vi "MacroGUI_MD.vi"() -> ()   [LabVIEW 2012]
doc: "SciScan 1.2 160622\nThis is the Macro User Interface which lets the user create a new macro, load an existing macro (from text file) and execute the macro (with feedback of execution)"
uses:
  Custom Controls and Typedefs/Available Operations Tree.ctl
  HFG/SubVIs/Master Slave messaging Flags.ctl
  HFG/Custom Controls and Typedefs/HB_Error Conditions Cluster.ctl
  HFG/Custom Controls and Typedefs/Heartbeat information cluster.ctl
  HFG/Custom Controls and Typedefs/Heartbeat Event Source.ctl
  Custom Controls/Heartbeat_States.ctl
  CommonResource VIs/Timing/Timing Indicator.ctl
  Custom Controls/Edit button with text.ctl
  Custom Controls and Typedefs/Timing Estimate Cluster.ctl
  Custom Controls and Typedefs/Confirm Settings.ctl
  Custom Controls and Typedefs/Delete Button.ctl
  Custom Controls and Typedefs/Cancel Settings.ctl
  Custom Controls and Typedefs/Load from PSM Button.ctl
  Custom Controls and Typedefs/Macro_MD_UI Control Refnums.ctl
  HFG/SubVIs/Heartbeat state manager Input VI names.ctl
  HFG/Custom Controls and Typedefs/HB Actionable Event.ctl
  CommonResource VIs/FormatTree&TableStyle_Commands.ctl
  <vilib>/Utility/miscctls.llb/LVRowAndColumnUnsignedTypeDef.ctl
  <vilib>/Utility/miscctls.llb/LVNodeAndColumnTypeDef.ctl
  Custom Controls and Typedefs/LOOP Control Cluster.ctl
  SubVIs/FGV_MacroCore_Commands.ctl
  CommonResource VIs/Timing/Timer Commands.ctl
  Common Macro VIs/Backup or Restore GFG Config Data_Commands.ctl
  HFG/Custom Controls and Typedefs/HFG Commands.ctl
  SubVIs/Update Scan Settings_Commands.ctl
  CommonResource VIs/UI Control and Indicator properties_Commands.ctl
  CommonResource VIs/Enable-Disable SCISCAN controls_Command.ctl
  Macro Rule/subVIs/MacroErrorsFGV_Commands.ctl
  image & display/Draw ROI on Line Scan Display Command.ctl
  SubVIs/MacroFileIO_Commands.ctl
  Macro Loop Manager Module/SubVIs/Macro Execution and Timing_Commands.ctl
  Custom Controls/scan mode main settings tab.ctl
  SubVIs/SCISCAN Image display to Enum_Commands.ctl
  GFG/GFG library.lvlib
  Custom Controls/Setting File Types.ctl
panel:
  in  "Refresh Timing":bool
  in  "Copy Button":bool
  in  "Get Positions":T1
  in  "Cancel Settings":T2
  in  "Delete Button":T3
  in  "Preview Macro":bool
  in  "Preview Cluster":T4
  in  "Edit Parameters":T5
  out "MacroFile\nPath":path caption="MacroFile\nPath*"
  in  "Confirm Settings":T6
  in  "Select Display":u16(ring) items=["Channel 1", "Channel 2", "Channel 3", "Channel 4", "all channels", "RGB overlay", "ROI", "arbitrary line scan"]
  out "Timing\n(approx.)":T7 caption="Timing\n(approx.)*" {"Elapsed" format="%<%H:%M:%S>t"; "Progress" scale=0.0..100.0; "Remaining" format="%<%H:%M:%S>t"; "Est. Time" format="%<%H:%M:%S>t"}
  out "Macro Error?":bool
  in  "Info":string[][](table)
  out "Paused/Wait for Trig":T8 caption="Paused" {"Elapsed" format="%<%H:%M:%S>t"; "Progress" scale=0.0..100.0; "Seconds" scale=0.0..60.0; "Remaining" format="%<%H:%M:%S>t"; "Set Time" format="%<%H:%M:%S>t"}
  out "Slave Completions Received":i32
  in  "stop 2":bool
  out "Master instr received":i32
  out "Slave conf received":i32
  out "Heartbeat information cluster":T9
  out "Error conditions Cluster":T12
  out "Master-Slave messaging Flags":T13={"Instruction available"=TRUE, "Slave action completed"=TRUE, "Slave Ready?"=FALSE}
  out "Current Index":i32
  in  "MacroTreeOperation":cluster{"Save Button":bool}
  in  "File Operation Cluster":T14
  in  "Parameters":string[][](table)
  in  "Execute Macro":bool
  in  "Available Actions":T15
  in  "Macro":string(tree)
  # "(hh:mm:ss)"
  # "(hh:mm:ss)"
  # "(hh:mm:ss)"
  # "(hh:mm:ss)"
  # "(hh:mm:ss)"
  # "(hh:mm:ss)"
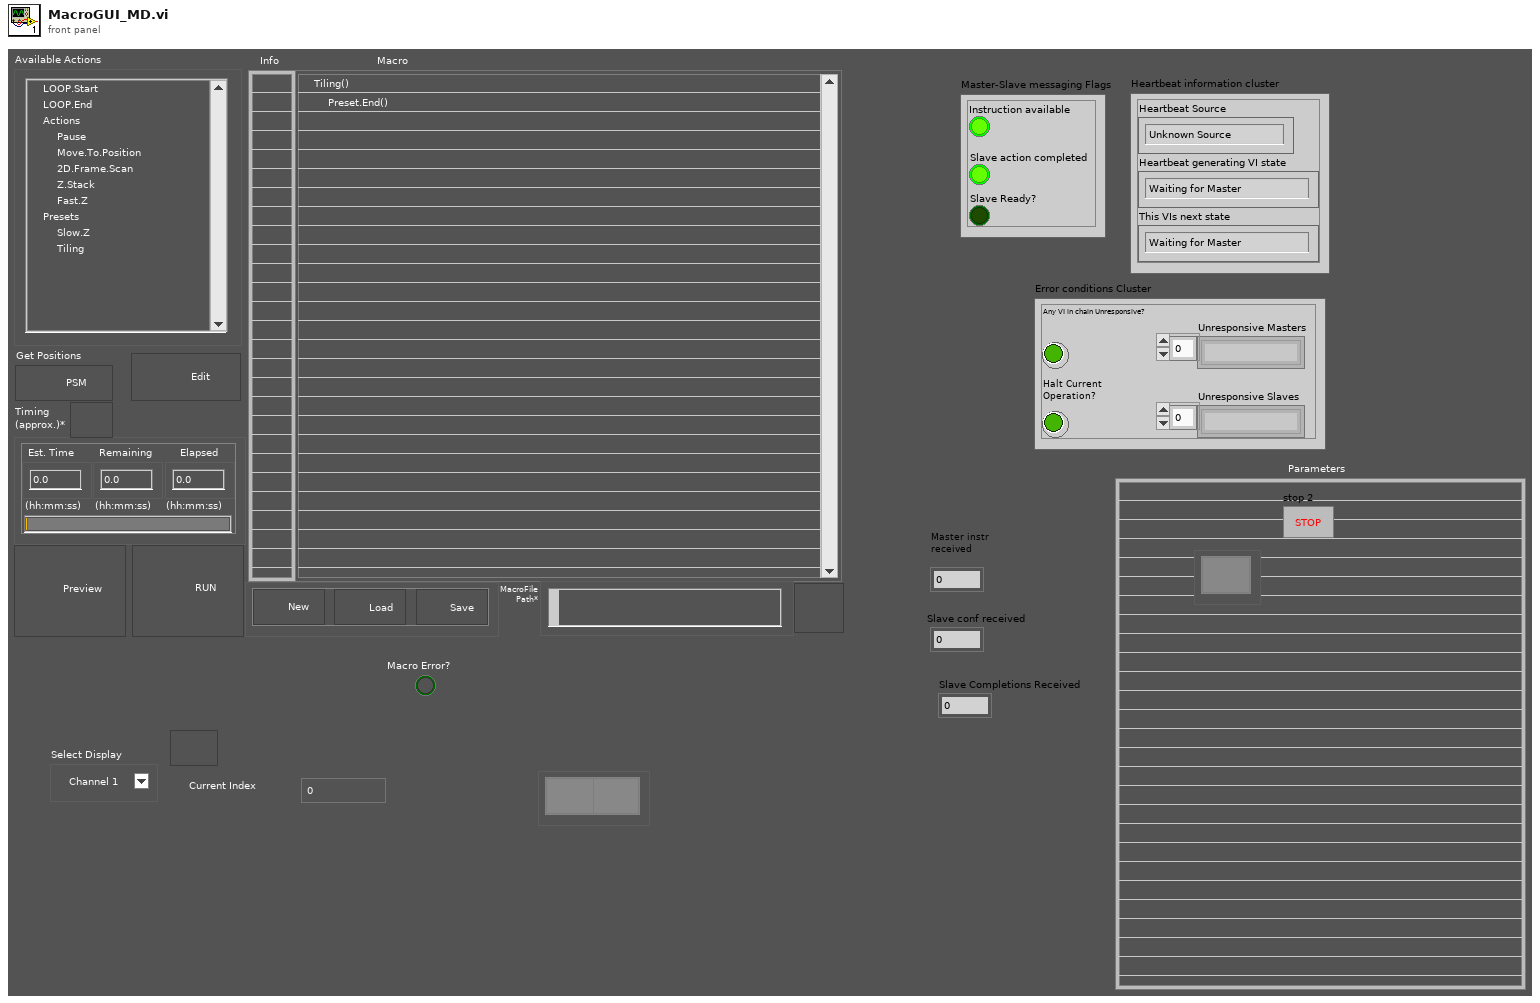
[diagram p1: front panel]
types:
  T1 = typedef "Load from PSM Button.ctl" = bool
  T2 = typedef "Cancel Settings.ctl" = bool
  T3 = typedef "Delete Button.ctl" = bool
  T4 = cluster{"Skip Forward Macro":bool, "Skip Back Macro":bool}
  T5 = typedef "Edit button with text.ctl" = bool
  T6 = typedef "Confirm Settings.ctl" = bool
  T7 = typedef "Timing Estimate Cluster.ctl" = cluster{"Est. Time":dbl, "Remaining":dbl, "Progress":u8, "Elapsed":dbl}
  T8 = typedef "Timing Indicator.ctl" = cluster{"Set Time":dbl, "Remaining":dbl, "Seconds":dbl, "Progress":u8, "Elapsed":dbl}
  T9 = typedef "Heartbeat information cluster.ctl" = cluster{"Heartbeat Source":T10, "Heartbeat generating VI state":T11, "This VIs next state":T11}
  T10 = typedef "Heartbeat Event Source.ctl" = enum16{"Unknown Source", "Timeout", "This VI", "Master", "Slave"}
  T11 = typedef "Heartbeat_States.ctl" = enum16{"Waiting for Master", "Instruction Issued", "Waiting for Slave Completion", "Completed", "Cancelled", "Failed", "Broken Link"}
  T12 = typedef "HB_Error Conditions Cluster.ctl" = cluster{"Any VI in chain Unresponsive?":bool, "Halt Current Operation?":bool, "Unresponsive Masters":string[], "Unresponsive Slaves":string[]}
  T13 = typedef "Master Slave messaging Flags.ctl" = cluster{"Instruction available":bool, "Slave action completed":bool, "Slave Ready?":bool}
  T14 = cluster{"Load Macro":bool, "Save Macro":bool, "New Macro":bool}
  T15 = typedef "Available Operations Tree.ctl" = string
  T16 = typedef "HB Actionable Event.ctl" = enum16{"Master instruction event", "Slave ready event", "Slave unavailable event", "Cancelled or Failed event", "Slave action complete event", "QUIT", "Broken Link", "Recovered from Broken Link"}
  T17 = typedef "Heartbeat state manager Input VI names.ctl" = cluster{"Current VI name":string, "Master VI Names":string[], "Slave VI Names":string[]}
  T18 = typedef "Macro_MD_UI Control Refnums.ctl" = cluster{"Avail. Operations":refnum<vi>, "Created Macro":refnum<vi>, "Load Macro":refnum<vi>, "Save Macro":refnum<vi>, "Params Table":refnum<vi>, "Delete":refnum<vi>, "Edit Button":refnum<vi>, "Execute Macro":refnum<vi>, "Info Tbl":refnum<vi>, "Execution Timing":refnum<vi>, "Select Display":refnum<vi>, "File Ops Cluster":refnum<vi>, "Paused/Waiting Trig":refnum<vi>, "Confirm":refnum<vi>, "New Macro":refnum<vi>, "Preview Macro":refnum<vi>, "Skip Forward":refnum<vi>, "Skip Back":refnum<vi>, "Macro File Path":refnum<vi>, "Main GUI Reference":refnum<vi>, "Cancel Settings":refnum<vi>, "Get Positions":refnum<vi>, "Copy":refnum<vi>, "Refresh Timing":refnum<vi>}
  T19 = typedef "LVRowAndColumnUnsignedTypeDef.ctl" = cluster{"Row":u32, "Column":u32}
  T20 = cluster{"user event out":refnum<user-event>, "HB Actionable Event":refnum<user-event>, "Index Values":refnum<user-event>, "Macro":refnum<vi>, "Parameters":refnum<vi>}
  T21 = typedef "Timer Commands.ctl" = enum16{"Clear All", "Start", "Pause", "Check Time"}
  T22 = typedef "FormatTree&TableStyle_Commands.ctl" = enum16{"Colour Row", "Uncolour Row", "Bold Row", "Unbold Row", "Clear", "UpdateVisibleRows"}
  T23 = typedef "LVNodeAndColumnTypeDef.ctl" = cluster{"Node":string, "Column":i32}
  T24 = typedef "FGV_MacroCore_Commands.ctl" = enum16{"Initialize", "Get Array", "Load macro from file", "Insert Item", "Insert at End", "Edit Parameter String", "Delete instruction", "Move Items", "Save", "SaveAs", "UpdateInfoTable", "Edit Settings File", "New Macro", "Read Temp File", "Delete Multiple"}
  T25 = enum16{"None", "Stacked", "Clockwise", "Counterclockwise"}
  T26 = typedef "SCISCAN Image display to Enum_Commands.ctl" = enum16{"Initialize", "SCISCAN disp to Enum", "Enum to SCISCAN disp"}
  T27 = typedef "Backup or Restore GFG Config Data_Commands.ctl" = enum16{"Backup", "Restore"}
  T28 = typedef "UI Control and Indicator properties_Commands.ctl" = enum16{"Enable", "Disable", "Disable and Grey", "Make Visible", "Make Invisible"}
  T29 = typedef "Update Scan Settings_Commands.ctl" = enum16{"Initiate Update", "Finalise Update"}
  T30 = typedef "HFG Commands.ctl" = enum16{"Set", "Get", "Initialize"}
  T31 = typedef "Enable-Disable SCISCAN controls_Command.ctl" = enum16{"Enable the items disabled earlier", "Disable", "Disable and Gray", "Enable all (except those in skip list)"}
  T32 = enum8{"Enabled", "Disabled", "Disabled and Grayed Out"}
  T33 = enum16{"Available Operations Tree", "Macro Tree"}
  T34 = typedef "MacroErrorsFGV_Commands.ctl" = enum16{"Initialize", "Get Error Array", "Set Error Array"}
  T35 = typedef "Draw ROI on Line Scan Display Command.ctl" = enum16{"Draw ROI from GFG", "Clear ROI"}
  T36 = typedef "Macro Execution and Timing_Commands.ctl" = enum16{"Initialize (Update FGV & Rst Idx)", "Run", "EstimateTime", "Preview", "Update Macro array (Idx Unchanged)", "Update Index", "Clear Timing Info"}
  T37 = typedef "MacroFileIO_Commands.ctl" = enum16{"Get Macro Info", "Initialize", "New Macro", "Load Macro", "Save", "Save in today's folder", "Update Settings File", "Add Settings File", "Delete Settings File", "Update Macro Text", "Save As", "Read Temp File"}
  T38 = enum32{"Invalid", "Standard", "Closed", "Hidden", "Minimized", "Maximized"}
  T39 = typedef "Setting File Types.ctl" = enum16{"2D.Frame.Scan.Settings", "2D.Line.Scan.Settings", "Z.Stack.Settings", "HW Settings", "Configuration Settings", "Unknown Settings", "Fast.Z.Settings"}
  T40 = typedef "scan mode main settings tab.ctl" = enum32{"2D frame", "2D line scan", "general settings", "Z Stack", "piezo"}
  T41 = typedef "LOOP Control Cluster.ctl" = cluster{"Index of LOOP.Start":i32, "Iteration Count Down":i32, "No of iterations (N)":i32}
  T42 = cluster{"Estimated Run time":dbl, "Step by step exec time":dbl[]}
  T43 = typedef "eventvkey.ctl" = enum16{"ASCII", "Enter", "Return", "Shift", "Ctrl", "Alt", "Cmd", "Opt", "Caps", "NumLock", "Clear", "Break", "Up", "Down", "Left", "Right", "Insert", "Delete", "Home", "End", "PageUp", "PageDown", "Escape", "Help", "Pause", "ScrollLock", "F1", "F2", "F3", "F4", "F5", "F6", "F7", "F8", "F9", "F10", "F11", "F12", "F13", "F14", "F15", "F16", "F17", "F18", "F19", "F20", "F21", "F22", "F23", "F24", "Play", "VolumeUp", "VolumeDown", "Mute", "Two Byte Char"}
  T44 = cluster{"data name":string, "drag data":variant}[]
  T45 = typedef "LVPoint32TypeDef.ctl" = cluster{"Horizontal":i32, "Vertical":i32}
  T46 = typedef "LVRowAndColumnTypeDef.ctl" = cluster{"Row":i32, "Column":i32}
  T47 = typedef "Macro Error Cluster.ctl" = cluster{"Error?":bool, "Description":string, "Warning?":bool}
  T48 = typedef "File Operation Status.ctl" = enum16{"Success", "File does not exist", "Cancelled by User", "Incorrect extension type"}
  T49 = typedef "Macro_Action_List.ctl" = enum16{"Unknown Command", "2D.Frame.Scan", "2D.Line.Scan", "Load.Settings.File", "Move.To.Position", "Pause", "Z.Stack", "LOOP.Start", "LOOP.End", "Record", "Fast.Z", "Generic", "Slow.Z", "Tiling", "Preset.End"}
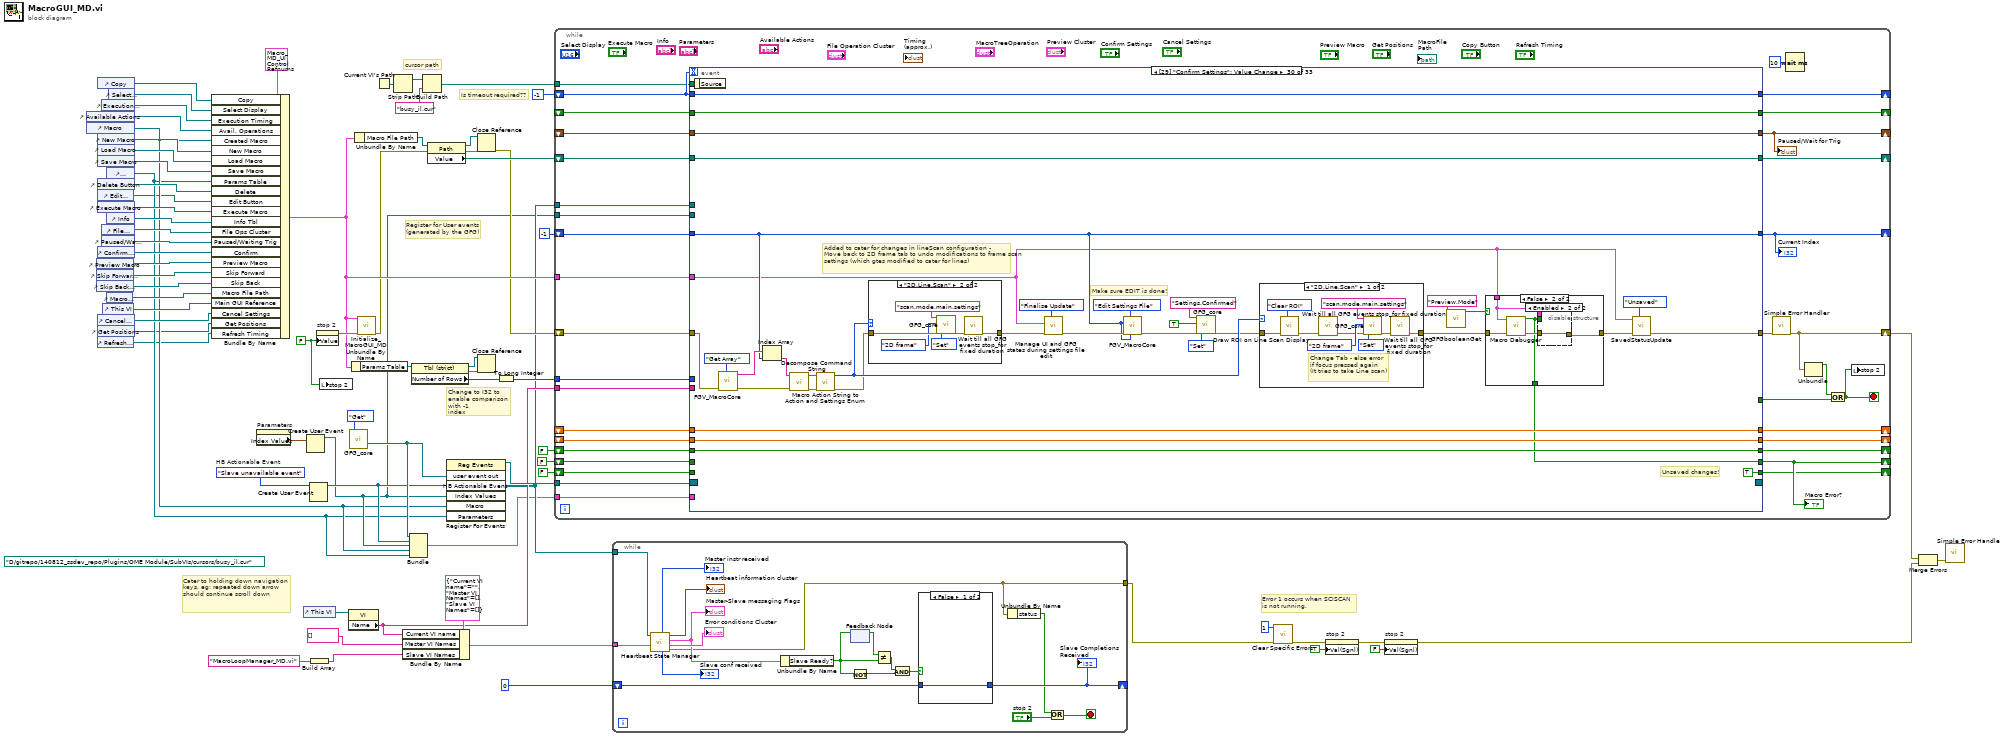
[diagram p0: block diagram]
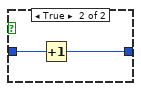
[diagram p2: hidden frame]
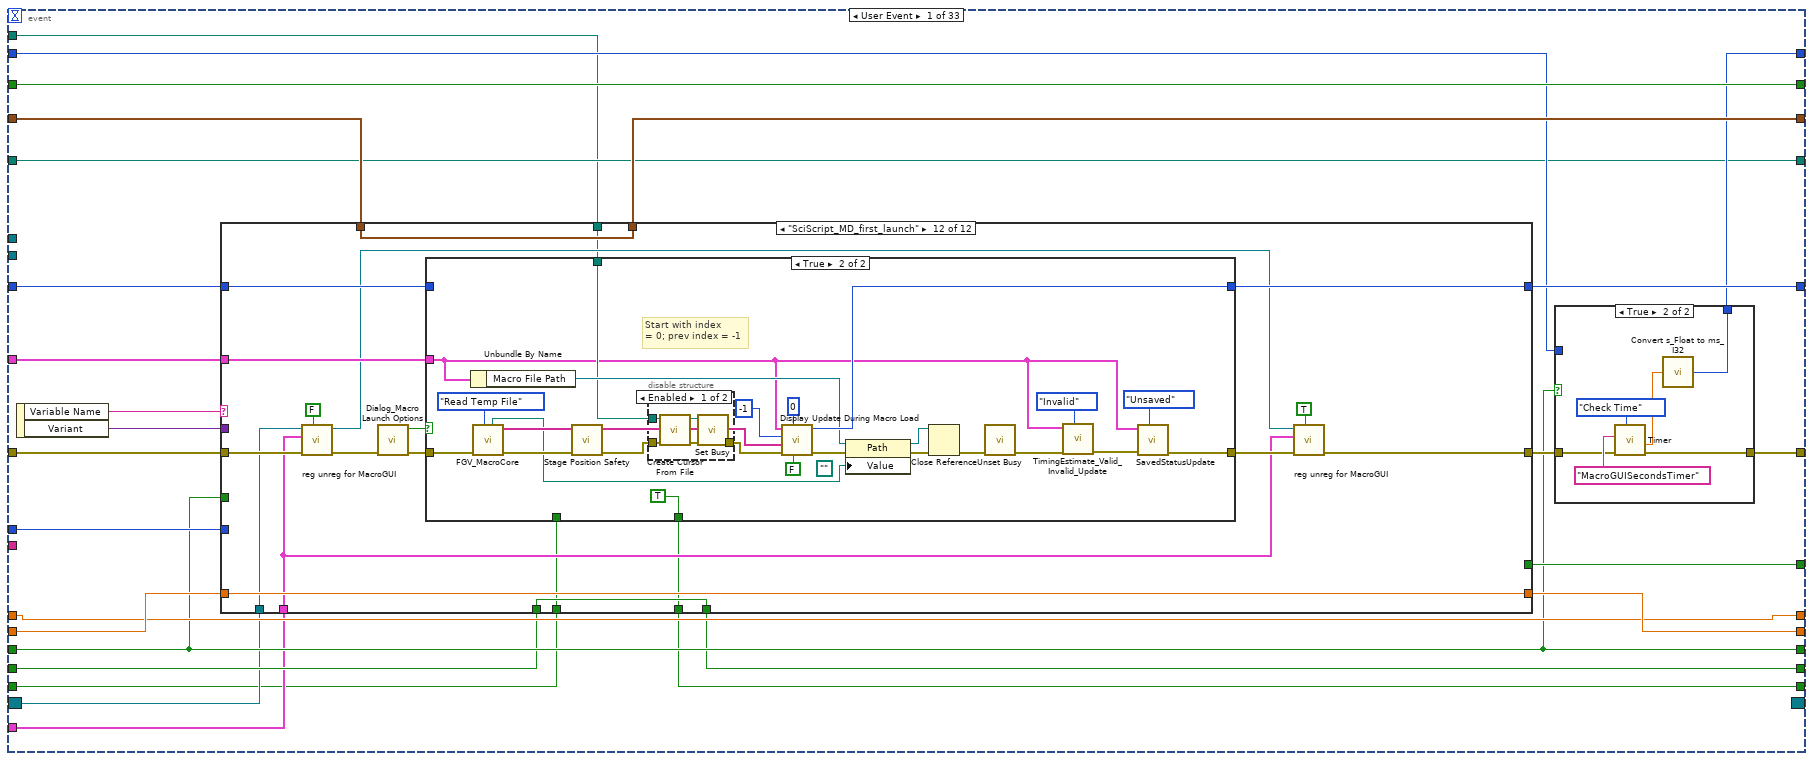
[diagram p3: hidden frame]
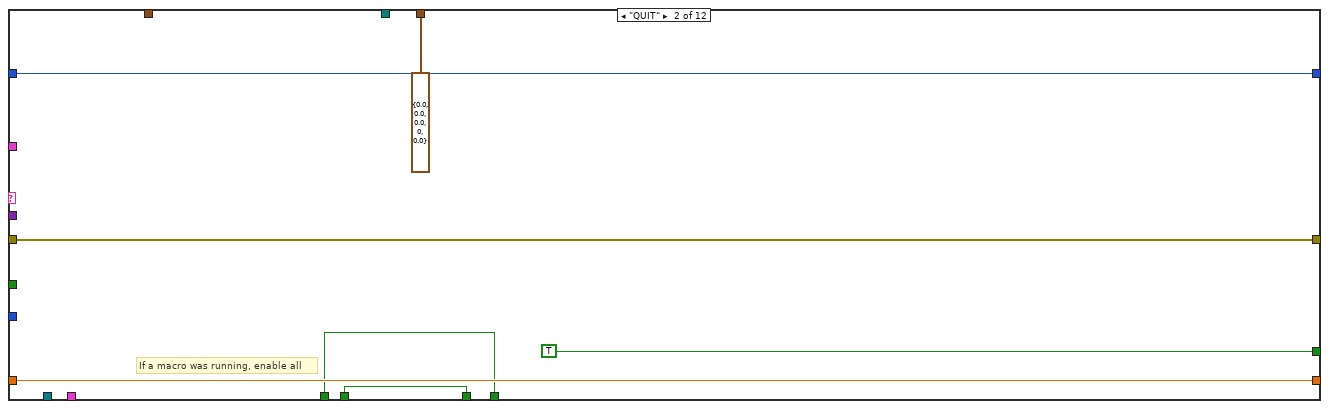
[diagram p6: hidden frame]
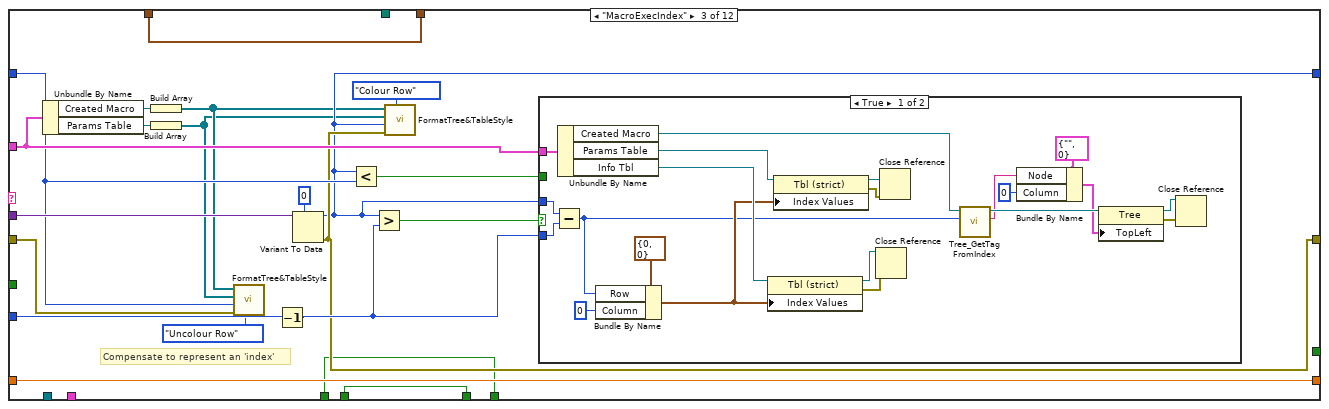
[diagram p7: hidden frame]
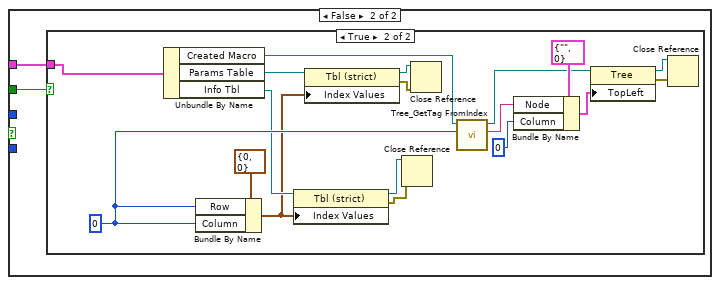
[diagram p8: hidden frame]
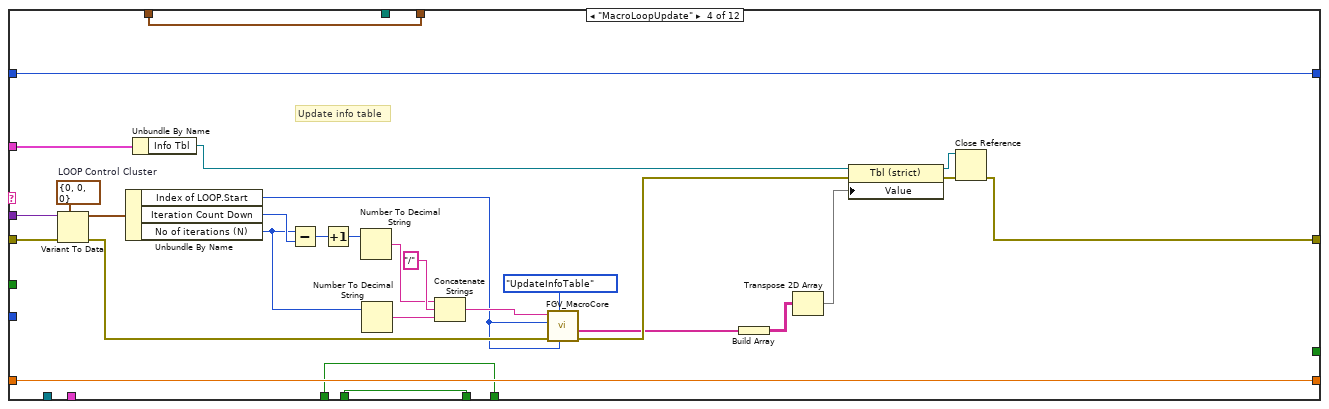
[diagram p10: hidden frame]
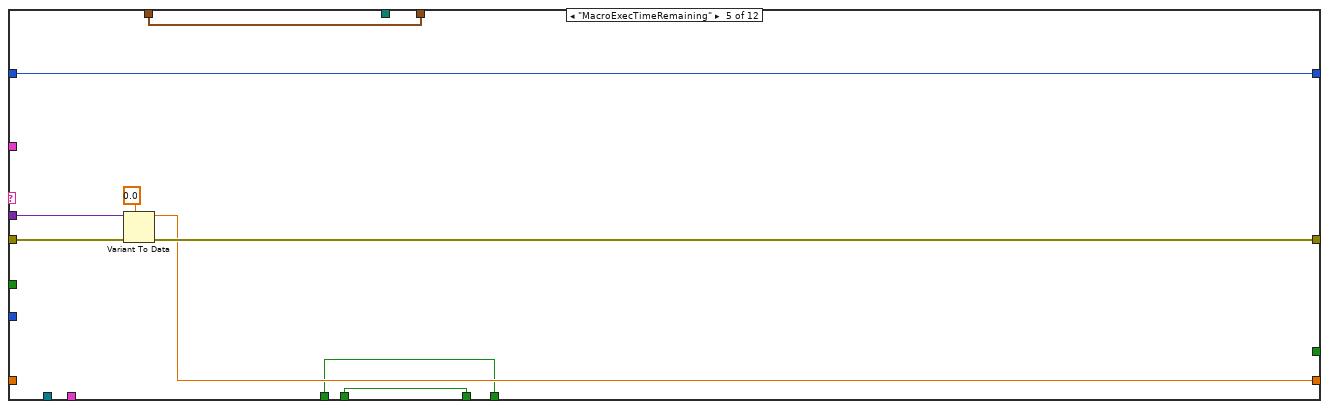
[diagram p11: hidden frame]
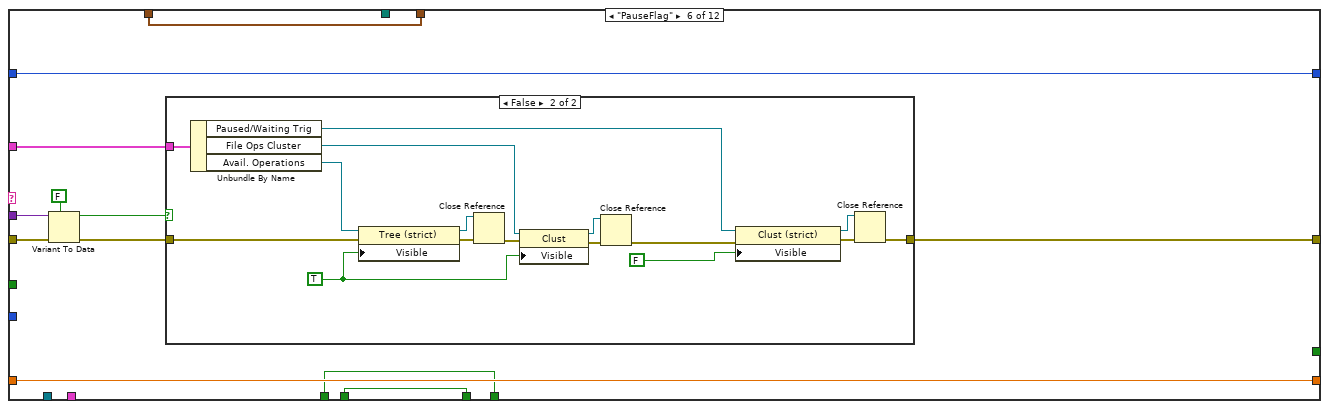
[diagram p12: hidden frame]
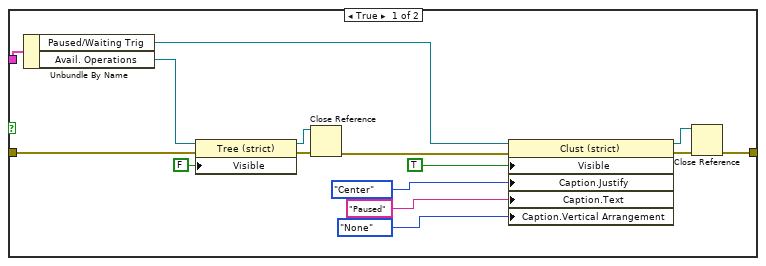
[diagram p13: hidden frame]
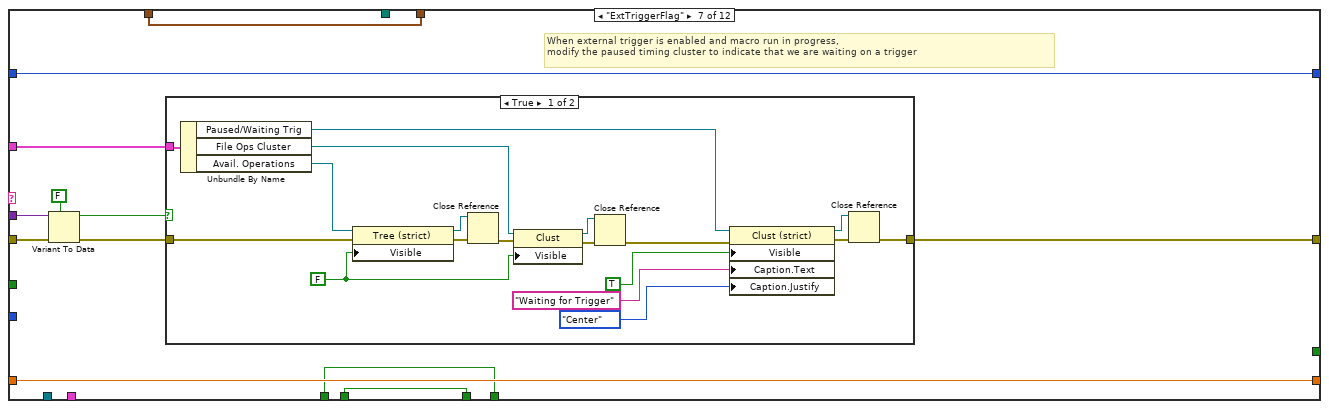
[diagram p14: hidden frame]
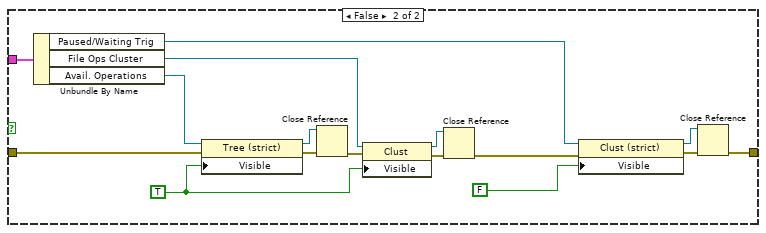
[diagram p15: hidden frame]
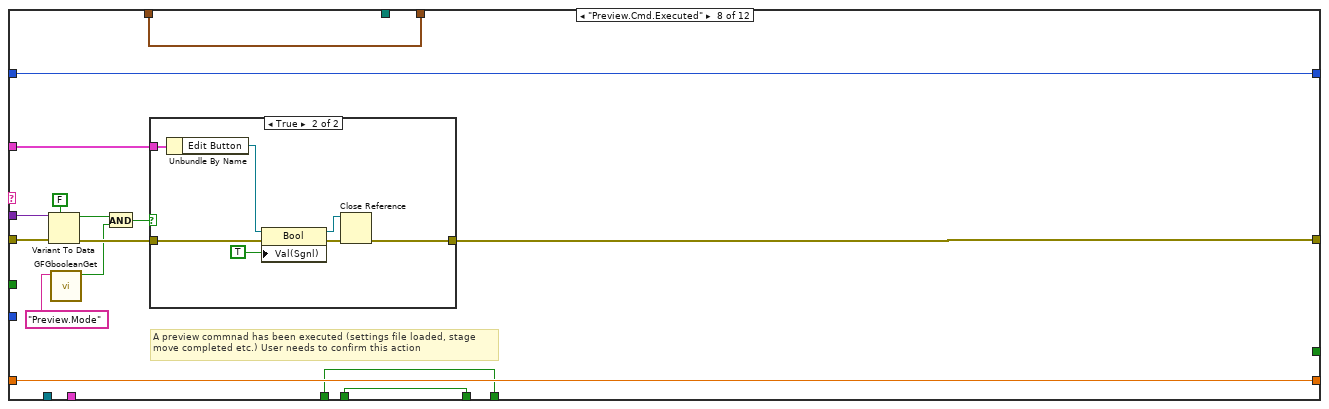
[diagram p16: hidden frame]
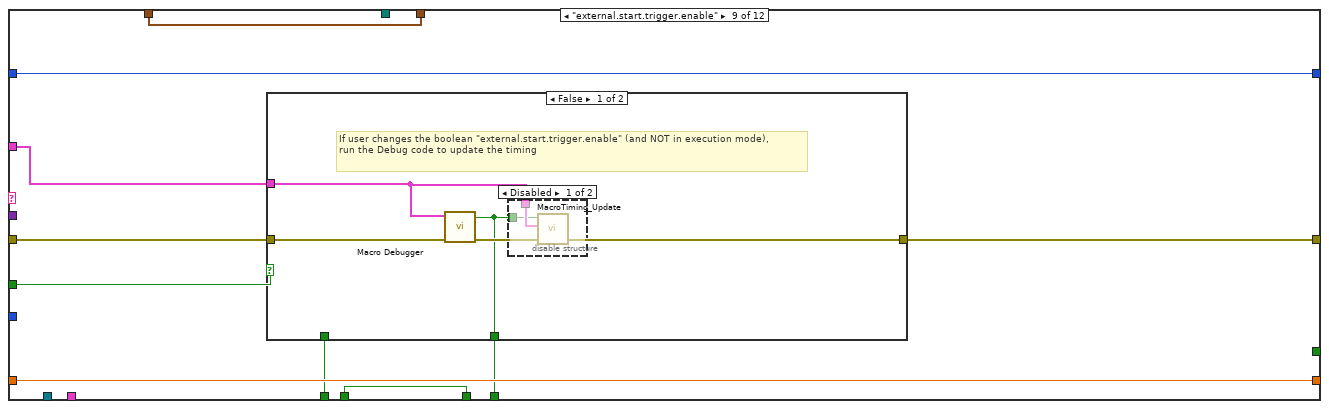
[diagram p18: hidden frame]
diagram:
  (unwired) path "D:/gitrepo/140812_ssdev_repo/Plugins/OME Module/SubVIs/cursors/busy_il.cur" ("cursor file")
  w65 = HB_Actionable_Event."Slave unavailable event"  # HB Actionable Event
  w51 = FALSE ("Execute Macro")
  # "cursor path"
  # "Cater to holding down navigation keys. eg: repeated down arrow should continue scroll down"
  # "Change to I32 to\nenable comparison with -1\nindex"
  # "Error 1 occurs when SCISCAN\nis not running."
  # "Is timeout required??"
  # "Register for User events\n(generated by the GFG)"
  n1 = control-ref of="Available Actions"() -> (w71:refnum<vi>)
  n2 = control-ref of="Macro"() -> (w13:refnum<vi>)
  n3 = control-ref of="Preview Macro"() -> (w33:refnum<vi>)
  n4 = control-ref of="Skip Forward Macro"() -> (w32:refnum<vi>)
  n5 = control-ref of="Skip Back Macro"() -> (w31:refnum<vi>)
  n6 = control-ref of="Edit Parameters"() -> (w2:refnum<vi>)
  n7 = control-ref of="Refresh Timing"() -> (w1:refnum<vi>)
  n8 = control-ref of="Copy"() -> (w7:refnum<vi>)
  n9 = control-ref of="New Macro"() -> (w34:refnum<vi>)
  n10 = control-ref of="Load Macro"() -> (w36:refnum<vi>)
  n11 = control-ref of="Save Macro"() -> (w72:refnum<vi>)
  n12 = control-ref of="Delete Button"() -> (w50:refnum<vi>)
  n13 = control-ref of="Execute Macro"() -> (w35:refnum<vi>)
  n14 = control-ref of="Confirm Settings"() -> (w37:refnum<vi>)
  n15 = control-ref of="Cancel Settings"() -> (w19:refnum<vi>)
  n16 = control-ref of="Get Positions"() -> (w10:refnum<vi>)
  n17 = control-ref of="Execution Timing"() -> (w42:refnum<vi>)
  n18 = control-ref of="File Operation Cluster"() -> (w40:refnum<vi>)
  n19 = control-ref of="Paused/Wait for Trig"() -> (w39:refnum<vi>)
  n20 = control-ref of="This VI"() -> (w20:refnum<vi>)
  n21 = control-ref of="Parameters"() -> (w12:refnum<vi>)
  n22 = control-ref of="Info"() -> (w45:refnum<vi>)
  n23 = control-ref of="Macro File Path"() -> (w30:refnum<vi>)
  n24 = control-ref of="Select Display"() -> (w41:refnum<vi>)
  n25 = Bundle By Name(cluster=T18 {"Avail. Operations"=refnum, "Created Macro"=refnum, "Load Macro"=refnum, "Save Macro"=refnum, "Params Table"=refnum, "Delete"=refnum, "Edit Button"=refnum, "Execute Macro"=refnum, "Info Tbl"=refnum, "Execution Timing"=refnum, "Select Display"=refnum, "File Ops Cluster"=refnum, "Paused/Waiting Trig"=refnum, "Confirm"=refnum, "New Macro"=refnum, "Preview Macro"=refnum, "Skip Forward"=refnum, "Skip Back"=refnum, "Macro File Path"=refnum, "Main GUI Reference"=refnum, "Cancel Settings"=refnum, "Get Positions"=refnum, "Copy"=refnum, "Refresh Timing"=refnum} ("UI control refnums"), "Copy"=w7, "Select Display"=w41, "Execution Timing"=w42, "Avail. Operations"=w71, "Created Macro"=w13, "New Macro"=w34, "Load Macro"=w36, "Save Macro"=w72, "Params Table"=w12, "Delete"=w50, "Edit Button"=w2, "Execute Macro"=w35, "Info Tbl"=w45, "File Ops Cluster"=w40, "Paused/Waiting Trig"=w39, "Confirm"=w37, "Preview Macro"=w33, "Skip Forward"=w32, "Skip Back"=w31, "Macro File Path"=w30, "Main GUI Reference"=w20, "Cancel Settings"=w19, "Get Positions"=w10, "Refresh Timing"=w1) -> (w29:T18)
  n26 = property on="Parameters" class="Tbl (strict)"() -> ("Index Values"=w49:T19)  [unwired: 2 in, 2 out]
  n27 = control-ref of="This VI"() -> (w67:refnum<vi>)
  n28 = Create User Event(user event datatype=w49) -> (user event=w14:refnum<user-event>)  [unwired: 1 in, 1 out]
  n29 = Create User Event(user event datatype=w65) -> (user event=w15:refnum<user-event>)  [unwired: 1 in, 1 out]
  n30 = Build Array("MacroLoopManager_MD.vi") -> (w22:string[])
  n31 = property on="stop 2" class="Bool (strict)"("Value"=w51) -> (error out=w38:errorcluster)  [unwired: 2 in, 1 out]
  n32 = local write "stop 2"(w51) -> ()
  n33 = property class="VI"(reference=w67) -> ("Name"=w64:string)  [unwired: 1 in, 2 out]
  n34 = call "GFG_core.vi"("Action"=enum16{"Init", "Set", "Get", "Clear"}."Get") -> ("user event out"=w16:refnum<user-event>)  [unwired: 12 in, 6 out]
  n35 = Unbundle By Name(w29) -> ("Params Table"=w46:refnum<vi>)
  n36 = Unbundle By Name(w29) -> ("Macro File Path"=w28:refnum<vi>)
  n37 = call "Initialize_MacroGUI_MD.vi"("Error In"=w38, "UI control refnums"=w29) -> ("Error Out"=w25:errorcluster)  [unwired: 7 in, 2 out]
  n38 = Current VI's Path() -> (path=w6:path)
  n39 = Strip Path(path=w6) -> (stripped path=w5:path)  [unwired: 1 out]
  n40 = Bundle By Name(cluster=T17 {"Current VI name"="", "Master VI Names"=[], "Slave VI Names"=[]} ("Heartbeat state manager Input VI names 2"), "Current VI name"=w64, "Master VI Names"=string[] [], "Slave VI Names"=w22) -> (w66:T17)
  n41 = Bundle("user event out"=w16, "HB Actionable Event"=w15, "Index Values"=w14, "Macro"=w13, "Parameters"=w12) -> (w11:T20)  [unwired: 1 in]
  n42 = property class="Tbl (strict)"(reference=w46) -> (reference out=w47:refnum<vi>, error out=w48:errorcluster, "Number of Rows"=w44:u32)  [unwired: 1 in]
  n43 = Build Path(base path=w5, name or relative path="busy_il.cur") -> (appended path=w3:path)
  n44 = property class="Path"(reference=w28, error in=w25) -> (reference out=w26:refnum<vi>, error out=w27:errorcluster, "Value"=w24:path)
  n45 = register-events(w16, w15, w14, w13, w12) -> (reference out=w70:refnum<event-registration>)  [unwired: 2 in, 1 out]
  n46 = Close Reference(reference=w26, error in (no error)=w27) -> (error out=w21:errorcluster)
  n47 = Close Reference(reference=w47, error in (no error)=w48) -> ()  [unwired: 1 out]
  n48 = To Long Integer(number=w44) -> (32bit integer=w43:i32)
  n49 = while {
    tunnel: w29 -> [w104]
    shift-right: [w80] -> w59
    shift-left: w21 -> [w89]
    shift-right: [w105] -> _
    shift-left: -1 ("New Index OUT") -> [w103]
    tunnel: w70 -> [w86]
    shift-right: [w102] -> _
    shift-left: -1 ("Index") -> [w101]
    tunnel: w64 -> [w100]
    shift-right: [w99] -> _
    shift-left: FALSE -> [w98]
    shift-right: [w97] -> _
    shift-left: _ -> [w96]
    shift-right: [w95] -> _
    shift-left: _ -> [w94]
    tunnel: w43 -> [w90]
    shift-right: [w92] -> _
    shift-left: FALSE ("Any Error?") -> [w91]
    shift-right: [w88] -> _
    shift-left: _ -> [w87]
    shift-right: [w85] -> _
    shift-left: _ -> [w84]
    shift-right: [w82] -> _
    shift-left: w24 -> [w83]
    tunnel: w15 -> [w79]
    tunnel: w14 -> [w78]
    tunnel: w11 -> [w77]
    shift-right: [w75] -> _
    shift-left: FALSE ("Any Error?") -> [w76]
    tunnel: w3 -> [w74]
    stop <- w93 stop-if-true
    n50 = event shown="[29] \"Confirm Settings\": Value Change" {
      selector: w86 -> [w112 _ _ _ _ _ _ _ _ _ _ _ _ _ w1038 w1064 _ _ _ _ _ _ _ w1619 w1652 _ _ w1859 _ _ w2253 _ _]
      dyn-events: [_ _ _ _ _ _ _ _ _ _ _ _ _ _ w1035 w1062 _ _ _ _ _ _ _ w1613 w1651 _ _ w1852 _ _ w2247 _ _] -> _
      timeout: w101 -> [_ _ _ _ _ _ _ _ _ _ _ _ _ _ _ _ _ _ _ _ _ _ _ _ _ _ _ _ _ _ _ _ _]
      tunnel: [w132 _ _ _ _ _ _ _ _ _ _ _ _ _ _ _ _ _ _ _ _ _ _ _ _ _ _ _ _ _ _ _ w2355] -> w108
      tunnel: w104 -> [w125 w481 _ w627 _ _ w805 w826 w846 w935 _ _ w1002 _ w1058 w1068 _ w1133 _ w1358 w1431 w1504 w1558 w1628 w1656 w1768 w1823 w1846 w2154 w2181 w2244 w2325 _]
      tunnel: w89 -> [w133 w482 w609 w629 w764 w793 w804 w844 w851 w930 w964 w976 w997 w1033 w1044 w1072 w1118 w1138 w1333 w1359 w1427 w1510 w1556 w1620 w1660 w1772 w1802 w1857 w2159 w2177 w2242 w2330 w2359]
      tunnel: [w121 w473 w608 w628 w764 w793 w811 w844 w853 w933 w964 w976 w994 w1033 w1039 w1081 w1114 w1139 w1332 w1357 w1428 w1511 w1560 w1612 w1658 w1769 w1797 w1853 w2158 w2183 w2246 w2316 w2359] -> w81
      tunnel: [w130 w485 w615 w625 w763 w792 w803 w843 w881 w928 w963 w975 w999 w1032 w1059 w1070 w1125 w1140 w1336 w1344 w1424 w1506 w1568 w1636 w1654 w1781 w1819 w1860 w2173 w2182 w2243 w2319 w2358] -> w105
      tunnel: w103 -> [w131 w485 w615 w626 w763 w792 w803 w843 w871 w927 w963 w975 w1000 w1032 w1059 w1069 w1125 w1140 w1336 w1344 w1426 w1505 w1568 w1636 w1655 w1781 w1820 w1842 w2173 w2182 w2240 w2319 w2358]
      tunnel: [w122 w475 w614 w634 w762 w779 w802 w836 w867 100 ("Index") -1 ("Index") w974 w981 -1 ("Index") w1053 w1094 w1124 w1130 w1335 w1354 w1438 w1509 w1567 w1635 w1668 w1780 w1815 w1869 w2172 w2208 w2266 w2337 w2357] -> w102
      tunnel: w101 -> [w123 w476 w614 w634 w762 w779 w802 w836 w867 _ _ w974 w981 _ w1053 w1094 w1124 _ w1335 w1347 w1438 w1509 w1567 w1635 w1668 w1780 w1815 w1869 w2172 w2208 w2266 w2337 w2357]
      tunnel: w100 -> [_ w480 _ _ _ _ _ _ _ _ _ _ _ _ _ _ _ w1136 _ _ _ _ _ _ w1659 _ _ _ _ _ _ _ _]
      tunnel: [w117 w477 w613 w624 w761 w778 w801 w835 w864 w924 w962 w973 w991 w1031 w1052 w1093 w1123 w1135 w1330 w1355 w1437 w1508 w1566 w1634 w1667 w1779 w1814 w1868 w2171 w2207 w2265 w2336 w2356] -> w99
      tunnel: w98 -> [w117 w483 w613 w624 w761 w778 w801 w835 w864 w924 w962 w973 w991 w1031 w1052 w1093 w1123 _ w1330 w1355 w1437 w1508 w1566 w1634 w1667 w1779 w1814 w1868 w2171 w2207 w2265 w2336 w2356]
      tunnel: [w129 w479 w612 w633 w760 w777 w800 w834 w866 w919 w961 w972 w990 w1030 w1051 w1092 w1122 w1134 w1331 w1360 w1436 w1503 w1565 w1633 w1666 w1778 w1813 w1867 w2170 w2206 w2264 w2335 w2354] -> w97
      tunnel: w96 -> [w128 w479 w612 w633 w760 w777 w800 w834 w866 w919 w961 w972 w990 w1030 w1051 w1092 w1122 w1134 w1331 w1360 w1436 w1503 w1565 w1633 w1666 w1778 w1813 w1867 w2170 w2206 w2264 w2335 w2354]
      tunnel: [w127 w478 w611 w632 w759 w776 w799 w833 w865 TRUE FALSE w971 FALSE FALSE w1050 w1091 w1121 w1132 w1329 w1346 w1435 w1502 w1564 w1632 w1665 w1777 w1812 w1866 w2169 w2205 w2263 w2334 w2353] -> w95
      tunnel: w94 -> [w127 w478 w611 w632 w759 w776 w799 w833 w865 _ _ w971 _ _ w1050 w1091 w1121 w1132 w1329 w1346 w1435 w1502 w1564 w1632 w1665 w1777 w1812 w1866 w2169 w2205 w2263 w2334 w2353]
      tunnel: [w114 w469 w610 w631 w758 w775 w798 w832 w859 w918 w960 w970 w982 w1027 w1049 w1090 w1120 w1131 w1328 w1356 w1430 w1500 w1563 w1631 w1664 w1776 w1809 w1864 w2164 w2190 w2255 w2323 w2352] -> w92
      tunnel: w91 -> [w115 w468 w610 w631 w758 w775 w798 w832 w863 w918 w960 w970 w982 w1027 w1049 w1090 w1120 w1131 w1328 w1356 w1429 w1499 w1563 w1631 w1664 w1776 w1810 w1865 w2164 _ w2256 _ w2352]
      tunnel: w90 -> [w126 _ _ _ _ _ _ _ _ _ _ _ _ _ _ _ _ _ _ w1345 _ _ _ _ _ _ _ _ _ _ _ _ _]
      tunnel: [w120 w472 w607 w623 w757 w774 w797 w831 w862 w917 w959 w969 w980 w1026 w1048 w1076 w1113 w1129 w1327 w1352 w1434 w1498 w1562 w1630 w1663 w1775 w1808 w1863 w2168 w2204 w2262 w2333 w2351] -> w88
      tunnel: w87 -> [w119 w472 w607 w623 w757 w774 w797 w831 w862 w917 w959 w969 w980 w1026 w1048 w1076 w1113 w1129 w1327 w1353 w1434 w1498 w1562 w1630 w1663 w1775 w1808 w1863 w2168 w2204 w2262 w2333 w2351]
      tunnel: [w118 w471 w606 w622 w756 w773 w796 w830 w861 w916 w958 w968 w979 w1025 w1047 w1075 w1112 w1127 w1326 w1351 w1433 w1497 w1561 w1629 w1662 w1774 w1807 w1862 w2167 w2203 w2261 w2332 w2350] -> w85
      tunnel: w84 -> [w118 w471 w606 w622 w756 w773 w796 w830 w861 w916 w958 w968 w979 w1025 w1047 w1075 w1112 _ w1326 w1350 w1433 w1497 w1561 w1629 w1662 w1774 w1807 w1862 w2167 w2203 w2261 w2332 w2350]
      tunnel: [w116 w470 w605 w621 w755 w772 w795 w829 w860 w915 w957 w967 w978 w1024 w1046 w1074 w1111 w1128 w1325 w1349 w1432 w1496 w1554 w1622 w1661 w1767 w1806 w1861 w2166 w2201 w2260 w2329 w2349] -> w82
      tunnel: w83 -> [w116 w470 w605 w621 w755 w772 w795 w829 w860 w915 w957 w967 w978 w1024 w1046 w1074 w1111 w1128 w1325 w1349 w1425 w1496 w1555 w1627 w1661 _ w1806 w1861 w2166 w2201 w2260 w2329 w2349]
      tunnel: w79 -> [_ _ _ _ _ _ _ _ _ _ _ _ _ _ _ _ _ _ _ _ _ _ _ _ _ _ _ _ _ _ _ _ _]
      tunnel: w78 -> [_ _ _ _ _ _ _ _ _ _ _ _ _ _ _ _ _ _ _ _ _ _ _ _ _ _ _ _ _ _ _ _ _]
      tunnel: w77 -> [w113 _ _ _ _ _ _ _ _ _ _ _ _ _ w1036 w1063 _ _ _ _ _ _ _ w1614 w1653 _ _ w1850 _ _ w2251 _ _]
      tunnel: w76 -> [w111 w467 w604 w620 w754 w771 w794 w828 _ w914 w956 w965 w977 w1023 w1034 w1061 w1110 w1126 w1324 w1348 w1421 w1494 w1559 w1610 w1650 w1765 w1805 w1849 w2165 _ w2245 w2310 w2348]
      tunnel: [w110 w467 w604 w620 w754 w771 w794 w828 TRUE ("Any Error?") w914 w956 w965 w977 w1023 w1034 w1061 w1110 w1126 w1324 w1348 w1421 w1494 w1559 w1611 w1650 w1766 w1804 w1848 w2165 TRUE ("Any Error?") w2245 w2310 w2348] -> w75
      tunnel: w74 -> [w109 _ _ _ _ _ _ _ w852 _ _ _ _ _ _ _ _ _ _ _ _ w1493 _ _ _ _ w1799 _ w2160 _ _ _ _]
      event User Event {
        n51 = event-data() -> ("Variable Name"=w135:string, "Variant"=w134:variant)  [unwired: 1 in]
        n52 = case shown="\"SciScript_MD_first_launch\"" w135 {
          tunnel: w134 -> [_ _ w177 w244 w255 w265 w308 w354 _ _ _ _]
          tunnel: w133 -> [w149 w153 w170 w245 w253 w266 w309 w353 w375 w397 w403 w419]
          tunnel: [w149 w153 w165 w229 w252 w262 w305 w356 w373 w391 w402 w409] -> w124
          tunnel: [_ TRUE _ _ _ _ _ _ _ _ _ _] -> w132
          tunnel: w131 -> [w148 w155 w167 w247 w256 w268 w311 w360 w378 w398 w405 w423]
          tunnel: [w148 w155 w164 w247 w256 w268 w311 w360 w378 w398 w405 w422] -> w130
          tunnel: [w147 T8 {"Set Time"=0.0, "Remaining"=0.0, "Seconds"=0.0, "Progress"=0, "Elapsed"=0.0} ("Paused") w175 w228 w250 w261 w304 w358 w372 w390 w404 w426] -> w129
          tunnel: w128 -> [w147 _ w175 w228 w250 w261 w304 w358 w372 _ w404 w426]
          tunnel: w126 -> [_ _ w172 _ _ _ _ _ _ _ _ _]
          tunnel: w125 -> [_ _ w168 w242 _ w259 w302 w357 w374 _ _ w421]
          tunnel: [w146 w152 w159 w224 w251 w260 w303 w359 w377 w389 w401 w428] -> w120
          tunnel: w119 -> [w146 w152 w159 w224 _ w260 w303 w359 w377 w389 w401 w428]
          tunnel: w117 -> [_ _ _ _ _ _ _ _ w376 _ _ _]
          tunnel: w115 -> [w145 w151 w158 w223 w249 w258 w301 w347 w371 w388 w400 w427]
          tunnel: [w145 w151 w158 w223 w249 w258 w301 w347 w370 w388 w400 w427] -> w114
          tunnel: w113 -> [_ _ _ _ _ _ _ _ _ _ _ w413]
          tunnel: w112 -> [_ _ _ _ _ _ _ _ _ _ _ w415]
          tunnel: w111 -> [w144 w150 w157 w221 w248 w257 w300 w346 w369 w387 w399 w412]
          tunnel: [w144 w150 w157 w221 w248 w257 w300 w346 w369 w387 w399 w411] -> w110
          tunnel: w109 -> [_ _ _ _ _ _ _ _ _ _ _ w410]
          frame Default {
          }
          frame "QUIT" {
            # "If a macro was running, enable all"
          }
          frame "MacroExecIndex" {
            # "Compensate to represent an 'index'"
            n53 = Unbundle By Name(w168) -> ("Created Macro"=w162:refnum<vi>, "Params Table"=w163:refnum<vi>)
            n54 = Build Array(w162) -> (w161:refnum<vi>[])
            n55 = Build Array(w163) -> (w160:refnum<vi>[])
            n56 = call "FormatTree&TableStyle.vi"("Format Command"=FormatTree&TableStyle_Commands."Uncolour Row", "Error In"=w170, "Row Index"=w167, "Array of Table references"=w160, "Array of Tree references"=w161) -> ()  [unwired: 6 in, 1 out]
            n57 = Decrement(x=w172) -> (x-1=w171:i32)
            n58 = Variant To Data(type=0 ("Index"), Variant=w177) -> (data=w164:i32, error out=w165:errorcluster)  [unwired: 1 in]
            n59 = Less?(x=w164, y=w167) -> (x < y?=w173:bool)
            n60 = Greater?(x=w164, y=w171) -> (0:w174:bool)
            n61 = call "FormatTree&TableStyle.vi"("Format Command"=FormatTree&TableStyle_Commands."Colour Row", "Error In"=w165, "Row Index"=w164, "Array of Table references"=w160, "Array of Tree references"=w161) -> ()  [unwired: 6 in, 1 out]
            n62 = case shown="True" w174 {
              tunnel: w164 -> [w197 _]
              tunnel: w171 -> [w196 _]
              tunnel: w168 -> [w198 w200]
              tunnel: w173 -> [_ w199]
              frame True {
                n63 = Subtract(x=w197, y=w196) -> (x-y=w178:i32)
                n64 = Unbundle By Name(w198) -> ("Created Macro"=w191:refnum<vi>, "Params Table"=w195:refnum<vi>, "Info Tbl"=w182:refnum<vi>)
                n65 = Bundle By Name(cluster=T19 {"Row"=0, "Column"=0} ("Index Values"), "Row"=w178, "Column"=u32 0) -> (w181:T19)
                n66 = property class="Tbl (strict)"(reference=w182, "Index Values"=w181) -> (reference out=w179:refnum<vi>, error out=w180:errorcluster)  [unwired: 1 in]
                n67 = property class="Tbl (strict)"(reference=w195, "Index Values"=w181) -> (reference out=w192:refnum<vi>, error out=w193:errorcluster)  [unwired: 1 in]
                n68 = Close Reference(reference=w179, error in (no error)=w180) -> ()  [unwired: 1 out]
                n69 = Close Reference(reference=w192, error in (no error)=w193) -> ()  [unwired: 1 out]
                n70 = call "Tree_GetTag FromIndex.vi"("Index IN"=w178, "Tree Refnum IN"=w191) -> ("Tag OUT"=w188:string, "Tree Refnum OUT"=w189:refnum<vi>)  [unwired: 7 in, 1 out]
                n71 = Bundle By Name(cluster=T23 {"Node"="", "Column"=0} ("Top Left Visible Cell"), "Node"=w188, "Column"=0) -> (w186:T23)
                n72 = property class="Tree"(reference=w189, "TopLeft"=w186) -> (reference out=w184:refnum<vi>, error out=w185:errorcluster)  [unwired: 1 in]
                n73 = Close Reference(reference=w184, error in (no error)=w185) -> ()  [unwired: 1 out]
              }
              frame False {
                n74 = case shown="True" w199 {
                  tunnel: w200 -> [_ w218]
                  frame False {
                  }
                  frame True {
                    w205 = u32 0 ("Column")
                    n75 = Unbundle By Name(w218) -> ("Created Macro"=w213:refnum<vi>, "Params Table"=w217:refnum<vi>, "Info Tbl"=w203:refnum<vi>)
                    n76 = Bundle By Name(cluster=T19 {"Row"=0, "Column"=0} ("Index Values"), "Row"=w205, "Column"=w205) -> (w202:T19)
                    n77 = property class="Tbl (strict)"(reference=w203, "Index Values"=w202) -> (reference out=w201:refnum<vi>, error out=w204:errorcluster)  [unwired: 1 in]
                    n78 = property class="Tbl (strict)"(reference=w217, "Index Values"=w202) -> (reference out=w214:refnum<vi>, error out=w215:errorcluster)  [unwired: 1 in]
                    n79 = Close Reference(reference=w201, error in (no error)=w204) -> ()  [unwired: 1 out]
                    n80 = Close Reference(reference=w214, error in (no error)=w215) -> ()  [unwired: 1 out]
                    n81 = call "Tree_GetTag FromIndex.vi"("Index IN"=w205, "Tree Refnum IN"=w213) -> ("Tag OUT"=w210:string, "Tree Refnum OUT"=w211:refnum<vi>)  [unwired: 7 in, 1 out]
                    n82 = Bundle By Name(cluster=T23 {"Node"="", "Column"=0} ("Top Left Visible Cell"), "Node"=w210, "Column"=0) -> (w208:T23)
                    n83 = property class="Tree"(reference=w211, "TopLeft"=w208) -> (reference out=w206:refnum<vi>, error out=w207:errorcluster)  [unwired: 1 in]
                    n84 = Close Reference(reference=w206, error in (no error)=w207) -> ()  [unwired: 1 out]
                  }
                }
              }
            }
          }
          frame "MacroLoopUpdate" {
            w246 = T41 {"Index of LOOP.Start"=0, "Iteration Count Down"=0, "No of iterations (N)"=0}  # LOOP Control Cluster
            # "Update info table"
            n85 = Variant To Data(error in=w245, type=w246, Variant=w244) -> (data=w243:T41, error out=w233:errorcluster)
            n86 = Unbundle By Name(w243) -> ("Index of LOOP.Start"=w222:i32, "Iteration Count Down"=w241:i32, "No of iterations (N)"=w238:i32)
            n87 = Unbundle By Name(w242) -> ("Info Tbl"=w234:refnum<vi>)
            n88 = Subtract(x=w238, y=w241) -> (x-y=w219:i32)
            n89 = Increment(x=w219) -> (x+1=w220:i32)
            n90 = Number To Decimal String(number=w220) -> (decimal integer string=w237:string)  [unwired: 1 in]
            n91 = Number To Decimal String(number=w238) -> (decimal integer string=w239:string)  [unwired: 1 in]
            n92 = Concatenate Strings(w237, "/" ("string"), w239) -> (w235:string)
            n93 = call "FGV_MacroCore.vi"("Final Index"=w222, "MacroFGV_Commands"=FGV_MacroCore_Commands."UpdateInfoTable", "Error In"=w233, "Start Index"=w222, "Macro Command or Info (String)"=w235) -> ("Error Out"=w232:errorcluster, "Info Table Array"=w227:string[])  [unwired: 2 in, 3 out]
            n94 = Build Array(w227) -> (w226:string[][])
            n95 = Transpose 2D Array(2D array=w226) -> (transposed array=w225:string[][])
            n96 = property class="Tbl (strict)"(reference=w234, error in=w232, "Value"=w225) -> (reference out=w230:refnum<vi>, error out=w231:errorcluster)
            n97 = Close Reference(reference=w230, error in (no error)=w231) -> (error out=w229:errorcluster)
          }
          frame "MacroExecTimeRemaining" {
            n98 = Variant To Data(error in=w253, type=0.0, Variant=w255) -> (data=w251:dbl, error out=w252:errorcluster)
          }
          frame "PauseFlag" {
            n99 = Variant To Data(error in=w266, type=FALSE, Variant=w265) -> (data=w264:bool, error out=w263:errorcluster)
            n100 = case shown="False" w264 {
              tunnel: w263 -> [w280 w295]
              tunnel: [w273 w286] -> w262
              tunnel: w259 -> [w283 w299]
              frame True {
                n101 = Unbundle By Name(w283) -> ("Paused/Waiting Trig"=w281:refnum<vi>, "Avail. Operations"=w282:refnum<vi>)
                n102 = property class="Tree (strict)"(reference=w282, error in=w280, "Visible"=FALSE) -> (reference out=w278:refnum<vi>, error out=w279:errorcluster)
                n103 = Close Reference(reference=w278, error in (no error)=w279) -> (error out=w269:errorcluster)
                n104 = property class="Clust (strict)"(reference=w281, error in=w269, "Visible"=TRUE, "Caption.Justify"=enum16{"Left", "Center", "Right"}."Center" ("Caption.Justification"), "Caption.Text"="Paused", "Caption.Vertical Arrangement"=T25."None") -> (reference out=w276:refnum<vi>, error out=w277:errorcluster)
                n105 = Close Reference(reference=w276, error in (no error)=w277) -> (error out=w273:errorcluster)
              }
              frame False {
                w287 = TRUE ("Visible")
                n106 = Unbundle By Name(w299) -> ("Paused/Waiting Trig"=w296:refnum<vi>, "File Ops Cluster"=w297:refnum<vi>, "Avail. Operations"=w298:refnum<vi>)
                n107 = property class="Tree (strict)"(reference=w298, error in=w295, "Visible"=w287) -> (reference out=w293:refnum<vi>, error out=w294:errorcluster)
                n108 = Close Reference(reference=w293, error in (no error)=w294) -> (error out=w284:errorcluster)
                n109 = property class="Clust"(reference=w297, error in=w284, "Visible"=w287) -> (reference out=w291:refnum<vi>, error out=w292:errorcluster)
                n110 = Close Reference(reference=w291, error in (no error)=w292) -> (error out=w285:errorcluster)
                n111 = property class="Clust (strict)"(reference=w296, error in=w285, "Visible"=FALSE) -> (reference out=w289:refnum<vi>, error out=w290:errorcluster)
                n112 = Close Reference(reference=w289, error in (no error)=w290) -> (error out=w286:errorcluster)
              }
            }
          }
          frame "ExtTriggerFlag" {
            # "When external trigger is enabled and macro run in progress,\nmodify the paused timing cluster to indicate that we are waiting on a trigger"
            n113 = Variant To Data(error in=w309, type=FALSE, Variant=w308) -> (data=w307:bool, error out=w306:errorcluster)
            n114 = case shown="True" w307 {
              tunnel: w306 -> [w325 w341]
              tunnel: [w316 w332] -> w305
              tunnel: w302 -> [w329 w345]
              frame True {
                w317 = FALSE ("Visible")
                n115 = Unbundle By Name(w329) -> ("Paused/Waiting Trig"=w326:refnum<vi>, "File Ops Cluster"=w327:refnum<vi>, "Avail. Operations"=w328:refnum<vi>)
                n116 = property class="Tree (strict)"(reference=w328, error in=w325, "Visible"=w317) -> (reference out=w323:refnum<vi>, error out=w324:errorcluster)
                n117 = Close Reference(reference=w323, error in (no error)=w324) -> (error out=w314:errorcluster)
                n118 = property class="Clust"(reference=w327, error in=w314, "Visible"=w317) -> (reference out=w321:refnum<vi>, error out=w322:errorcluster)
                n119 = Close Reference(reference=w321, error in (no error)=w322) -> (error out=w315:errorcluster)
                n120 = property class="Clust (strict)"(reference=w326, error in=w315, "Visible"=TRUE, "Caption.Text"="Waiting for Trigger", "Caption.Justify"=enum16{"Left", "Center", "Right"}."Center" ("Caption.Justification")) -> (reference out=w319:refnum<vi>, error out=w320:errorcluster)
                n121 = Close Reference(reference=w319, error in (no error)=w320) -> (error out=w316:errorcluster)
              }
              frame False {
                w333 = TRUE ("Visible")
                n122 = Unbundle By Name(w345) -> ("Paused/Waiting Trig"=w342:refnum<vi>, "File Ops Cluster"=w343:refnum<vi>, "Avail. Operations"=w344:refnum<vi>)
                n123 = property class="Tree (strict)"(reference=w344, error in=w341, "Visible"=w333) -> (reference out=w339:refnum<vi>, error out=w340:errorcluster)
                n124 = Close Reference(reference=w339, error in (no error)=w340) -> (error out=w330:errorcluster)
                n125 = property class="Clust"(reference=w343, error in=w330, "Visible"=w333) -> (reference out=w337:refnum<vi>, error out=w338:errorcluster)
                n126 = Close Reference(reference=w337, error in (no error)=w338) -> (error out=w331:errorcluster)
                n127 = property class="Clust (strict)"(reference=w342, error in=w331, "Visible"=FALSE) -> (reference out=w335:refnum<vi>, error out=w336:errorcluster)
                n128 = Close Reference(reference=w335, error in (no error)=w336) -> (error out=w332:errorcluster)
              }
            }
          }
          frame "Preview.Cmd.Executed" {
            # "A preview commnad has been executed (settings file loaded, stage move completed etc.) User needs to confirm this action"
            n129 = Variant To Data(error in=w353, type=FALSE, Variant=w354) -> (data=w349:bool, error out=w352:errorcluster)
            n130 = call "GFGbooleanGet.vi"("Variable Name in"="Preview.Mode") -> ("Boolean Value OUT"=w350:bool)  [unwired: 9 in, 1 out]
            n131 = And(x=w349, y=w350) -> (x .and. y?=w348:bool)
            n132 = case shown="True" w348 {
              tunnel: w357 -> [_ w368]
              tunnel: [w361 w363] -> w356
              tunnel: w352 -> [w361 w362]
              frame False {
              }
              frame True {
                n133 = Unbundle By Name(w368) -> ("Edit Button"=w367:refnum<vi>)
                n134 = property class="Bool"(reference=w367, error in=w362, "Val(Sgnl)"=TRUE) -> (reference out=w364:refnum<vi>, error out=w365:errorcluster)
                n135 = Close Reference(reference=w364, error in (no error)=w365) -> (error out=w363:errorcluster)
              }
            }
          }
          frame "external.start.trigger.enable" {
            n136 = case shown="False" w376 {
              tunnel: w375 -> [w382 w386]
              tunnel: w374 -> [w380 _]
              tunnel: [w381 w386] -> w373
              tunnel: w371 -> [_ w385]
              tunnel: [w379 w385] -> w370
              frame False {
                # "If user changes the boolean \"external.start.trigger.enable\" (and NOT in execution mode), \nrun the Debug code to update the timing"
                n137 = call "Macro Debugger.vi"("Error In"=w382, "UI control refnums"=w380) -> ("Error Out"=w381:errorcluster, "Any Error?"=w379:bool)  [unwired: 8 in]
                n138 = disable-structure shown="Disabled" {
                  disable-tunnel: w380 -> [w384 _]
                  disable-tunnel: w379 -> [w383 _]
                  frame Disabled {
                    n139 = call "MacroTiming_Update.vi"("UI control refnums"=w384, "Macro Error IN?"=w383) -> ()  [unwired: 9 in, 1 out]
                  }
                  frame Enabled {
                  }
                }
              }
              frame True {
                # "During Macro Execution, do nothing"
              }
            }
          }
          frame "PauseTime" {
            n140 = call "GFG_core.vi"("Variable Name in"="PauseTime", "error in (no error)"=w397, "Action"=enum16{"Init", "Set", "Get", "Clear"}."Get") -> ("Variant Out"=w393:variant, "error out"=w392:errorcluster)  [unwired: 10 in, 5 out]
            n141 = Variant To Data(error in=w392, type=T8 {"Set Time"=0.0, "Remaining"=0.0, "Seconds"=0.0, "Progress"=0, "Elapsed"=0.0} ("Paused"), Variant=w393) -> (data=w390:T8, error out=w391:errorcluster)
          }
          frame "MAIN.Image.panels.", "MAIN.Image.panels.reso." {
            n142 = disable-structure shown="Disabled" {
              disable-tunnel: w403 -> [w408 _]
              disable-tunnel: [w406 _] -> w402
              frame Disabled {
                n143 = call "SCISCAN Image display TO Enum .vi"("SCISCAN Image display_to_Enum_Commands"=SCISCAN_Image_display_to_Enum_Commands."SCISCAN disp to Enum", "Error In"=w408) -> ("Error Out"=w406:errorcluster)  [unwired: 9 in]
              }
              frame Enabled {
              }
            }
          }
          frame "SciScript_MD_first_launch" {
            n144 = call "reg unreg for MacroGUI.vi"("T for reg, F for unreg"=FALSE, "error in (no error)"=w419, "event cluster"=w413, "Event Registration Refnum"=w415) -> ("error out"=w418:errorcluster, "Event Registration Refnum Out"=w414:refnum<event-registration>)  [unwired: 6 in]
            n145 = call "Dialog_Macro Launch Options.vi"("error in (no error)"=w418) -> ("error out"=w424:errorcluster, "Load Temp?"=w425:bool)  [unwired: 9 in]
            n146 = case shown="True" w425 {
              tunnel: w424 -> [w431 w460]
              tunnel: w423 -> [w436 _]
              tunnel: [w436 w456] -> w422
              tunnel: [w433 w445] -> w416
              tunnel: w421 -> [w430 w437]
              tunnel: w412 -> [w435 _]
              tunnel: [w435 TRUE] -> w411
              tunnel: w410 -> [_ w442]
              frame False {
                n147 = call "TimingEstimate_Valid_Invalid_Update.vi"("Command"=enum16{"Valid", "Invalid"}."Valid", "error in (no error)"=w431, "UI control refnums"=w430) -> ("error out"=w429:errorcluster)  [unwired: 8 in]
                n148 = call "SavedStatusUpdate.vi"("Options"=enum16{"Unsaved", "Saved"}."Saved", "error in (no error)"=w429, "UI control refnums"=w430) -> ("error out"=w433:errorcluster)  [unwired: 8 in]
              }
              frame True {
                (unwired) path ""
                # "Start with index\n= 0; prev index = -1"
                n149 = Unbundle By Name(w437) -> ("Macro File Path"=w454:refnum<vi>)
                n150 = call "FGV_MacroCore.vi"("MacroFGV_Commands"=FGV_MacroCore_Commands."Read Temp File", "Error In"=w460) -> ("Error Out"=w451:errorcluster, "Macro String Array"=w455:string[], "Saved Macro Path"=w449:path)  [unwired: 5 in, 2 out]
                n151 = call "Stage Position Safety.vi"("error in (no error)"=w451, "Macro Array IN"=w455) -> ("error out"=w444:errorcluster, "Modified Array OUT"=w448:string[])  [unwired: 7 in, 1 out]
                n152 = disable-structure shown="Enabled" {
                  disable-tunnel: [w464 _] -> w443
                  disable-tunnel: w444 -> [w463 _]
                  disable-tunnel: w442 -> [w462 _]
                  frame Enabled {
                    n153 = call <vilib>:"Create Cursor From File.vi"("error in (no error)"=w463, "cursor file"=w462) -> ("error out"=w465:errorcluster, "cursor ID"=w466:refnum<k1>)  [unwired: 8 in]
                    n154 = call <vilib>:"Set Busy.vi"("error in (no error)"=w465, "cursor ID"=w466) -> ("error out"=w464:errorcluster)  [unwired: 8 in, 1 out]
                  }
                  frame Disabled {
                  }
                }
                n155 = call "Display Update During Macro Load.vi"("Macro Error IN"=FALSE, "New Index IN"=0, "error in (no error)"=w443, "Macro Array IN"=w448, "Previous Index IN"=-1, "UI control refnums"=w437) -> ("error out"=w450:errorcluster, "New Index OUT"=w456:i32)  [unwired: 3 in, 1 out]
                n156 = property class="Path"(reference=w454, error in=w450, "Value"=w449) -> (reference out=w452:refnum<vi>, error out=w453:errorcluster)
                n157 = Close Reference(reference=w452, error in (no error)=w453) -> (error out=w441:errorcluster)
                n158 = call <vilib>:"Unset Busy.vi"("error in (no error)"=w441) -> ("error out"=w439:errorcluster)  [unwired: 10 in]
                n159 = call "TimingEstimate_Valid_Invalid_Update.vi"("Command"=enum16{"Valid", "Invalid"}."Invalid", "error in (no error)"=w439, "UI control refnums"=w437) -> ("error out"=w438:errorcluster)  [unwired: 8 in]
                n160 = call "SavedStatusUpdate.vi"("Options"=enum16{"Unsaved", "Saved"}."Unsaved", "error in (no error)"=w438, "UI control refnums"=w437) -> ("error out"=w445:errorcluster)  [unwired: 8 in]
              }
            }
            n161 = call "reg unreg for MacroGUI.vi"("T for reg, F for unreg"=TRUE, "error in (no error)"=w416, "event cluster"=w413, "Event Registration Refnum"=w414) -> ("error out"=w409:errorcluster)  [unwired: 6 in, 1 out]
          }
        }
        n162 = case shown="True" w117 {
          tunnel: w124 -> [w136 w141]
          tunnel: w123 -> [w137 _]
          tunnel: [w137 w139] -> w122
          tunnel: [w136 w138] -> w121
          frame False {
          }
          frame True {
            n163 = call "Timer.vi"("Timer Command"=Timer_Commands."Check Time", "Error In"=w141, "VI name (Optional)"="MacroGUISecondsTimer") -> ("Error Out"=w138:errorcluster, "Remaining Time (s)"=w140:dbl)  [unwired: 3 in, 4 out]
            n164 = call "Convert s_Float to ms_I32.vi"("Seconds IN (Float)"=w140) -> ("milliseconds OUT (I32)"=w139:i32)
          }
        }
      }
      event User Event {
        n165 = event-data() -> ("HB Actionable Event"=w484:T16)  [unwired: 1 in]
        n166 = case shown="\"Slave action complete event\"" w484 {
          tunnel: [w496 w505 w585 w596] -> w477
          tunnel: w483 -> [w496 w501 w585 w596]
          tunnel: w482 -> [w495 w503 w582 w601]
          tunnel: w481 -> [_ w504 w590 w594]
          tunnel: [w495 w497 w584 w592] -> w474
          tunnel: w480 -> [_ w502 _ _]
          tunnel: [w494 w500 w578 w593] -> w469
          tunnel: w468 -> [w494 w500 w578 _]
          frame Default {
          }
          frame "Slave action complete event" {
            n167 = case shown="True" w501 {
              selector: w501 -> [w512 _]
              tunnel: [w512 FALSE] -> w505
              tunnel: w504 -> [w506 w544]
              tunnel: [w507 w542] -> w498
              tunnel: w503 -> [w509 w565]
              tunnel: w502 -> [w508 w563]
              frame False {
                # "Was there a preview\nin progress?"
                n168 = call "GFGbooleanGet.vi"("Variable Name in"="Preview.Mode") -> ("Boolean Value OUT"=w510:bool)  [unwired: 9 in, 1 out]
                n169 = case shown="True" w510 {
                  tunnel: w509 -> [w513 w531]
                  tunnel: w508 -> [_ w528]
                  tunnel: [w513 w514] -> w507
                  tunnel: w506 -> [_ w517]
                  frame False {
                    # "Not preview mode - do nothing"
                  }
                  frame True {
                    n170 = call "GFG_core.vi"("Variable Name in"="Preview.Mode", "Variant in"=FALSE, "error in (no error)"=w531, "Action"=enum16{"Init", "Set", "Get", "Clear"}."Set") -> ("error out"=w527:errorcluster)  [unwired: 9 in, 6 out]
                    n171 = call "HFG_Core.vi"("HFG Commands"=HFG_Commands."Set", "Error In"=w527, "Heartbeat state IN"=Heartbeat_States."Completed" ("Run state IN"), "VI Name (Calling VIs name by default)"=w528) -> ("Error Out"=w523:errorcluster)  [unwired: 4 in, 3 out]
                    n172 = Unbundle By Name(w517) -> ("Preview Macro"=w524:refnum<vi>)
                    n173 = property class="Bool (strict)"(reference=w524, error in=w523, "Value"=FALSE) -> (reference out=w525:refnum<vi>, error out=w526:errorcluster)
                    n174 = Unbundle By Name(w517) -> ("Execute Macro"=w518:refnum<vi>)
                    n175 = Close Reference(reference=w525, error in (no error)=w526) -> (error out=w520:errorcluster)
                    n176 = call "Manage UI and GFG states during settings file edit.vi"("Commands"=Update_Scan_Settings_Commands."Finalise Update", "Error In"=w520, "UI control refnums"=w517) -> ("Error Out"=w516:errorcluster)  [unwired: 8 in]
                    n177 = Build Array(w518) -> (w515:refnum<vi>[])
                    n178 = call "UI Control and Indicator properties.vi"("Enable Command"=UI_Control_and_Indicator_properties_Commands."Enable", "Error In"=w516, "Control Refnums"=w515) -> ("Error Out"=w514:errorcluster)  [unwired: 8 in]
                  }
                }
              }
              frame True {
                w545 = u8 0 ("Progress")
                # "Invalidate Zip Path"
                n179 = Unbundle By Name(w544) -> ("Execute Macro"=w571:refnum<vi>, "Info Tbl"=w551:refnum<vi>)
                n180 = call "HFG_Core.vi"("HFG Commands"=HFG_Commands."Set", "Error In"=w565, "Heartbeat state IN"=Heartbeat_States."Completed" ("Run state IN"), "VI Name (Calling VIs name by default)"=w563) -> ("Error Out"=w564:errorcluster)  [unwired: 4 in, 3 out]
                n181 = property class="Bool (strict)"(reference=w571, error in=w564, "Val(Sgnl)"=FALSE ("Value")) -> (reference out=w568:refnum<vi>, error out=w569:errorcluster)
                n182 = Close Reference(reference=w568, error in (no error)=w569) -> (error out=w562:errorcluster)
                n183 = call "Enable-Disable SCISCAN Controls.vi"("Enable-Disable SCISCAN Controls_Command"=Enable-Disable_SCISCAN_controls_Command."Enable the items disabled earlier", "Error In"=w562) -> ("Error Out"=w552:errorcluster)  [unwired: 9 in]
                n184 = call "GFG_core.vi"("Variable Name in"="MacroZipPath", "Variant in"=path "", "Action"=enum16{"Init", "Set", "Get", "Clear"}."Set") -> ()  [unwired: 10 in, 7 out]
                n185 = call "FGV_MacroCore.vi"("MacroFGV_Commands"=FGV_MacroCore_Commands."Get Array", "Error In"=w552) -> ("Error Out"=w557:errorcluster, "Info Table Array"=w560:string[])  [unwired: 5 in, 3 out]
                n186 = Array Size(array=w560) -> (size(s)=w559:i32)
                n187 = Initialize Array("", w559) -> (w556:string[])
                n188 = Build Array(w556) -> (w555:string[][])
                n189 = disable-structure shown="Disabled" {
                  disable-tunnel: [w576 _] -> _
                  frame Disabled {
                    n190 = call "MacroExecTimeCalc.vi"() -> ("Estimated Timing cluster"=w577:T42)  [unwired: 9 in, 2 out]
                    n191 = Unbundle By Name(w577) -> ("Estimated Run time"=w576:dbl)
                  }
                  frame Enabled {
                  }
                }
                n192 = property class="Tbl (strict)"(reference=w551, error in=w557, "Value"=w555) -> (reference out=w553:refnum<vi>, error out=w554:errorcluster)
                n193 = Unbundle By Name(w544) -> ("Execution Timing"=w537:refnum<vi>)
                n194 = Close Reference(reference=w553, error in (no error)=w554) -> (error out=w550:errorcluster)
                n195 = disable-structure shown="Disabled" {
                  disable-tunnel: w550 -> [w575 _]
                  disable-tunnel: w544 -> [w574 _]
                  disable-tunnel: [w573 _] -> w543
                  frame Disabled {
                    n196 = call "Macro Debugger.vi"("Error In"=w575, "UI control refnums"=w574) -> ("Error Out"=w573:errorcluster)  [unwired: 8 in, 1 out]
                  }
                  frame Enabled {
                  }
                }
                n197 = property class="Clust (strict)"(reference=w537) -> (reference out=w536:refnum<vi>, "Value"=w535:T7)  [unwired: 1 in, 1 out]
                n198 = Bundle By Name(cluster=w535, "Remaining"=inf, "Progress"=w545, "Elapsed"=w545) -> (w548:T7)
                n199 = property class="Clust (strict)"(reference=w536, error in=w543, "Value"=w548) -> (reference out=w546:refnum<vi>, error out=w547:errorcluster)
                n200 = Close Reference(reference=w546, error in (no error)=w547) -> (error out=w542:errorcluster)
              }
            }
            n201 = call "Backup or Restore GFG Config Data.vi"("Action Select"=Backup_or_Restore_GFG_Config_Data_Commands."Restore", "error in (no error)"=w498) -> ("error out"=w497:errorcluster)  [unwired: 9 in]
          }
          frame "Broken Link" {
            n202 = Unbundle By Name(w590) -> ("Execute Macro"=w583:refnum<vi>)
            n203 = property class="Bool (strict)"(reference=w583, error in=w582, "Val(Sgnl)"=FALSE ("Value")) -> (reference out=w581:refnum<vi>, error out=w580:errorcluster)
            n204 = property class="Bool (strict)"(reference=w581, error in=w580, "DisabledEnum"=T32."Disabled and Grayed Out" ("Disabled"), "TipStrip"="One (or more) required services not running " ("Tip Strip")) -> (reference out=w588:refnum<vi>, error out=w589:errorcluster)
            n205 = Close Reference(reference=w588, error in (no error)=w589) -> (error out=w584:errorcluster)
          }
          frame "Recovered from Broken Link" {
            n206 = Unbundle By Name(w594) -> ("Execute Macro"=w602:refnum<vi>)
            n207 = property class="Bool (strict)"(reference=w602, error in=w601, "DisabledEnum"=T32."Enabled" ("Disabled"), "TipStrip"="Macro execution control" ("Tip Strip")) -> (reference out=w599:refnum<vi>, error out=w600:errorcluster)
            n208 = Close Reference(reference=w599, error in (no error)=w600) -> (error out=w595:errorcluster)
            n209 = call "Macro Debugger.vi"("Error In"=w595, "UI control refnums"=w594) -> ("Error Out"=w592:errorcluster, "Any Error?"=w593:bool)  [unwired: 8 in]
            n210 = First Call?() -> (First Call?: T/F=w591:bool)
            n211 = case shown="False" w591 {
              frame False {
                n212 = One Button Dialog(message="SciScript Module has recovered from an internal error. If you were running a macro, there is a chance this was not successfully completed") -> ()  [unwired: 1 in, 1 out]
              }
              frame True {
              }
            }
          }
        }
        n213 = case shown="True" w477 {
          tunnel: w476 -> [w487 _]
          tunnel: [w487 w490] -> w475
          tunnel: w474 -> [w486 w489]
          tunnel: [w486 w488] -> w473
          frame False {
          }
          frame True {
            n214 = call "Timer.vi"("Timer Command"=Timer_Commands."Check Time", "Error In"=w489, "VI name (Optional)"="MacroGUISecondsTimer") -> ("Error Out"=w488:errorcluster, "Remaining Time (s)"=w491:dbl)  [unwired: 3 in, 4 out]
            n215 = call "Convert s_Float to ms_I32.vi"("Seconds IN (Float)"=w491) -> ("milliseconds OUT (I32)"=w490:i32)
          }
        }
      }
      event "Select Display": Value Change {
        n216 = event-data() -> ()  [unwired: 1 in, 1 out]
        n217 = disable-structure shown="Disabled" {
          disable-tunnel: w609 -> [w618 w619]
          disable-tunnel: [w616 w619] -> w608
          frame Disabled {
            n218 = call "SCISCAN Image display TO Enum .vi"("SCISCAN Image display_to_Enum_Commands"=SCISCAN_Image_display_to_Enum_Commands."Enum to SCISCAN disp", "Error In"=w618) -> ("Error Out"=w616:errorcluster)  [unwired: 9 in]
          }
          frame Enabled {
          }
        }
      }
      event Key Down; Key Repeat {
        # "Is Macro run in progress?"
        n219 = event-data() -> ("VKey"=w630:T43)  [unwired: 1 in]
        n220 = case shown="False" w624 {
          tunnel: w630 -> [w640 _]
          tunnel: w629 -> [w639 w752]
          tunnel: [w638 w752] -> w628
          tunnel: w627 -> [w637 _]
          tunnel: w626 -> [w636 w753]
          tunnel: [w635 w753] -> w625
          frame False {
            n221 = case shown="\"Home\"" w640 {
              tunnel: w639 -> [w642 w651 w674 w703 w731]
              tunnel: [w642 w643 w672 w695 w724] -> w638
              tunnel: w637 -> [_ w652 w675 w699 w728]
              tunnel: w636 -> [w641 w648 w673 w698 w727]
              tunnel: [w641 w644 w671 w696 w725] -> w635
              frame "ASCII", Default {
              }
              frame "Down" {
                # "Is current index less than the\nmax possible index?"
                n222 = call "FGV_MacroCore.vi"("MacroFGV_Commands"=FGV_MacroCore_Commands."Get Array") -> ("Macro String Array"=w649:string[])  [unwired: 6 in, 4 out]
                n223 = Array Size(array=w649) -> (size(s)=w647:i32)
                n224 = Decrement(x=w647) -> (x-1=w646:i32)
                n225 = Less?(x=w648, y=w646) -> (x < y?=w645:bool)
                n226 = case shown="True" w645 {
                  tunnel: w652 -> [_ w670]
                  tunnel: w651 -> [w653 w668]
                  tunnel: w648 -> [w654 w667]
                  tunnel: [w654 w662] -> w644
                  tunnel: [w653 w658] -> w643
                  frame False {
                  }
                  frame True {
                    n227 = Unbundle By Name(w670) -> ("Created Macro"=w660:refnum<vi>, "Params Table"=w661:refnum<vi>, "Info Tbl"=w656:refnum<vi>)
                    n228 = Build Array(w660) -> (w659:refnum<vi>[])
                    n229 = Build Array(w661) -> (w657:refnum<vi>[])
                    n230 = call "FormatTree&TableStyle.vi"("Format Command"=FormatTree&TableStyle_Commands."Uncolour Row", "Error In"=w668, "Row Index"=w667, "Array of Table references"=w657, "Array of Tree references"=w659) -> ("Error Out"=w665:errorcluster)  [unwired: 6 in]
                    n231 = Increment(x=w667) -> (x+1=w662:i32)
                    n232 = call "FormatTree&TableStyle.vi"("Format Command"=FormatTree&TableStyle_Commands."Colour Row", "Error In"=w665, "Row Index"=w662, "Array of Table references"=w657, "Array of Tree references"=w659) -> ("Error Out"=w663:errorcluster)  [unwired: 6 in]
                    n233 = Insert Into Array(array=w657, new element=w656) -> (w655:refnum<vi>[])  [unwired: 1 in]
                    n234 = call "FormatTree&TableStyle.vi"("Format Command"=FormatTree&TableStyle_Commands."UpdateVisibleRows", "Error In"=w663, "Row Index"=w662, "Array of Table references"=w655, "Array of Tree references"=w659) -> ("Error Out"=w658:errorcluster)  [unwired: 6 in]
                  }
                }
              }
              frame "Up" {
                # "Are we at the top?"
                n235 = Greater Than 0?(x=w673) -> (x > 0?=w676:bool)
                n236 = case shown="True" w676 {
                  tunnel: w675 -> [_ w693]
                  tunnel: w674 -> [w677 w692]
                  tunnel: w673 -> [w678 w691]
                  tunnel: [w677 w685] -> w672
                  tunnel: [w678 w682] -> w671
                  frame False {
                  }
                  frame True {
                    n237 = Unbundle By Name(w693) -> ("Created Macro"=w688:refnum<vi>, "Params Table"=w687:refnum<vi>, "Info Tbl"=w681:refnum<vi>)
                    n238 = Build Array(w687) -> (w680:refnum<vi>[])
                    n239 = Build Array(w688) -> (w683:refnum<vi>[])
                    n240 = Decrement(x=w691) -> (x-1=w682:i32)
                    n241 = call "FormatTree&TableStyle.vi"("Format Command"=FormatTree&TableStyle_Commands."Uncolour Row", "Error In"=w692, "Row Index"=w691, "Array of Table references"=w680, "Array of Tree references"=w683) -> ("Error Out"=w689:errorcluster)  [unwired: 6 in]
                    n242 = call "FormatTree&TableStyle.vi"("Format Command"=FormatTree&TableStyle_Commands."Colour Row", "Error In"=w689, "Row Index"=w682, "Array of Table references"=w680, "Array of Tree references"=w683) -> ("Error Out"=w684:errorcluster)  [unwired: 6 in]
                    n243 = Insert Into Array(array=w680, new element=w681) -> (w679:refnum<vi>[])  [unwired: 1 in]
                    n244 = call "FormatTree&TableStyle.vi"("Format Command"=FormatTree&TableStyle_Commands."UpdateVisibleRows", "Error In"=w684, "Row Index"=w682, "Array of Table references"=w679, "Array of Tree references"=w683) -> ("Error Out"=w685:errorcluster)  [unwired: 6 in]
                  }
                }
              }
              frame "Home" {
                # "Are there more than\n1 entries?"
                n245 = call "FGV_MacroCore.vi"("MacroFGV_Commands"=FGV_MacroCore_Commands."Get Array", "Error In"=w703) -> ("Error Out"=w697:errorcluster, "Macro String Array"=w702:string[])  [unwired: 5 in, 3 out]
                n246 = Array Size(array=w702) -> (size(s)=w701:i32)
                n247 = Greater Than 0?(x=w701) -> (x > 0?=w700:bool)
                n248 = case shown="True" w700 {
                  tunnel: w699 -> [_ w722]
                  tunnel: w698 -> [w706 w719]
                  tunnel: w697 -> [w705 w721]
                  tunnel: [w706 w710] -> w696
                  tunnel: [w705 w712] -> w695
                  frame False {
                  }
                  frame True {
                    w710 = 0 ("Index")
                    n249 = Unbundle By Name(w722) -> ("Created Macro"=w716:refnum<vi>, "Params Table"=w715:refnum<vi>, "Info Tbl"=w708:refnum<vi>)
                    n250 = Build Array(w715) -> (w709:refnum<vi>[])
                    n251 = Build Array(w716) -> (w711:refnum<vi>[])
                    n252 = call "FormatTree&TableStyle.vi"("Format Command"=FormatTree&TableStyle_Commands."Uncolour Row", "Error In"=w721, "Row Index"=w719, "Array of Table references"=w709, "Array of Tree references"=w711) -> ("Error Out"=w717:errorcluster)  [unwired: 6 in]
                    n253 = call "FormatTree&TableStyle.vi"("Format Command"=FormatTree&TableStyle_Commands."Colour Row", "Error In"=w717, "Row Index"=w710, "Array of Table references"=w709, "Array of Tree references"=w711) -> ("Error Out"=w713:errorcluster)  [unwired: 6 in]
                    n254 = Insert Into Array(array=w709, new element=w708) -> (w707:refnum<vi>[])  [unwired: 1 in]
                    n255 = call "FormatTree&TableStyle.vi"("Format Command"=FormatTree&TableStyle_Commands."UpdateVisibleRows", "Error In"=w713, "Row Index"=w710, "Array of Table references"=w707, "Array of Tree references"=w711) -> ("Error Out"=w712:errorcluster)  [unwired: 6 in]
                  }
                }
              }
              frame "End" {
                # "Are there more than\n1 entries?"
                n256 = call "FGV_MacroCore.vi"("MacroFGV_Commands"=FGV_MacroCore_Commands."Get Array", "Error In"=w731) -> ("Error Out"=w726:errorcluster, "Macro String Array"=w730:string[])  [unwired: 5 in, 3 out]
                n257 = Array Size(array=w730) -> (size(s)=w723:i32)
                n258 = Greater Than 0?(x=w723) -> (x > 0?=w729:bool)
                n259 = case shown="True" w729 {
                  tunnel: w728 -> [_ w751]
                  tunnel: w727 -> [w734 w748]
                  tunnel: w726 -> [w733 w750]
                  tunnel: [w734 w739] -> w725
                  tunnel: [w733 w740] -> w724
                  tunnel: w723 -> [_ w745]
                  frame False {
                  }
                  frame True {
                    # "Convert to Index"
                    n260 = Unbundle By Name(w751) -> ("Created Macro"=w743:refnum<vi>, "Params Table"=w744:refnum<vi>, "Info Tbl"=w736:refnum<vi>)
                    n261 = Decrement(x=w745) -> (x-1=w739:i32)
                    n262 = Build Array(w743) -> (w738:refnum<vi>[])
                    n263 = Build Array(w744) -> (w737:refnum<vi>[])
                    n264 = call "FormatTree&TableStyle.vi"("Format Command"=FormatTree&TableStyle_Commands."Uncolour Row", "Error In"=w750, "Row Index"=w748, "Array of Table references"=w737, "Array of Tree references"=w738) -> ("Error Out"=w746:errorcluster)  [unwired: 6 in]
                    n265 = call "FormatTree&TableStyle.vi"("Format Command"=FormatTree&TableStyle_Commands."Colour Row", "Error In"=w746, "Row Index"=w739, "Array of Table references"=w737, "Array of Tree references"=w738) -> ("Error Out"=w741:errorcluster)  [unwired: 6 in]
                    n266 = Insert Into Array(array=w737, new element=w736) -> (w735:refnum<vi>[])  [unwired: 1 in]
                    n267 = call "FormatTree&TableStyle.vi"("Format Command"=FormatTree&TableStyle_Commands."UpdateVisibleRows", "Error In"=w741, "Row Index"=w739, "Array of Table references"=w735, "Array of Tree references"=w738) -> ("Error Out"=w740:errorcluster)  [unwired: 6 in]
                  }
                }
              }
            }
          }
          frame True {
          }
        }
      }
      event Edit Cell? {
        n268 = event-data() -> ()  [unwired: 1 in, 1 out]
        n269 = event-data("Discard?"=TRUE) -> ()  [unwired: 2 in, 1 out]
      }
      event Drag Starting? {
        n270 = event-data() -> ("Data"=w781:T44)  [unwired: 1 in]
        n271 = Index Array(array=w781, index=0) -> (element=w790:cluster{"data name":string, "drag data":variant})
        n272 = Unbundle By Name(w790) -> ("drag data"=w789:variant)
        n273 = Variant To Data(type="", Variant=w789) -> (data=w769:string)  [unwired: 1 in, 1 out]
        n274 = Equal?(x=w769, y="Actions") -> (x = y?=w767:bool)
        n275 = Equal?(x="Presets" ("y"), y=w769) -> (x = y?=w768:bool)
        n276 = Or(x=w768, y=w767) -> (x .or. y?=w766:bool)
        n277 = Bundle By Name(cluster=cluster{"data name":string, "drag data":variant} {"data name"="", "drag data"=variant} ("element"), "data name"="DataSource", "drag data"="AvailableActionsTree" ("data name")) -> (w782:cluster{"data name":string, "drag data":variant})
        n278 = Insert Into Array(array=w781, new element=w782) -> (w780:T44)  [unwired: 1 in]
        n279 = event-data("Data"=w780, "Drag Mode"=enum32{"copy or move", "copy only", "move only"}."copy only", "Discard?"=w766) -> ()  [unwired: 1 in, 1 out]
      }
      event Drop {
        # "Carry out a delete operation when dragged from 'Macro' tree and dropped in 'Available Actions' tree."
        n280 = event-data() -> ("Available Data Names"=w806:string[])  [unwired: 1 in]
        n281 = Index Array(array=w806, index=3) -> (element=w808:string)
        n282 = Get Drag Drop Data(8:"", 9:w808) -> (3:w807:string)  [unwired: 1 in, 1 out]
        n283 = case shown="\"MacroTree\"" w807 {
          tunnel: w804 -> [w818 w820]
          tunnel: [w813 w820] -> w811
          tunnel: w805 -> [w814 _]
          frame "MacroTree" {
            n284 = Unbundle By Name(w814) -> ("Delete"=w819:refnum<vi>)
            n285 = property class="Bool"(reference=w819, error in=w818, "Val(Sgnl)"=TRUE) -> (reference out=w815:refnum<vi>, error out=w816:errorcluster)
            n286 = Close Reference(reference=w815, error in (no error)=w816) -> (error out=w813:errorcluster)
          }
          frame Default {
          }
        }
        n287 = event-data("Accepted?"=FALSE) -> ()  [unwired: 1 in, 1 out]
      }
      event "Macro": Drag Starting? {
        # "Check if the item being dragged is part of a preset"
        n288 = event-data() -> ("Data"=w827:T44, "Coords"=w822:T45)  [unwired: 1 in]
        n289 = Unbundle By Name(w826) -> ("Created Macro"=w825:refnum<vi>)
        n290 = invoke class="Tree (strict)" method="Point To Row Column"(reference=w825, "Point"=w822) -> (reference out=w823:refnum<vi>, "Tag"=w824:string)  [unwired: 6 in, 6 out]
        n291 = call "Check if specified tag is inside a Preset.vi"("Tag to check"=w824, "Tree Refnum"=w823) -> ("Specified tag is part of a Preset?"=w821:bool)  [unwired: 6 in, 3 out]
        n292 = Bundle By Name(cluster=cluster{"data name":string, "drag data":variant} {"data name"="", "drag data"=variant} ("element"), "data name"="DataSource", "drag data"="MacroTree" ("data name")) -> (w837:cluster{"data name":string, "drag data":variant})
        n293 = Insert Into Array(array=w827, new element=w837) -> (w841:T44)  [unwired: 1 in]
        n294 = event-data("Data"=w841, "Drag Mode"=enum32{"copy or move", "copy only", "move only"}."copy only", "Discard?"=w821) -> ()  [unwired: 1 in, 1 out]
      }
      event "Macro": Drop {
        # "Unsaved changes"
        n295 = event-data() -> ("Available Data Names"=w868:string[], "Coords"=w884:T45)  [unwired: 1 in]
        n296 = Unbundle By Name(w846) -> ("Created Macro"=w883:refnum<vi>)
        n297 = invoke class="Tree (strict)" method="Point To Row Column"(reference=w883, error in=w851, "Point"=w884) -> (reference out=w869:refnum<vi>, error out=w870:errorcluster, "Tag"=w882:string)  [unwired: 5 in, 5 out]
        n298 = Index Array(array=w868, index=3) -> (element=w877:string)
        n299 = Index Array(array=w868, index=1) -> (element=w875:string)
        n300 = Index Array(array=w868, index=0) -> (element=w886:string)
        n301 = Get Drag Drop Data(8:"", 9:w875) -> (3:w872:string)  [unwired: 1 in, 1 out]
        n302 = Get Drag Drop Data(8:"", 9:w877) -> (3:w876:string)  [unwired: 1 in, 1 out]
        n303 = Get Drag Drop Data(8:"", 9:w886) -> (3:w880:string)  [unwired: 1 in, 1 out]
        n304 = Close Reference(reference=w869, error in (no error)=w870) -> (error out=w850:errorcluster)
        n305 = call <vilib>:"Create Cursor From File.vi"("error in (no error)"=w850, "cursor file"=w852) -> ("error out"=w855:errorcluster, "cursor ID"=w856:refnum<k1>)  [unwired: 8 in]
        n306 = call <vilib>:"Set Busy.vi"("error in (no error)"=w855, "cursor ID"=w856) -> ("error out"=w849:errorcluster)  [unwired: 8 in, 1 out]
        n307 = case shown="\"AvailableActionsTree\"" w876 {
          tunnel: w882 -> [w892 _ w911]
          tunnel: [w897 w901 w906] -> w881
          tunnel: w849 -> [w893 w900 w909]
          tunnel: w880 -> [w891 _ w908]
          tunnel: [w896 w900 w910] -> w847
          tunnel: w872 -> [w894 _ w904]
          tunnel: w871 -> [w898 w901 w907]
          tunnel: w846 -> [w895 _ w905]
          tunnel: w863 -> [_ w899 _]
          tunnel: [w889 w899 w902] -> w859
          frame "MacroTree" {
            n308 = call "Drop Into MacroTree.vi"("UI control refnums"=w895, "Index IN"=w898, "Source Tag"=w894, "Source Text"=w891, "Destination Tag"=w892, "Error In"=w893, "Drag Source"=T33."Macro Tree") -> ("Index OUT"=w897:i32, "Any Error? OUT"=w889:bool, "Error Out"=w896:errorcluster)  [unwired: 6 in]
          }
          frame Default {
          }
          frame "AvailableActionsTree" {
            n309 = call "Drop Into MacroTree.vi"("UI control refnums"=w905, "Index IN"=w907, "Source Tag"=w904, "Source Text"=w908, "Destination Tag"=w911, "Error In"=w909, "Drag Source"=T33."Available Operations Tree") -> ("Index OUT"=w906:i32, "Any Error? OUT"=w902:bool, "Error Out"=w910:errorcluster)  [unwired: 6 in]
          }
        }
        n310 = call "TimingEstimate_Valid_Invalid_Update.vi"("Command"=enum16{"Valid", "Invalid"}."Invalid", "error in (no error)"=w847, "UI control refnums"=w846) -> ("error out"=w845:errorcluster)  [unwired: 8 in]
        n311 = call "SavedStatusUpdate.vi"("Options"=enum16{"Unsaved", "Saved"}."Unsaved", "error in (no error)"=w845, "UI control refnums"=w846) -> ("error out"=w854:errorcluster)  [unwired: 8 in]
        n312 = call <vilib>:"Unset Busy.vi"("error in (no error)"=w854) -> ("error out"=w853:errorcluster)  [unwired: 10 in]
        n313 = event-data("Accepted?"=TRUE) -> ()  [unwired: 1 in, 1 out]
      }
      event "Macro": Mouse Down {
        # "are there any elements?"
        # "Valid selection?"
        # "Valid user selection; hence change index"
        n314 = event-data() -> ()  [unwired: 1 in, 1 out]
        n315 = Unbundle By Name(w935) -> ("Created Macro"=w931:refnum<vi>, "Params Table"=w934:refnum<vi>)
        n316 = property class="Tree (strict)"(reference=w931, error in=w930) -> (reference out=w929:refnum<vi>, error out=w932:errorcluster, "Value"=w922:string, "All Tags"=w923:string[])
        n317 = Greater Or Equal To 0?(x=w927) -> (x >= 0?=w926:bool)
        n318 = Search 1D Array(1D array=w923, element=w922) -> (index of element=w921:i32)  [unwired: 1 in]
        n319 = Greater Or Equal To 0?(x=w921) -> (x >= 0?=w920:bool)
        n320 = And(x=w926, y=w920) -> (x .and. y?=w925:bool)
        n321 = case shown="True" w925 {
          tunnel: w927 -> [w937 w946]
          tunnel: w934 -> [_ w940]
          tunnel: [w936 w942] -> w933
          tunnel: w932 -> [w936 w949]
          tunnel: w931 -> [_ w941]
          tunnel: w929 -> [_ w950]
          tunnel: w922 -> [_ w951]
          tunnel: [w937 w943] -> w928
          frame False {
          }
          frame True {
            n322 = Build Array(w940) -> (w939:refnum<vi>[])
            n323 = Build Array(w941) -> (w938:refnum<vi>[])
            n324 = call "FormatTree&TableStyle.vi"("Format Command"=FormatTree&TableStyle_Commands."Uncolour Row", "Error In"=w949, "Row Index"=w946, "Array of Table references"=w939, "Array of Tree references"=w938) -> ("Error Out"=w948:errorcluster)  [unwired: 6 in]
            n325 = call "Tree_GetIndexFromTag.vi"("Error In"=w948, "Tag IN"=w951, "Tree Refnum IN"=w950) -> ("Error Out"=w953:errorcluster, "Index OUT"=w943:i32, "Tree Refnum OUT"=w952:refnum<vi>)  [unwired: 6 in]
            n326 = Close Reference(reference=w952, error in (no error)=w953) -> (error out=w944:errorcluster)
            n327 = call "FormatTree&TableStyle.vi"("Format Command"=FormatTree&TableStyle_Commands."Colour Row", "Error In"=w944, "Row Index"=w943, "Array of Table references"=w939, "Array of Tree references"=w938) -> ("Error Out"=w942:errorcluster)  [unwired: 6 in]
          }
        }
      }
      event "MacroTreeOperation": Mouse Up {
        # "Stop looking for a Scroll action"
        n328 = event-data() -> ()  [unwired: 1 in, 8 out]
      }
      event "Macro": event type 3.0.x80000011 {
        n329 = event-data() -> ()  [unwired: 1 in, 5 out]
        n330 = event-data("Discard?"=TRUE) -> ()  [unwired: 1 in, 1 out]
      }
      event "Parameters": Mouse Down {
        # "Also ensure there is a \nchange in the row selected\n(Mouse down is also being\nlistned to for scroll functionality)"
        # "Timeout to check for scroll"
        # "Is selection valid?\nIf yes, get index"
        n331 = event-data() -> ()  [unwired: 1 in, 1 out]
        n332 = Unbundle By Name(w1002) -> ("Created Macro"=w992:refnum<vi>, "Params Table"=w998:refnum<vi>)
        n333 = property class="Tbl (strict)"(reference=w998, error in=w997) -> (reference out=w996:refnum<vi>, error out=w995:errorcluster, "Selection Start"=w987:T46)
        n334 = call "Tree_GetAll.vi"("Tree Refnum IN"=w992) -> ("Tags"=w993:string[])  [unwired: 7 in, 3 out]
        n335 = Unbundle By Name(w987) -> ("Row"=w985:i32)
        n336 = Array Size(array=w993) -> (size(s)=w1001:i32)
        n337 = feedback-in #1(w985) -> ()
        n338 = feedback #1() -> (w988:i32)  [unwired: 1 in]
        n339 = Greater?(x=w1001, y=w985) -> (0:w986:bool)
        n340 = Not Equal?(x=w985, y=w988) -> (x != y?=w984:bool)
        n341 = And(x=w986, y=w984) -> (x .and. y?=w983:bool)
        n342 = case shown="True" w983 {
          tunnel: w1000 -> [w1008 w1018]
          tunnel: [w1008 w1015] -> w999
          tunnel: w996 -> [w1004 w1012]
          tunnel: w992 -> [w1003 w1009]
          tunnel: w985 -> [_ w1015]
          tunnel: w995 -> [w1007 w1019]
          tunnel: [w1005 w1013] -> w994
          frame False {
            # "Invalid user selection!\nDo nothing"
            n343 = Close Reference(reference=w1004, error in (no error)=w1007) -> (error out=w1006:errorcluster)
            n344 = Close Reference(reference=w1003, error in (no error)=w1006) -> (error out=w1005:errorcluster)
          }
          frame True {
            # "Valid user selection; hence change index and\ncolur the table and tree accordingly"
            n345 = Build Array(w1012) -> (w1010:refnum<vi>[])
            n346 = Build Array(w1009) -> (w1011:refnum<vi>[])
            n347 = call "FormatTree&TableStyle.vi"("Format Command"=FormatTree&TableStyle_Commands."Uncolour Row", "Error In"=w1019, "Row Index"=w1018, "Array of Table references"=w1010, "Array of Tree references"=w1011) -> ("Error Out"=w1017:errorcluster)  [unwired: 6 in]
            n348 = property class="Tree (strict)"(reference=w1009, error in=w1017, "Active Item Row Number"=w1015) -> (reference out=w1021:refnum<vi>, error out=w1022:errorcluster)
            n349 = Close Reference(reference=w1021, error in (no error)=w1022) -> (error out=w1014:errorcluster)
            n350 = call "FormatTree&TableStyle.vi"("Format Command"=FormatTree&TableStyle_Commands."Colour Row", "Error In"=w1014, "Row Index"=w1015, "Array of Table references"=w1010, "Array of Tree references"=w1011) -> ("Error Out"=w1013:errorcluster)  [unwired: 6 in]
          }
        }
      }
      event "Parameters": Mouse Up {
        n351 = event-data() -> ()  [unwired: 1 in, 5 out]
      }
      event "Parameters": Value Change {
        n352 = event-data() -> ("OldVal"=w1056:string[][])  [unwired: 1 in]
        n353 = call "reg unreg for MacroGUI.vi"("T for reg, F for unreg"=FALSE, "error in (no error)"=w1044, "event cluster"=w1036, "Event Registration Refnum"=w1038) -> ("error out"=w1043:errorcluster, "Event Registration Refnum Out"=w1037:refnum<event-registration>)  [unwired: 6 in]
        n354 = Unbundle By Name(w1058) -> ("Params Table"=w1057:refnum<vi>)
        n355 = property class="Tbl (strict)"(reference=w1057, error in=w1043, "Value"=w1056) -> (reference out=w1054:refnum<vi>, error out=w1055:errorcluster)
        n356 = Close Reference(reference=w1054, error in (no error)=w1055) -> (error out=w1042:errorcluster)
        n357 = flat-sequence {
          tunnel: w1042 -> [w1060]
          tunnel: [w1060] -> w1040
          frame #0 {
            n358 = call "Dialog_CannotEditMacroParam_Error.vi"() -> ()  [unwired: 12 in]
          }
        }
        n359 = call "reg unreg for MacroGUI.vi"("T for reg, F for unreg"=TRUE, "error in (no error)"=w1040, "event cluster"=w1036, "Event Registration Refnum"=w1037) -> ("error out"=w1039:errorcluster, "Event Registration Refnum Out"=w1035:refnum<event-registration>)  [unwired: 6 in]
      }
      event "Info": Mouse Down {
        n360 = event-data() -> ("CtlRef"=w1079:refnum<vi>, "Coords"=w1078:T45)  [unwired: 1 in]
        n361 = Unbundle By Name(w1068) -> ("Info Tbl"=w1067:refnum<vi>)
        n362 = call "Select a new macro line.vi"("error in (no error)"=w1072, "Index IN"=w1069, "Clicked Table reference"=w1067, "UI control refnums"=w1068) -> ("error out"=w1071:errorcluster, "Index Out"=w1070:i32)  [unwired: 6 in]
        n363 = invoke class="Tbl (strict)" method="Point To Row Column"(reference=w1079, error in=w1071, "Point"=w1078) -> (reference out=w1088:refnum<vi>, error out=w1089:errorcluster, "CellPosition"=w1087:T46)  [unwired: 3 in, 3 out]
        n364 = Close Reference(reference=w1088, error in (no error)=w1089) -> (error out=w1082:errorcluster)
        n365 = Unbundle By Name(w1087) -> ("Row"=w1084:i32)
        n366 = call "MacroErrorsFGV.vi"("MacroErrorsFGV_Commands"=MacroErrorsFGV_Commands."Get Error Array", "Error In"=w1082) -> ("Error Out"=w1080:errorcluster, "Error Array OUT"=w1085:T47[])  [unwired: 8 in]
        n367 = Index Array(array=w1085, index=w1084) -> (element=w1083:T47)
        n368 = Unbundle By Name(w1083) -> ("Error?"=w1065:bool, "Warning?"=w1066:bool, "Description"=w1077:string)
        n369 = Or(x=w1065, y=w1066) -> (x .or. y?=w1073:bool)
        n370 = case shown="True" w1073 {
          tunnel: [w1096 w1101] -> w1081
          tunnel: w1080 -> [w1096 w1104]
          tunnel: w1077 -> [_ w1109]
          tunnel: w1066 -> [_ w1108]
          tunnel: w1065 -> [_ w1107]
          tunnel: w1064 -> [w1095 w1100]
          tunnel: w1063 -> [_ w1098]
          tunnel: [w1095 w1097] -> w1062
          frame False {
          }
          frame True {
            n371 = call "reg unreg for MacroGUI.vi"("T for reg, F for unreg"=FALSE, "error in (no error)"=w1104, "event cluster"=w1098, "Event Registration Refnum"=w1100) -> ("error out"=w1103:errorcluster, "Event Registration Refnum Out"=w1099:refnum<event-registration>)  [unwired: 6 in]
            n372 = call "Dialog Macro Error Description.vi"("Error In"=w1103, "Warning?"=w1108, "Error?"=w1107, "Error Description IN"=w1109) -> ("Error Out"=w1102:errorcluster)  [unwired: 7 in]
            n373 = call "reg unreg for MacroGUI.vi"("T for reg, F for unreg"=TRUE, "error in (no error)"=w1102, "event cluster"=w1098, "Event Registration Refnum"=w1099) -> ("error out"=w1101:errorcluster, "Event Registration Refnum Out"=w1097:refnum<event-registration>)  [unwired: 6 in]
          }
        }
      }
      event "Info": Value Change {
        # "Dont let user change any value in the Info table"
        n374 = event-data() -> ("CtlRef"=w1119:refnum<vi>, "OldVal"=w1117:string[][])  [unwired: 1 in]
        n375 = property class="Tbl (strict)"(reference=w1119, error in=w1118, "Value"=w1117) -> (reference out=w1115:refnum<vi>, error out=w1116:errorcluster)
        n376 = Close Reference(reference=w1115, error in (no error)=w1116) -> (error out=w1114:errorcluster)
      }
      event "Execute Macro": Value Change {
        n377 = event-data() -> ("NewVal"=w1137:bool)  [unwired: 1 in]
        n378 = case shown="True" w1137 {
          tunnel: [w1155 w1251] -> w1139
          tunnel: w1138 -> [w1196 w1227]
          tunnel: w1136 -> [w1195 w1295]
          tunnel: [FALSE TRUE] -> w1135
          tunnel: w1133 -> [w1154 w1286]
          tunnel: [-1 ("Index") 1000 ("Index")] -> w1130
          tunnel: [_ w1250] -> w1127
          frame False {
            # "Invalidate Zip Path"
            # "Clear any ROI that has\nbeen drawn (for LineScan)"
            # "Stop stage first"
            n379 = call "HFG_Core.vi"("HFG Commands"=HFG_Commands."Set", "Error In"=w1196, "Heartbeat state IN"=Heartbeat_States."Cancelled" ("Run state IN"), "VI Name (Calling VIs name by default)"=w1195) -> ("Error Out"=w1169:errorcluster)  [unwired: 4 in, 3 out]
            n380 = Unbundle By Name(w1154) -> ("Info Tbl"=w1147:refnum<vi>, "Avail. Operations"=w1178:refnum<vi>, "Created Macro"=w1177:refnum<vi>, "Load Macro"=w1176:refnum<vi>, "Save Macro"=w1175:refnum<vi>, "Params Table"=w1174:refnum<vi>, "Delete"=w1173:refnum<vi>, "Edit Button"=w1172:refnum<vi>, "Preview Macro"=w1150:refnum<vi>, "New Macro"=w1149:refnum<vi>, "Copy"=w1148:refnum<vi>, "Get Positions"=w1146:refnum<vi>, "Refresh Timing"=w1141:refnum<vi>)
            n381 = Build Array(w1147, w1178, w1177, w1176, w1175, w1174, w1173, w1172, w1150, w1149, w1148, w1146, w1141) -> (w1170:refnum<vi>[])
            n382 = call "UI Control and Indicator properties.vi"("Enable Command"=UI_Control_and_Indicator_properties_Commands."Enable", "Error In"=w1169, "Control Refnums"=w1170) -> ("Error Out"=w1168:errorcluster)  [unwired: 8 in]
            n383 = call "GFG_core.vi"("Variable Name in"="Stage Stop", "Variant in"=TRUE, "Action"=enum16{"Init", "Set", "Get", "Clear"}."Set") -> ("error out"=w1179:errorcluster)  [unwired: 10 in, 6 out]
            n384 = call "Enable-Disable SCISCAN Controls.vi"("Enable-Disable SCISCAN Controls_Command"=Enable-Disable_SCISCAN_controls_Command."Enable the items disabled earlier", "Error In"=w1168) -> ("Error Out"=w1158:errorcluster)  [unwired: 9 in]
            n385 = call "GFG_core.vi"("Variable Name in"="Shutter", "Variant in"=FALSE, "error in (no error)"=w1179, "Action"=enum16{"Init", "Set", "Get", "Clear"}."Set") -> ("error out"=w1184:errorcluster)  [unwired: 9 in, 6 out]
            n386 = call "FGV_MacroCore.vi"("MacroFGV_Commands"=FGV_MacroCore_Commands."Get Array", "Error In"=w1158) -> ("Error Out"=w1163:errorcluster, "Info Table Array"=w1166:string[])  [unwired: 5 in, 3 out]
            n387 = Array Size(array=w1166) -> (size(s)=w1165:i32)
            n388 = call "GFG_core.vi"("Variable Name in"="Record", "Variant in"=FALSE, "error in (no error)"=w1184, "Action"=enum16{"Init", "Set", "Get", "Clear"}."Set") -> ("error out"=w1183:errorcluster)  [unwired: 9 in, 6 out]
            n389 = Initialize Array("", w1165) -> (w1162:string[])
            n390 = Build Array(w1162) -> (w1161:string[][])
            n391 = property class="Tbl (strict)"(reference=w1147, error in=w1163, "Value"=w1161) -> (reference out=w1159:refnum<vi>, error out=w1160:errorcluster)
            n392 = call "GFG_core.vi"("Variable Name in"="FOCUS", "Variant in"=FALSE, "error in (no error)"=w1183, "Action"=enum16{"Init", "Set", "Get", "Clear"}."Set") -> ()  [unwired: 9 in, 7 out]
            n393 = Close Reference(reference=w1159, error in (no error)=w1160) -> (error out=w1152:errorcluster)
            n394 = call "Draw ROI on Line Scan Display.vi"("Draw ROI on Line Scan Display_Command"=Draw_ROI_on_Line_Scan_Display_Command."Clear ROI", "error in (no error)"=w1152) -> ("error out"=w1151:errorcluster)  [unwired: 9 in]
            n395 = call "Backup or Restore GFG Config Data.vi"("Action Select"=Backup_or_Restore_GFG_Config_Data_Commands."Restore") -> ()  [unwired: 10 in, 1 out]
            n396 = disable-structure shown="Disabled" {
              disable-tunnel: [w1206 _] -> w1155
              disable-tunnel: w1154 -> [w1202 _]
              disable-tunnel: w1151 -> [w1199 _]
              frame Disabled {
                w1207 = u8 0 ("Progress")
                n397 = Unbundle By Name(w1202) -> ("Execution Timing"=w1201:refnum<vi>)
                n398 = call "MacroExecTimeCalc.vi"("Error In"=w1199) -> ("Error Out"=w1203:errorcluster, "Estimated Timing cluster"=w1205:T42)  [unwired: 8 in, 1 out]
                n399 = Unbundle By Name(w1205) -> ("Estimated Run time"=w1204:dbl)
                n400 = Bundle By Name(cluster=T7 {"Est. Time"=0.0, "Remaining"=0.0, "Progress"=0, "Elapsed"=0.0} ("Value"), "Est. Time"=w1204, "Remaining"=inf, "Progress"=w1207, "Elapsed"=w1207) -> (w1210:T7)
                n401 = property class="Clust (strict)"(reference=w1201, error in=w1203, "Value"=w1210) -> (reference out=w1208:refnum<vi>, error out=w1209:errorcluster)
                n402 = Close Reference(reference=w1208, error in (no error)=w1209) -> (error out=w1206:errorcluster)
              }
              frame Enabled {
              }
            }
            n403 = call "GFG_core.vi"("Variable Name in"="MacroZipPath", "Variant in"=path "", "Action"=enum16{"Init", "Set", "Get", "Clear"}."Set") -> ()  [unwired: 10 in, 7 out]
          }
          frame True {
            # "Timeout every second to update\nexecution progress"
            n404 = Unbundle By Name(w1286) -> ("Info Tbl"=w1245:refnum<vi>, "Created Macro"=w1284:refnum<vi>, "Params Table"=w1283:refnum<vi>, "Preview Macro"=w1249:refnum<vi>, "Load Macro"=w1292:refnum<vi>, "Save Macro"=w1291:refnum<vi>, "Delete"=w1290:refnum<vi>, "Edit Button"=w1289:refnum<vi>, "Copy"=w1248:refnum<vi>, "New Macro"=w1247:refnum<vi>, "Get Positions"=w1246:refnum<vi>, "Avail. Operations"=w1244:refnum<vi>, "Refresh Timing"=w1224:refnum<vi>, "Execution Timing"=w1222:refnum<vi>)
            n405 = call "GFG_core.vi"("Variable Name in"="Stage Stop", "Variant in"=TRUE, "error in (no error)"=w1227, "Action"=enum16{"Init", "Set", "Get", "Clear"}."Set") -> ("error out"=w1228:errorcluster)  [unwired: 9 in, 6 out]
            n406 = Build Array(w1245, w1284, w1283) -> (w1282:refnum<vi>[])
            n407 = Build Array(w1249, w1292, w1291, w1290, w1289, w1248, w1247, w1246, w1244, w1224) -> (w1287:refnum<vi>[])
            n408 = call "GFG_core.vi"("Variable Name in"="Shutter", "Variant in"=FALSE, "error in (no error)"=w1228, "Action"=enum16{"Init", "Set", "Get", "Clear"}."Set") -> ("error out"=w1233:errorcluster)  [unwired: 9 in, 6 out]
            n409 = call "GFG_core.vi"("Variable Name in"="Record", "Variant in"=FALSE, "error in (no error)"=w1233, "Action"=enum16{"Init", "Set", "Get", "Clear"}."Set") -> ("error out"=w1232:errorcluster)  [unwired: 9 in, 6 out]
            n410 = call "FGV_MacroCore.vi"("MacroFGV_Commands"=FGV_MacroCore_Commands."Get Array") -> ("Error Out"=w1271:errorcluster, "Info Table Array"=w1274:string[])  [unwired: 6 in, 3 out]
            n411 = call "GFG_core.vi"("Variable Name in"="FOCUS", "Variant in"=FALSE, "error in (no error)"=w1232, "Action"=enum16{"Init", "Set", "Get", "Clear"}."Set") -> ("error out"=w1226:errorcluster)  [unwired: 9 in, 6 out]
            n412 = Array Size(array=w1274) -> (size(s)=w1273:i32)
            n413 = call "Wait till all GFG events stop_for fixed duration.vi"("error in (no error)"=w1226) -> ("error out"=w1225:errorcluster)  [unwired: 10 in]
            n414 = call "UI Control and Indicator properties.vi"("Enable Command"=UI_Control_and_Indicator_properties_Commands."Disable and Grey", "Error In"=w1225, "Control Refnums"=w1287) -> ("Error Out"=w1281:errorcluster)  [unwired: 8 in]
            n415 = call "UI Control and Indicator properties.vi"("Enable Command"=UI_Control_and_Indicator_properties_Commands."Disable", "Error In"=w1281, "Control Refnums"=w1282) -> ("Error Out"=w1280:errorcluster)  [unwired: 8 in]
            n416 = call "Enable-Disable SCISCAN Controls.vi"("Enable-Disable SCISCAN Controls_Command"=Enable-Disable_SCISCAN_controls_Command."Disable and Gray", "Error In"=w1280) -> ("Error Out"=w1293:errorcluster)  [unwired: 9 in]
            n417 = call "FGV_MacroCore.vi"("MacroFGV_Commands"=FGV_MacroCore_Commands."Get Array", "Error In"=w1293) -> ("Error Out"=w1279:errorcluster, "Macro String Array"=w1219:string[])  [unwired: 5 in, 3 out]
            n418 = call "Macro_Text Array to Instruction and Argument array.vi"("Error In"=w1279, "Macro Array IN"=w1219) -> ("Error Out"=w1218:errorcluster, "Argument List (Txt)"=w1276:string[], "Action List (Txt)"=w1277:string[])  [unwired: 7 in]
            n419 = Initialize Array("", w1273) -> (w1270:string[])
            n420 = for {
              shift-right: [w1323] -> w1300
              shift-left: w1218 -> [w1323]
              tunnel: [w1320] -> w1278 mode=indexing
              tunnel: w1277 -> [w1322] mode=indexing
              tunnel: w1276 -> [w1321] mode=indexing
              i -> [w1318]
              # "clear info\ntable"
              n421 = Concatenate Strings(w1322, w1321) -> (w1320:string)
              n422 = call "FGV_MacroCore.vi"("Final Index"=w1318, "MacroFGV_Commands"=FGV_MacroCore_Commands."UpdateInfoTable", "Start Index"=w1318, "Macro Command or Info (String)"="") -> ()  [unwired: 3 in, 5 out]
            }
            n423 = Build Array(w1270) -> (w1269:string[][])
            n424 = property class="Tbl (strict)"(reference=w1245, error in=w1271, "Value"=w1269) -> (reference out=w1267:refnum<vi>, error out=w1268:errorcluster)
            n425 = property class="Clust (strict)"(reference=w1222) -> (reference out=w1215:refnum<vi>, "Value"=w1214:T7)  [unwired: 1 in, 1 out]
            n426 = Close Reference(reference=w1267, error in (no error)=w1268) -> ()  [unwired: 1 out]
            n427 = Bundle By Name(cluster=w1214, "Progress"=u8 0) -> (w1212:T7)
            n428 = Unbundle By Name(w1214) -> ("Est. Time"=w1221:dbl)
            n429 = call "GFG_core.vi"("Variable Name in"="Macro", "Variant in"=w1278, "error in (no error)"=w1300, "Action"=enum16{"Init", "Set", "Get", "Clear"}."Set") -> ("error out"=w1217:errorcluster)  [unwired: 9 in, 6 out]
            n430 = call "MacroExecution and Timing.vi"("MacroExecution and Timing Command"=Macro_Execution_and_Timing_Commands."Initialize (Update FGV & Rst Idx)" ("MacroExecution Command"), "Error In"=w1217, "Macro IN"=w1219) -> ("Error Out"=w1216:errorcluster)  [unwired: 3 in, 5 out]
            n431 = disable-structure shown="Disabled" {
              disable-tunnel: w1217 -> [w1315 w1316]
              disable-tunnel: [w1314 w1316] -> _
              disable-tunnel: [w1313 _] -> w1223
              frame Disabled {
                n432 = call "MacroExecTimeCalc.vi"("Error In"=w1315) -> ("Error Out"=w1314:errorcluster, "Estimated Timing cluster"=w1313:T42)  [unwired: 8 in, 1 out]
              }
              frame Enabled {
              }
            }
            n433 = property class="Clust (strict)"(reference=w1215, "Value"=w1212) -> ()  [unwired: 1 in, 2 out]
            n434 = call "HFG_Core.vi"("HFG Commands"=HFG_Commands."Set", "Error In"=w1216, "Heartbeat state IN"=Heartbeat_States."Instruction Issued" ("Run state IN"), "VI Name (Calling VIs name by default)"=w1295) -> ("Error Out"=w1259:errorcluster)  [unwired: 4 in, 3 out]
            n435 = disable-structure shown="Disabled" {
              disable-tunnel: [w1311 _] -> w1264
              disable-tunnel: [w1308 _] -> _
              disable-tunnel: w1223 -> [w1309 _]
              frame Disabled {
                w1310 = u8 0 ("Progress")
                n436 = Unbundle By Name(w1309) -> ("Estimated Run time"=w1308:dbl)
                n437 = Bundle By Name(cluster=T7 {"Est. Time"=0.0, "Remaining"=0.0, "Progress"=0, "Elapsed"=0.0} ("Value"), "Est. Time"=w1308, "Remaining"=w1308, "Progress"=w1310, "Elapsed"=w1310) -> (w1311:T7)
              }
              frame Enabled {
              }
            }
            n438 = call "Timer.vi"("Timer Command"=Timer_Commands."Start", "Error In"=w1259, "VI name (Optional)"="MacroExecutionTimer", "Set Time IN (s)"=w1221) -> ("Error Out"=w1257:errorcluster)  [unwired: 2 in, 5 out]
            n439 = disable-structure shown="Disabled" {
              disable-tunnel: w1264 -> [w1307 _]
              disable-tunnel: w1257 -> [w1304 _]
              disable-tunnel: w1222 -> [w1303 _]
              disable-tunnel: [w1302 _] -> w1255
              frame Disabled {
                n440 = property class="Clust (strict)"(reference=w1303, error in=w1304, "Value"=w1307) -> (reference out=w1305:refnum<vi>, error out=w1306:errorcluster)
                n441 = Close Reference(reference=w1305, error in (no error)=w1306) -> (error out=w1302:errorcluster)
              }
              frame Enabled {
              }
            }
            n442 = call "Timer.vi"("Timer Command"=Timer_Commands."Start", "VI name (Optional)"="MacroGUISecondsTimer", "Set Time IN (s)"=1.0) -> ()  [unwired: 3 in, 6 out]
            n443 = call "MacroFileIO.vi"("MacroFileIO_Command"=MacroFileIO_Commands."Save in today's folder", "Error In"=w1255) -> ("Error Out"=w1252:errorcluster)  [unwired: 8 in, 5 out]
            n444 = call "Backup or Restore GFG Config Data.vi"("Action Select"=Backup_or_Restore_GFG_Config_Data_Commands."Backup") -> ()  [unwired: 10 in, 1 out]
            n445 = call "Timer.vi"("Timer Command"=Timer_Commands."Start", "Error In"=w1252, "VI name (Optional)"="MacroGUIelapsed") -> ("Error Out"=w1251:errorcluster, "Elapsed Time (s)"=w1250:dbl)  [unwired: 3 in, 4 out]
          }
        }
      }
      event Panel Close? {
        # "When user closes the Macro UI:\nHide the window  if there is no macro currently executing\nElse, Ignore"
        # "Donot stop running this VI when user closes window\n- Set FP state to Hidden instead which can be reactivated form the main VI"
        n446 = event-data() -> ()  [unwired: 1 in, 1 out]
        n447 = case shown="True" w1330 {
          tunnel: w1333 -> [w1338 w1343]
          tunnel: [w1337 w1343] -> w1332
          frame False {
            n448 = control-ref of="This VI"() -> (w1342:refnum<vi>)
            n449 = property class="VI"(reference=w1342, error in=w1338, "FP.State"=T38."Hidden" ("Front Panel Window:State")) -> (reference out=w1339:refnum<vi>, error out=w1340:errorcluster)
            n450 = Close Reference(reference=w1339, error in (no error)=w1340) -> (error out=w1337:errorcluster)
          }
          frame True {
          }
        }
        n451 = event-data("Discard?"=TRUE) -> ()  [unwired: 1 in, 1 out]
      }
      event Timeout {
        n452 = event-data() -> ()  [unwired: 1 in, 1 out]
        n453 = case shown="True" w1355 {
          tunnel: w1359 -> [w1367 w1392]
          tunnel: w1358 -> [w1368 w1420]
          tunnel: [w1366 w1403] -> w1357
          tunnel: [w1369 w1402] -> w1354
          tunnel: w1353 -> [w1372 w1398]
          tunnel: [w1372 w1397] -> w1352
          tunnel: [w1371 w1393] -> w1351
          tunnel: w1350 -> [w1371 _]
          tunnel: w1347 -> [w1370 _]
          tunnel: w1346 -> [w1362 _]
          tunnel: w1345 -> [w1364 _]
          tunnel: w1344 -> [w1363 _]
          frame False {
            # "Possible Scroll!\nMake sure Index of Info Table matches that of Macro"
            n454 = Greater Or Equal?(x=w1363, y=w1364) -> (x >= y?=w1361:bool)
            n455 = And(x=w1362, y=w1361) -> (x .and. y?=w1365:bool)
            n456 = case shown="True" w1365 {
              tunnel: w1370 -> [_ w1378]
              tunnel: [-1 ("Index") w1378] -> w1369
              tunnel: w1368 -> [_ w1390]
              tunnel: w1367 -> [w1373 w1388]
              tunnel: [w1373 w1375] -> w1366
              frame False {
                # "Stop timing out and updating execution progress\nas there is no execution in progress OR possible scroll"
              }
              frame True {
                n457 = Unbundle By Name(w1390) -> ("Info Tbl"=w1383:refnum<vi>, "Created Macro"=w1389:refnum<vi>)
                n458 = property class="Tree (strict)"(reference=w1389, error in=w1388) -> (reference out=w1386:refnum<vi>, error out=w1387:errorcluster, "TopLeft"=w1385:T23)
                n459 = Unbundle(w1385) -> ("Node"=w1384:string)  [unwired: 1 out]
                n460 = call "Tree_GetIndexFromTag.vi"("Error In"=w1387, "Tag IN"=w1384, "Tree Refnum IN"=w1386) -> ("Error Out"=w1382:errorcluster, "Index OUT"=w1380:i32)  [unwired: 6 in, 1 out]
                n461 = Bundle By Name(cluster=T19 {"Row"=0, "Column"=0} ("Index Values"), "Row"=w1380) -> (w1379:T19)
                n462 = property class="Tbl (strict)"(reference=w1383, error in=w1382, "Index Values"=w1379) -> (reference out=w1376:refnum<vi>, error out=w1377:errorcluster)
                n463 = Close Reference(reference=w1376, error in (no error)=w1377) -> (error out=w1375:errorcluster)
              }
            }
          }
          frame True {
            # "Timeout ever second to update\nexecution progress"
            n464 = Unbundle By Name(w1420) -> ("Execution Timing"=w1412:refnum<vi>)
            n465 = call "Timer.vi"("Timer Command"=Timer_Commands."Check Time", "Error In"=w1392, "VI name (Optional)"="MacroGUIelapsed") -> ("Error Out"=w1391:errorcluster, "Elapsed Time (s)"=w1393:dbl)  [unwired: 3 in, 4 out]
            n466 = call "Timer.vi"("Timer Command"=Timer_Commands."Check Time", "Error In"=w1391, "VI name (Optional)"="MacroExecutionTimer") -> ("Error Out"=w1413:errorcluster, "Set Time OUT (s)"=w1411:dbl)  [unwired: 3 in, 4 out]
            n467 = Divide(x=w1398, y=w1411) -> (x/y=w1410:dbl)
            n468 = Multiply(x=w1410, y=100.0) -> (x*y=w1408:dbl)
            n469 = To Unsigned Byte Integer(number=w1408) -> (unsigned 8bit integer=w1400:u8)
            n470 = Subtract(x=u8 100 ("unsigned 8bit integer"), y=w1400) -> (x-y=w1399:u8)
            n471 = Bundle By Name(cluster=T7 {"Est. Time"=0.0, "Remaining"=0.0, "Progress"=0, "Elapsed"=0.0} ("Value"), "Est. Time"=w1411, "Remaining"=w1398, "Progress"=w1399, "Elapsed"=w1393) -> (w1416:T7)
            n472 = property class="Clust (strict)"(reference=w1412, error in=w1413, "Value"=w1416) -> (reference out=w1414:refnum<vi>, error out=w1415:errorcluster)
            n473 = Close Reference(reference=w1414, error in (no error)=w1415) -> (error out=w1404:errorcluster)
            n474 = call "Timer.vi"("Timer Command"=Timer_Commands."Start", "Error In"=w1404, "VI name (Optional)"="MacroGUISecondsTimer", "Set Time IN (s)"=1.0) -> ("Error Out"=w1403:errorcluster, "Remaining Time (s)"=w1405:dbl)  [unwired: 2 in, 4 out]
            n475 = call "Convert s_Float to ms_I32.vi"("Seconds IN (Float)"=w1405) -> ("milliseconds OUT (I32)"=w1402:i32)
            n476 = Decrement(x=w1398) -> (x-1=w1397:dbl)
          }
        }
      }
      event "File Operation Cluster.New Macro": Value Change {
        # "If any unsaved changes,\nwarn user to save"
        n477 = event-data() -> ()  [unwired: 1 in, 2 out]
        n478 = case shown="True" w1421 {
          tunnel: w1427 -> [w1440 w1443]
          tunnel: [w1440 w1442] -> w1423
          tunnel: [TRUE ("Confirmed?") w1441] -> w1422
          frame False {
          }
          frame True {
            n479 = call "Dialog macro changes not saved warning.vi"("error in (no error)"=w1443) -> ("error out"=w1442:errorcluster, "Confirmed?"=w1441:bool)  [unwired: 9 in]
          }
        }
        n480 = case shown="True" w1422 {
          tunnel: [w1444 w1467] -> w1432
          tunnel: w1431 -> [_ w1448]
          tunnel: [w1445 w1462] -> w1430
          tunnel: w1429 -> [w1445 w1461]
          tunnel: [w1446 w1449] -> w1428
          tunnel: w1423 -> [w1446 w1453]
          tunnel: w1426 -> [w1447 _]
          tunnel: w1425 -> [w1444 _]
          tunnel: [w1447 -1 ("Index")] -> w1424
          frame False {
          }
          frame True {
            w1460 = -1 ("New Index IN")
            n481 = Unbundle By Name(w1448) -> ("Info Tbl"=w1475:refnum<vi>, "Params Table"=w1474:refnum<vi>, "Created Macro"=w1473:refnum<vi>)
            n482 = call "FGV_MacroCore.vi"("MacroFGV_Commands"=FGV_MacroCore_Commands."Get Array", "Error In"=w1453) -> ("Error Out"=w1456:errorcluster, "Macro String Array"=w1455:string[])  [unwired: 5 in, 3 out]
            n483 = Build Array(w1473) -> (w1458:refnum<vi>[])
            n484 = Build Array(w1475, w1474) -> (w1459:refnum<vi>[])
            n485 = for {
              tunnel: w1455 -> [_] mode=indexing
              tunnel: w1459 -> [w1487]
              tunnel: w1458 -> [w1486]
              shift-right: [w1484] -> w1457
              shift-left: w1456 -> [w1485]
              i -> [w1488]
              n486 = call "FormatTree&TableStyle.vi"("Format Command"=FormatTree&TableStyle_Commands."Uncolour Row", "Error In"=w1485, "Row Index"=w1488, "Array of Table references"=w1487, "Array of Tree references"=w1486) -> ("Error Out"=w1484:errorcluster)  [unwired: 6 in]
            }
            n487 = for {
              tunnel: w1455 -> [_] mode=indexing
              shift-right: [w1491] -> w1454
              shift-left: w1457 -> [w1491]
              w1490 = 0 ("Final Index")
              n488 = call "FGV_MacroCore.vi"("Final Index"=w1490, "MacroFGV_Commands"=FGV_MacroCore_Commands."Delete instruction", "Start Index"=w1490) -> ()  [unwired: 4 in, 5 out]
            }
            n489 = invoke class="Tree (strict)" method="Edit Tree Items.Delete"(reference=w1473, error in=w1454, "tag"="" ("Tag"), "Delete Children"=TRUE ("Delete Children?")) -> (reference out=w1480:refnum<vi>, error out=w1481:errorcluster)  [unwired: 1 in, 3 out]
            n490 = Close Reference(reference=w1480, error in (no error)=w1481) -> (error out=w1477:errorcluster)
            n491 = property class="Tbl (strict)"(reference=w1474, error in=w1477, "Value"=string[][] []) -> (reference out=w1478:refnum<vi>, error out=w1479:errorcluster)
            n492 = Close Reference(reference=w1478, error in (no error)=w1479) -> (error out=w1471:errorcluster)
            n493 = Unbundle By Name(w1448) -> ("Macro File Path"=w1469:refnum<vi>)
            n494 = call "FGV_MacroCore.vi"("MacroFGV_Commands"=FGV_MacroCore_Commands."New Macro", "Error In"=w1471) -> ("Error Out"=w1468:errorcluster, "Macro String Array"=w1464:string[], "Saved Macro Path"=w1467:path)  [unwired: 5 in, 2 out]
            n495 = property class="Path"(reference=w1469, error in=w1468, "Value"=w1467) -> (reference out=w1465:refnum<vi>, error out=w1466:errorcluster)
            n496 = Close Reference(reference=w1465, error in (no error)=w1466) -> (error out=w1463:errorcluster)
            n497 = call "Display Update During Macro Load.vi"("Macro Error IN"=w1461, "New Index IN"=w1460, "error in (no error)"=w1463, "Macro Array IN"=w1464, "Previous Index IN"=w1460, "UI control refnums"=w1448) -> ("error out"=w1450:errorcluster, "Macro Error OUT"=w1462:bool)  [unwired: 3 in, 1 out]
            n498 = call "TimingEstimate_Valid_Invalid_Update.vi"("Command"=enum16{"Valid", "Invalid"}."Valid", "error in (no error)"=w1450, "UI control refnums"=w1448) -> ("error out"=w1449:errorcluster)  [unwired: 8 in]
          }
        }
      }
      event "File Operation Cluster.Load Macro": Value Change {
        # "Cancelled by user?"
        n499 = event-data() -> ()  [unwired: 1 in, 1 out]
        n500 = call "FGV_MacroCore.vi"("MacroFGV_Commands"=FGV_MacroCore_Commands."Load macro from file", "Error In"=w1510) -> ("Error Out"=w1512:errorcluster, "File IO Cancelled/Error?"=w1507:bool, "Macro String Array"=w1501:string[], "Saved Macro Path"=w1495:path)  [unwired: 5 in, 1 out]
        n501 = case shown="False" w1507 {
          tunnel: w1512 -> [w1529 w1552]
          tunnel: [w1519 w1552] -> w1511
          tunnel: w1501 -> [w1532 _]
          tunnel: [w1534 w1553] -> w1506
          tunnel: w1505 -> [w1537 w1553]
          tunnel: w1504 -> [w1514 _]
          tunnel: [w1535 w1551] -> w1500
          tunnel: w1499 -> [w1536 w1551]
          tunnel: w1495 -> [w1530 _]
          tunnel: w1493 -> [w1518 _]
          frame False {
            # "Any changes to macro?\nIf yes, indicate to user as unsaved"
            n502 = Unbundle By Name(w1514) -> ("Macro File Path"=w1531:refnum<vi>)
            n503 = property class="Path"(reference=w1531, error in=w1529, "Value"=w1530) -> (reference out=w1527:refnum<vi>, error out=w1528:errorcluster)
            n504 = Close Reference(reference=w1527, error in (no error)=w1528) -> (error out=w1526:errorcluster)
            n505 = call "Stage Position Safety.vi"("error in (no error)"=w1526, "Macro Array IN"=w1532) -> ("error out"=w1521:errorcluster, "Line Modified ?"=w1525:bool[], "Modified Array OUT"=w1533:string[])  [unwired: 7 in]
            n506 = disable-structure shown="Enabled" {
              disable-tunnel: [w1540 _] -> w1520
              disable-tunnel: w1521 -> [w1539 _]
              disable-tunnel: w1518 -> [w1538 _]
              frame Enabled {
                n507 = call <vilib>:"Create Cursor From File.vi"("error in (no error)"=w1539, "cursor file"=w1538) -> ("error out"=w1541:errorcluster, "cursor ID"=w1542:refnum<k1>)  [unwired: 8 in]
                n508 = call <vilib>:"Set Busy.vi"("error in (no error)"=w1541, "cursor ID"=w1542) -> ("error out"=w1540:errorcluster)  [unwired: 8 in, 1 out]
              }
              frame Disabled {
              }
            }
            n509 = Or Array Elements(Boolean array=w1525) -> (logical OR=w1524:bool)
            n510 = call "Display Update During Macro Load.vi"("Macro Error IN"=w1536, "New Index IN"=0, "error in (no error)"=w1520, "Macro Array IN"=w1533, "Previous Index IN"=w1537, "UI control refnums"=w1514) -> ("error out"=w1523:errorcluster, "New Index OUT"=w1534:i32, "Macro Error OUT"=w1535:bool)  [unwired: 3 in]
            n511 = case shown="False" w1524 {
              tunnel: w1523 -> [w1545 w1549]
              tunnel: w1514 -> [w1544 w1548]
              tunnel: [w1543 w1547] -> w1516
              frame True {
                n512 = call "SavedStatusUpdate.vi"("Options"=enum16{"Unsaved", "Saved"}."Unsaved", "error in (no error)"=w1545, "UI control refnums"=w1544) -> ("error out"=w1543:errorcluster)  [unwired: 8 in]
              }
              frame False {
                n513 = call "SavedStatusUpdate.vi"("Options"=enum16{"Unsaved", "Saved"}."Saved", "error in (no error)"=w1549, "UI control refnums"=w1548) -> ("error out"=w1547:errorcluster)  [unwired: 8 in]
              }
            }
            n514 = call "TimingEstimate_Valid_Invalid_Update.vi"("Command"=enum16{"Valid", "Invalid"}."Invalid", "error in (no error)"=w1516, "UI control refnums"=w1514) -> ("error out"=w1515:errorcluster)  [unwired: 8 in]
            n515 = call <vilib>:"Unset Busy.vi"("error in (no error)"=w1515) -> ("error out"=w1519:errorcluster)  [unwired: 10 in]
          }
          frame True {
            # "Load operation cancelled by user - Keep index unchanged"
          }
        }
      }
      event "MacroFile\nPath": Value Change {
        n516 = event-data() -> ("NewVal"=w1557:path)  [unwired: 1 in]
        n517 = disable-structure shown="Disabled" {
          disable-tunnel: [w1578 w1608] -> w1560
          disable-tunnel: w1558 -> [w1577 _]
          disable-tunnel: w1557 -> [w1573 _]
          disable-tunnel: w1556 -> [w1572 w1608]
          disable-tunnel: w1555 -> [w1570 w1609]
          disable-tunnel: [w1569 w1609] -> w1554
          frame Disabled {
            n518 = call "File IO operation status.vi"("File Path"=w1573, "check if valid extension (Specify Extension Type)"=TRUE, "expected extension type"="sscr" ("string"), "error in (no error)"=w1572) -> ("File Operation Status"=w1574:T48, "error out"=w1571:errorcluster)  [unwired: 10 in]
            n519 = case shown="\"Success\"" w1574 {
              tunnel: w1573 -> [_ w1590]
              tunnel: w1571 -> [w1587 w1593]
              tunnel: [w1579 w1592] -> w1578
              tunnel: w1577 -> [w1583 w1591]
              tunnel: w1570 -> [w1580 w1588]
              tunnel: [w1580 w1590] -> w1569
              frame Default {
                n520 = Unbundle By Name(w1583) -> ("Macro File Path"=w1582:refnum<vi>)
                n521 = call <vilib>:"Clear Errors.vi"("error in (no error)"=w1587) -> ("error out"=w1584:errorcluster)  [unwired: 6 in]
                n522 = property class="Path"(reference=w1582, error in=w1584, "Value"=w1580) -> (reference out=w1585:refnum<vi>, error out=w1581:errorcluster)
                n523 = Close Reference(reference=w1585, error in (no error)=w1581) -> (error out=w1579:errorcluster)
                n524 = One Button Dialog(message="Invalid Path!") -> ()  [unwired: 1 in, 1 out]
              }
              frame "Success" {
                n525 = call "MacroFileIO.vi"("New Path IN"=w1590, "MacroFileIO_Command"=MacroFileIO_Commands."Save As", "Error In"=w1593) -> ("Error Out"=w1589:errorcluster)  [unwired: 7 in, 5 out]
                n526 = case shown="Error" w1589 {
                  tunnel: w1589 -> [w1597 w1607]
                  tunnel: [w1596 w1599] -> w1592
                  tunnel: w1591 -> [w1595 w1605]
                  tunnel: w1588 -> [_ w1602]
                  frame No Error {
                    n527 = call "SavedStatusUpdate.vi"("Options"=enum16{"Unsaved", "Saved"}."Saved", "error in (no error)"=w1597, "UI control refnums"=w1595) -> ("error out"=w1596:errorcluster)  [unwired: 8 in]
                  }
                  frame Error {
                    n528 = call <vilib>:"Clear Errors.vi"("error in (no error)"=w1607) -> ("error out"=w1604:errorcluster)  [unwired: 6 in]
                    n529 = Unbundle By Name(w1605) -> ("Macro File Path"=w1603:refnum<vi>)
                    n530 = property class="Path"(reference=w1603, error in=w1604, "Value"=w1602) -> (reference out=w1600:refnum<vi>, error out=w1601:errorcluster)
                    n531 = Close Reference(reference=w1600, error in (no error)=w1601) -> (error out=w1599:errorcluster)
                    n532 = One Button Dialog(message="Invalid Path!") -> ()  [unwired: 1 in, 1 out]
                  }
                }
              }
            }
          }
          frame Enabled {
          }
        }
      }
      event "Copy Button": Value Change {
        n533 = event-data() -> ()  [unwired: 1 in, 1 out]
        n534 = call "reg unreg for MacroGUI.vi"("T for reg, F for unreg"=FALSE, "error in (no error)"=w1620, "event cluster"=w1614, "Event Registration Refnum"=w1619) -> ("error out"=w1618:errorcluster, "Event Registration Refnum Out"=w1615:refnum<event-registration>)  [unwired: 6 in]
        n535 = call "MacroFileIO.vi"("MacroFileIO_Command"=MacroFileIO_Commands."Save As", "Error In"=w1618) -> ("File IO Cancelled/NotFound?"=w1624:bool, "Macro File Path OUT"=w1623:path, "Error Out"=w1625:errorcluster)  [unwired: 8 in, 3 out]
        n536 = case shown="False" w1624 {
          tunnel: w1625 -> [w1639 w1648]
          tunnel: [w1640 w1648] -> w1616
          tunnel: w1628 -> [w1641 _]
          tunnel: w1627 -> [_ w1649]
          tunnel: w1623 -> [w1638 _]
          tunnel: [w1638 w1649] -> w1622
          tunnel: [FALSE w1647] -> w1611
          tunnel: w1610 -> [_ w1647]
          frame False {
            n537 = Unbundle By Name(w1641) -> ("Macro File Path"=w1646:refnum<vi>)
            n538 = property class="Path"(reference=w1646, error in=w1639, "Value"=w1638) -> (reference out=w1644:refnum<vi>, error out=w1645:errorcluster)
            n539 = Close Reference(reference=w1644, error in (no error)=w1645) -> (error out=w1642:errorcluster)
            n540 = call "SavedStatusUpdate.vi"("Options"=enum16{"Unsaved", "Saved"}."Saved", "error in (no error)"=w1642, "UI control refnums"=w1641) -> ("error out"=w1640:errorcluster)  [unwired: 8 in]
          }
          frame True {
          }
        }
        n541 = call "reg unreg for MacroGUI.vi"("T for reg, F for unreg"=TRUE, "error in (no error)"=w1616, "event cluster"=w1614, "Event Registration Refnum"=w1615) -> ("error out"=w1612:errorcluster, "Event Registration Refnum Out"=w1613:refnum<event-registration>)  [unwired: 6 in]
      }
      event "Preview Macro": Value Change {
        n542 = event-data() -> ("NewVal"=w1657:bool)  [unwired: 1 in]
        n543 = case shown="True" w1657 {
          tunnel: w1660 -> [w1697 w1717]
          tunnel: w1659 -> [w1696 w1721]
          tunnel: [w1672 w1708] -> w1658
          tunnel: w1656 -> [w1671 w1720]
          tunnel: w1655 -> [w1673 w1719]
          tunnel: [w1673 w1719] -> w1654
          tunnel: w1653 -> [_ w1714]
          tunnel: w1652 -> [w1670 w1713]
          tunnel: [w1670 w1712] -> w1651
          frame False {
            # "If the current preview is a scan settings update,, programatically trigger a 'Cancel Edit.\n- So that, Update guide close3s and other cleanup happens"
            # "If 2D LineScan, clear the ROI and change tab to 2D frame scan (to deactivate linescan mode during the next press of focus)"
            # "Clear any ROI that gas\nbeen drawn (for LineScan)"
            n544 = call "HFG_Core.vi"("HFG Commands"=HFG_Commands."Set", "Error In"=w1697, "Heartbeat state IN"=Heartbeat_States."Cancelled" ("Run state IN"), "VI Name (Calling VIs name by default)"=w1696) -> ("Error Out"=w1692:errorcluster)  [unwired: 4 in, 3 out]
            n545 = call "GFG_core.vi"("Variable Name in"="Preview.Mode", "Variant in"=FALSE, "error in (no error)"=w1692, "Action"=enum16{"Init", "Set", "Get", "Clear"}."Set") -> ("error out"=w1689:errorcluster)  [unwired: 9 in, 6 out]
            n546 = One Button Dialog(message="Preview Cancelled!") -> ()  [unwired: 1 in, 1 out]
            n547 = Unbundle By Name(w1671) -> ("Preview Macro"=w1686:refnum<vi>, "Execute Macro"=w1669:refnum<vi>)
            n548 = call "Manage UI and GFG states during settings file edit.vi"("Commands"=Update_Scan_Settings_Commands."Finalise Update", "Error In"=w1689, "UI control refnums"=w1671) -> ("Error Out"=w1687:errorcluster)  [unwired: 8 in]
            n549 = Build Array(w1686, w1669) -> (w1685:refnum<vi>[])
            n550 = call "Draw ROI on Line Scan Display.vi"("Draw ROI on Line Scan Display_Command"=Draw_ROI_on_Line_Scan_Display_Command."Clear ROI", "error in (no error)"=w1687) -> ("error out"=w1683:errorcluster)  [unwired: 9 in]
            n551 = call "UI Control and Indicator properties.vi"("Enable Command"=UI_Control_and_Indicator_properties_Commands."Enable", "Error In"=w1683, "Control Refnums"=w1685) -> ("Error Out"=w1674:errorcluster)  [unwired: 8 in]
            n552 = call "FGV_MacroCore.vi"("MacroFGV_Commands"=FGV_MacroCore_Commands."Get Array", "Error In"=w1674) -> ("Error Out"=w1679:errorcluster, "Macro String Array"=w1681:string[])  [unwired: 5 in, 3 out]
            n553 = Index Array(array=w1681, index=w1673) -> (element=w1680:string)
            n554 = call "Decompose Command String.vi"("Error In"=w1679, "Command IN"=w1680) -> ("Error Out"=w1678:errorcluster, "Action"=w1675:string)  [unwired: 6 in, 2 out]
            n555 = call "Macro Action String to Action and Settings Enum.vi"("error in (no error)"=w1678, "Action String IN"=w1675) -> ("error out"=w1677:errorcluster, "Action Enum OUT"=w1676:T49)  [unwired: 6 in, 2 out]
            n556 = case shown="\"2D.Frame.Scan\", \"2D.Line.Scan\", \"Z.Stack\", \"Fast.Z\"" w1676 {
              tunnel: w1677 -> [w1704 w1707]
              tunnel: [w1701 w1707] -> w1672
              tunnel: w1671 -> [w1706 _]
              frame "2D.Frame.Scan", "2D.Line.Scan", "Z.Stack", "Fast.Z" {
                n557 = Unbundle By Name(w1706) -> ("Cancel Settings"=w1705:refnum<vi>)
                n558 = property class="Bool"(reference=w1705, error in=w1704, "Val(Sgnl)"=TRUE) -> (reference out=w1702:refnum<vi>, error out=w1703:errorcluster)
                n559 = Close Reference(reference=w1702, error in (no error)=w1703) -> (error out=w1701:errorcluster)
              }
              frame Default {
              }
            }
          }
          frame True {
            # "ISSUE!!\nThere is comms\nbreakdown betwn LOOP Mngr and GUI if unregistered"
            n560 = disable-structure shown="Enabled" {
              disable-tunnel: w1717 -> [w1726 _]
              disable-tunnel: [w1725 _] -> w1716
              disable-tunnel: w1714 -> [w1724 _]
              disable-tunnel: w1713 -> [w1723 _]
              disable-tunnel: [w1722 _] -> w1711
              frame Enabled {
                n561 = call "reg unreg for MacroGUI.vi"("T for reg, F for unreg"=FALSE, "error in (no error)"=w1726, "event cluster"=w1724, "Event Registration Refnum"=w1723) -> ("error out"=w1725:errorcluster, "Event Registration Refnum Out"=w1722:refnum<event-registration>)  [unwired: 6 in]
              }
              frame Disabled {
              }
            }
            n562 = call "Dialog Preview Message.vi"("error in (no error)"=w1716) -> ("error out"=w1710:errorcluster, "Cancelled?"=w1718:bool)  [unwired: 9 in]
            n563 = call "reg unreg for MacroGUI.vi"("T for reg, F for unreg"=TRUE, "error in (no error)"=w1710, "event cluster"=w1714, "Event Registration Refnum"=w1711) -> ("error out"=w1709:errorcluster, "Event Registration Refnum Out"=w1712:refnum<event-registration>)  [unwired: 6 in]
            n564 = case shown="False" w1718 {
              tunnel: w1721 -> [w1754 _]
              tunnel: w1720 -> [w1734 w1764]
              tunnel: [w1729 w1762] -> w1708
              tunnel: w1709 -> [w1728 w1762]
              frame False {
                n565 = Unbundle By Name(w1734) -> ("Execute Macro"=w1732:refnum<vi>)
                n566 = call "GFG_core.vi"("Variable Name in"="Preview.Mode", "Variant in"=TRUE, "error in (no error)"=w1728, "Action"=enum16{"Init", "Set", "Get", "Clear"}."Set") -> ("error out"=w1741:errorcluster)  [unwired: 9 in, 6 out]
                n567 = call "FGV_MacroCore.vi"("MacroFGV_Commands"=FGV_MacroCore_Commands."Get Array", "Error In"=w1741) -> ("Error Out"=w1746:errorcluster, "Macro String Array"=w1736:string[])  [unwired: 5 in, 3 out]
                n568 = call "Macro_Text Array to Instruction and Argument array.vi"("Error In"=w1746, "Macro Array IN"=w1736) -> ("Error Out"=w1745:errorcluster, "Argument List (Txt)"=w1742:string[], "Action List (Txt)"=w1743:string[])  [unwired: 7 in]
                n569 = for {
                  shift-right: [w1758] -> w1749
                  shift-left: w1745 -> [w1758]
                  tunnel: [w1755] -> w1744 mode=indexing
                  tunnel: w1743 -> [w1757] mode=indexing
                  tunnel: w1742 -> [w1756] mode=indexing
                  n570 = Concatenate Strings(w1757, w1756) -> (w1755:string)
                }
                n571 = call "GFG_core.vi"("Variable Name in"="Macro", "Variant in"=w1744, "error in (no error)"=w1749, "Action"=enum16{"Init", "Set", "Get", "Clear"}."Set") -> ("error out"=w1737:errorcluster)  [unwired: 9 in, 6 out]
                n572 = call "MacroExecution and Timing.vi"("MacroExecution and Timing Command"=Macro_Execution_and_Timing_Commands."Initialize (Update FGV & Rst Idx)" ("MacroExecution Command"), "Error In"=w1737, "Macro IN"=w1736) -> ("Error Out"=w1735:errorcluster)  [unwired: 3 in, 5 out]
                n573 = call "HFG_Core.vi"("HFG Commands"=HFG_Commands."Set", "Error In"=w1735, "Heartbeat state IN"=Heartbeat_States."Instruction Issued" ("Run state IN"), "VI Name (Calling VIs name by default)"=w1754) -> ("Error Out"=w1730:errorcluster)  [unwired: 4 in, 3 out]
                n574 = Build Array(w1732) -> (w1731:refnum<vi>[])
                n575 = call "UI Control and Indicator properties.vi"("Enable Command"=UI_Control_and_Indicator_properties_Commands."Disable and Grey", "Error In"=w1730, "Control Refnums"=w1731) -> ("Error Out"=w1729:errorcluster)  [unwired: 8 in]
              }
              frame True {
                n576 = Unbundle By Name(w1764) -> ("Preview Macro"=w1763:refnum<vi>)
                n577 = property class="Bool (strict)"(reference=w1763, error in=w1762, "Val(Sgnl)"=FALSE) -> (reference out=w1759:refnum<vi>, error out=w1760:errorcluster)
                n578 = Close Reference(reference=w1759, error in (no error)=w1760) -> ()  [unwired: 1 out]
              }
            }
          }
        }
      }
      event "File Operation Cluster.Save Macro": Value Change {
        n579 = event-data() -> ()  [unwired: 1 in, 1 out]
        n580 = call "MacroFileIO.vi"("MacroFileIO_Command"=MacroFileIO_Commands."Save" ("FGV_MacroFileIO_Command"), "Error In"=w1772) -> ("File IO Cancelled/NotFound?"=w1771:bool, "Macro File Path OUT"=w1767:path, "Error Out"=w1770:errorcluster)  [unwired: 8 in, 3 out]
        n581 = case shown="False" w1771 {
          tunnel: w1770 -> [w1790 w1793]
          tunnel: [w1786 w1793] -> w1769
          tunnel: w1768 -> [w1789 _]
          tunnel: w1767 -> [w1783 _]
          tunnel: [FALSE w1792] -> w1766
          tunnel: w1765 -> [_ w1792]
          frame False {
            n582 = Unbundle By Name(w1789) -> ("Macro File Path"=w1788:refnum<vi>)
            n583 = call "SavedStatusUpdate.vi"("Options"=enum16{"Unsaved", "Saved"}."Saved", "error in (no error)"=w1790, "UI control refnums"=w1789) -> ("error out"=w1787:errorcluster)  [unwired: 8 in]
            n584 = property class="Path"(reference=w1788, error in=w1787, "Value"=w1783) -> (reference out=w1784:refnum<vi>, error out=w1785:errorcluster)
            n585 = Close Reference(reference=w1784, error in (no error)=w1785) -> (error out=w1786:errorcluster)
          }
          frame True {
          }
        }
      }
      event Value Change {
        n586 = event-data() -> ()  [unwired: 1 in, 1 out]
        n587 = call <vilib>:"Create Cursor From File.vi"("error in (no error)"=w1802, "cursor file"=w1799) -> ("error out"=w1801:errorcluster, "cursor ID"=w1803:refnum<k1>)  [unwired: 8 in]
        n588 = call <vilib>:"Set Busy.vi"("error in (no error)"=w1801, "cursor ID"=w1803) -> ("error out"=w1800:errorcluster)  [unwired: 8 in, 1 out]
        n589 = Unbundle By Name(w1823) -> ("Created Macro"=w1816:refnum<vi>, "Params Table"=w1796:refnum<vi>)
        n590 = Not(x="Delete Button") -> (.not. x?=w1795:T3)
        n591 = call "Tree_GetAll.vi"("Error In"=w1800, "Tree Refnum IN"=w1816) -> ("Error Out"=w1818:errorcluster, "Tags"=w1811:string[], "Tree Refnum OUT"=w1817:refnum<vi>)  [unwired: 6 in, 1 out]
        n592 = local write "Delete Button"(w1795) -> ()
        n593 = Array Size(array=w1811) -> (size(s)=w1822:i32)
        n594 = Greater Than 0?(x=w1822) -> (x > 0?=w1821:bool)
        n595 = case shown="True" w1821 {
          tunnel: w1823 -> [_ w1828]
          tunnel: w1818 -> [w1827 w1837]
          tunnel: [w1827 w1833] -> w1798
          tunnel: w1820 -> [w1826 w1838]
          tunnel: [w1826 w1835] -> w1819
          tunnel: w1817 -> [_ _]
          tunnel: w1796 -> [_ _]
          tunnel: w1811 -> [_ _]
          tunnel: w1810 -> [w1825 _]
          tunnel: [w1825 w1836] -> w1809
          tunnel: w1805 -> [w1824 _]
          tunnel: [w1824 TRUE ("Any Error?")] -> w1804
          frame False {
          }
          frame True {
            n596 = call "Delete Operation and Display Update.vi"("error in (no error)"=w1837, "Previous Index IN"=w1838, "UI control refnums"=w1828) -> ("error out"=w1830:errorcluster, "New Index OUT"=w1835:i32, "Macro Error OUT"=w1836:bool)  [unwired: 6 in]
            n597 = call "TimingEstimate_Valid_Invalid_Update.vi"("Command"=enum16{"Valid", "Invalid"}."Invalid", "error in (no error)"=w1830, "UI control refnums"=w1828) -> ("error out"=w1829:errorcluster)  [unwired: 8 in]
            n598 = call "SavedStatusUpdate.vi"("Options"=enum16{"Unsaved", "Saved"}."Unsaved", "error in (no error)"=w1829, "UI control refnums"=w1828) -> ("error out"=w1833:errorcluster)  [unwired: 8 in]
          }
        }
        n599 = call <vilib>:"Unset Busy.vi"("error in (no error)"=w1798) -> ("error out"=w1797:errorcluster)  [unwired: 10 in]
      }
      event Value Change {
        n600 = event-data() -> ()  [unwired: 1 in, 1 out]
        n601 = Unbundle By Name(w1846) -> ("Created Macro"=w1845:refnum<vi>)
        n602 = call "Tree_GetAll.vi"("Tree Refnum IN"=w1845) -> ("Tags"=w1844:string[], "Tree Refnum OUT"=w1843:refnum<vi>)  [unwired: 7 in, 2 out]
        n603 = call "reg unreg for MacroGUI.vi"("T for reg, F for unreg"=FALSE, "error in (no error)"=w1857, "event cluster"=w1850, "Event Registration Refnum"=w1859) -> ("error out"=w1856:errorcluster, "Event Registration Refnum Out"=w1851:refnum<event-registration>)  [unwired: 6 in]
        n604 = Index Array(array=w1844, index=w1842) -> (element=w1841:string)
        n605 = call "Check if specified tag is inside a Preset.vi"("Tag to check"=w1841, "Tree Refnum"=w1843) -> ("Specified tag is part of a Preset?"=w1847:bool)  [unwired: 6 in, 3 out]
        n606 = case shown="False" w1847 {
          tunnel: w1865 -> [w1889 w2151]
          tunnel: [w1888 w2151] -> w1864
          tunnel: [w1884 w2150] -> w1860
          tunnel: w1846 -> [w1876 _]
          tunnel: w1856 -> [w1875 w2153]
          tunnel: [w1874 w2153] -> w1854
          tunnel: w1849 -> [w1873 w2152]
          tunnel: [w1872 w2152] -> w1848
          tunnel: w1842 -> [w1871 w2150]
          frame False {
            n607 = call "FGV_MacroCore.vi"("MacroFGV_Commands"=FGV_MacroCore_Commands."Get Array", "Error In"=w1875) -> ("Error Out"=w1885:errorcluster, "Macro String Array"=w1886:string[])  [unwired: 5 in, 3 out]
            n608 = Index Array(array=w1886, index=w1871) -> (element=w1883:string)
            n609 = call "Decompose Command String.vi"("Error In"=w1885, "Command IN"=w1883) -> ("Error Out"=w1881:errorcluster, "Parameter Table"=w1882:string[][], "Action"=w1880:string)  [unwired: 6 in, 1 out]
            n610 = call "Macro Action String to Action and Settings Enum.vi"("error in (no error)"=w1881, "Action String IN"=w1880) -> ("error out"=w1878:errorcluster, "Setting File Type OUT"=w1877:T39, "Action Enum OUT"=w1879:T49)  [unwired: 6 in, 1 out]
            n611 = case shown="\"2D.Frame.Scan\", \"Fast.Z\"" w1879 {
              tunnel: w1878 -> [w1982 w1989 w1992 w2002 w2026 w2069 w2102 w2114 w2131 w2147]
              tunnel: [w1983 w1988 w1992 w1995 w2015 w2065 w2097 w2105 w2124 w2146] -> w1892
              tunnel: [w1981 w1987 TRUE ("Cancelled?") w1998 TRUE ("Cancelled?") TRUE ("Cancelled?") TRUE ("Cancelled?") TRUE ("Cancelled?") TRUE ("Cancelled?") w2145] -> w1891
              tunnel: [w1980 w1986 _ w2001 _ _ _ _ _ w2144] -> w1890
              tunnel: w1876 -> [_ _ _ w1994 w2021 w2066 w2101 w2113 w2128 _]
              tunnel: w1883 -> [_ _ _ _ _ _ w2099 w2111 w2132 _]
              tunnel: w1882 -> [_ w1985 _ _ _ _ _ _ _ _]
              tunnel: w1877 -> [_ _ _ _ _ _ w2096 w2109 w2126 _]
              tunnel: w1871 -> [w1979 w1984 w1990 w1993 w2022 w2067 w2095 w2104 w2123 w2143]
              tunnel: [w1979 w1984 w1990 w1993 w2023 w2068 w2095 w2104 w2123 w2143] -> w1870
              frame "Pause" {
                # "Pause"
                n612 = call "Dialog_Enter Wait Duration.vi"("Error In"=w1982) -> ("Error Out"=w1983:errorcluster, "Cancelled?"=w1981:bool, "Macro Command"=w1980:string)  [unwired: 8 in]
              }
              frame "Generic" {
                # "Generic"
                n613 = call "Dialog_Enter Generic.vi"("Error In"=w1989, "Parameter Table"=w1985) -> ("Error Out"=w1988:errorcluster, "Cancelled?"=w1987:bool, "Generic Command"=w1986:string)  [unwired: 7 in]
              }
              frame Default {
                # "Default - Do nothing"
              }
              frame "Move.To.Position" {
                # "Move.To.Position"
                # "Cancelled\nand Preview?"
                n614 = call "GFGbooleanGet.vi"("Variable Name in"="Preview.Mode") -> ("Boolean Value OUT"=w1997:bool)  [unwired: 9 in, 1 out]
                n615 = call "Dialog_Enter Stage Position.vi"("Error In"=w2002) -> ("Error Out"=w1996:errorcluster, "Cancelled?"=w1998:bool, "Macro Command"=w2001:string)  [unwired: 8 in]
                n616 = And(x=w1998, y=w1997) -> (x .and. y?=w1999:bool)
                n617 = case shown="True" w1999 {
                  tunnel: w1996 -> [w2003 w2008]
                  tunnel: [w2003 w2007] -> w1995
                  tunnel: w1994 -> [_ w2006]
                  frame False {
                  }
                  frame True {
                    n618 = Unbundle By Name(w2006) -> ("Preview Macro"=w2005:refnum<vi>)
                    n619 = disable-structure shown="Disabled" {
                      disable-tunnel: w2008 -> [w2010 w2014]
                      disable-tunnel: [w2009 w2014] -> w2007
                      frame Disabled {
                        n620 = call "GFG_core.vi"("Variable Name in"="Settings.Confirmed", "Variant in"=TRUE, "error in (no error)"=w2010, "Action"=enum16{"Init", "Set", "Get", "Clear"}."Set") -> ("error out"=w2009:errorcluster)  [unwired: 9 in, 6 out]
                      }
                      frame Enabled {
                      }
                    }
                    n621 = property class="Bool (strict)"(reference=w2005, "Val(Sgnl)"=FALSE) -> ()  [unwired: 1 in, 2 out]
                  }
                }
              }
              frame "Slow.Z" {
                # "Is there a 2.D.Frame Scan?"
                n622 = Unbundle By Name(w2021) -> ("Created Macro"=w2020:refnum<vi>, "Params Table"=w2019:refnum<vi>)
                n623 = Unbundle By Name(w2021) -> ("Created Macro"=w2016:refnum<vi>, "Params Table"=w2028:refnum<vi>)
                n624 = Build Array(w2019) -> (w2017:refnum<vi>[])
                n625 = Build Array(w2020) -> (w2018:refnum<vi>[])
                n626 = call "Dialog_Configure Slow Z.vi"("Index of Slow.Z"=w2022, "Tbl Refnum"=w2028, "Tree Refnum"=w2016) -> ("Empty Slow.Z?"=w2024:bool, "Index of 2DFrame.Scan"=w2025:i32, "Updated Macro String Array"=w2027:string[])  [unwired: 6 in]
                n627 = case shown="False" w2024 {
                  tunnel: w2027 -> [w2043 _]
                  tunnel: w2021 -> [w2042 _]
                  tunnel: w2026 -> [w2032 w2053]
                  tunnel: [w2041 w2053] -> w2015
                  tunnel: w2025 -> [w2035 _]
                  tunnel: [w2035 w2052] -> w2023
                  tunnel: w2022 -> [w2039 w2052]
                  tunnel: w2018 -> [w2036 _]
                  tunnel: w2017 -> [w2037 _]
                  frame False {
                    n628 = Index Array(array=w2043, index=w2035) -> (element=w2031:string)
                    n629 = call "Prepare for a Scan_Load Settings.vi"("error in (no error)"=w2032, "Command IN"=w2031) -> ("error out"=w2033:errorcluster)  [unwired: 9 in]
                    n630 = call "FormatTree&TableStyle.vi"("Format Command"=FormatTree&TableStyle_Commands."Uncolour Row", "Row Index"=w2039, "Array of Table references"=w2037, "Array of Tree references"=w2036) -> ("Error Out"=w2034:errorcluster)  [unwired: 7 in]
                    n631 = call "Wait till all GFG events stop_for fixed duration.vi"("error in (no error)"=w2033) -> ("error out"=w2030:errorcluster)  [unwired: 10 in]
                    n632 = disable-structure shown="Enabled" {
                      disable-tunnel: w2042 -> [w2048 _]
                      disable-tunnel: w2031 -> [w2047 _]
                      disable-tunnel: w2030 -> [w2046 w2051]
                      disable-tunnel: [w2045 w2051] -> w2041
                      frame Disabled {
                        n633 = call "Manage UI and GFG states during settings file edit.vi"("Commands"=Update_Scan_Settings_Commands."Initiate Update", "Error In"=w2046, "Command String IN"=w2047, "UI control refnums"=w2048) -> ("Error Out"=w2050:errorcluster)  [unwired: 7 in]
                        n634 = call "Dynamically Call_Settings Info dialog VI.vi"("error in (no error)"=w2050, "Setting File Type"=Setting_File_Types."2D.Frame.Scan.Settings") -> ("error out"=w2045:errorcluster)  [unwired: 9 in]
                      }
                      frame Enabled {
                      }
                    }
                    n635 = call "FormatTree&TableStyle.vi"("Format Command"=FormatTree&TableStyle_Commands."Colour Row", "Error In"=w2034, "Row Index"=w2035, "Array of Table references"=w2037, "Array of Tree references"=w2036) -> ()  [unwired: 6 in, 1 out]
                  }
                  frame True {
                  }
                }
              }
              frame "Tiling" {
                # "Is there a 2.D.Frame Scan?"
                n636 = Unbundle By Name(w2066) -> ("Created Macro"=w2061:refnum<vi>, "Params Table"=w2060:refnum<vi>)
                n637 = Unbundle By Name(w2066) -> ("Created Macro"=w2057:refnum<vi>, "Params Table"=w2064:refnum<vi>)
                n638 = call "Dialog_Configure Tiling.vi"("Index of Tiling"=w2067, "Tbl Refnum"=w2064, "Tree Refnum"=w2057) -> ("Empty Array/Cancelled?"=w2055:bool, "Index of 2DFrame.Scan"=w2062:i32, "Updated Macro String Array"=w2063:string[], "Skip configure 2D settings?"=w2056:bool)  [unwired: 5 in]
                n639 = Build Array(w2060) -> (w2058:refnum<vi>[])
                n640 = Build Array(w2061) -> (w2059:refnum<vi>[])
                n641 = Or(x=w2055, y=w2056) -> (x .or. y?=w2054:bool)
                n642 = case shown="False" w2054 {
                  tunnel: w2063 -> [w2084 _]
                  tunnel: w2066 -> [w2083 _]
                  tunnel: w2069 -> [w2073 w2094]
                  tunnel: [w2082 w2094] -> w2065
                  tunnel: w2062 -> [w2076 _]
                  tunnel: [w2076 w2093] -> w2068
                  tunnel: w2067 -> [w2080 w2093]
                  tunnel: w2059 -> [w2077 _]
                  tunnel: w2058 -> [w2078 _]
                  frame False {
                    n643 = Index Array(array=w2084, index=w2076) -> (element=w2072:string)
                    n644 = call "Prepare for a Scan_Load Settings.vi"("error in (no error)"=w2073, "Command IN"=w2072) -> ("error out"=w2074:errorcluster)  [unwired: 9 in]
                    n645 = call "FormatTree&TableStyle.vi"("Format Command"=FormatTree&TableStyle_Commands."Uncolour Row", "Row Index"=w2080, "Array of Table references"=w2078, "Array of Tree references"=w2077) -> ("Error Out"=w2075:errorcluster)  [unwired: 7 in]
                    n646 = call "Wait till all GFG events stop_for fixed duration.vi"("error in (no error)"=w2074) -> ("error out"=w2071:errorcluster)  [unwired: 10 in]
                    n647 = disable-structure shown="Enabled" {
                      disable-tunnel: w2083 -> [w2089 _]
                      disable-tunnel: w2072 -> [w2088 _]
                      disable-tunnel: w2071 -> [w2087 w2092]
                      disable-tunnel: [w2086 w2092] -> w2082
                      frame Disabled {
                        n648 = call "Manage UI and GFG states during settings file edit.vi"("Commands"=Update_Scan_Settings_Commands."Initiate Update", "Error In"=w2087, "Command String IN"=w2088, "UI control refnums"=w2089) -> ("Error Out"=w2091:errorcluster)  [unwired: 7 in]
                        n649 = call "Dynamically Call_Settings Info dialog VI.vi"("error in (no error)"=w2091, "Setting File Type"=Setting_File_Types."2D.Frame.Scan.Settings") -> ("error out"=w2086:errorcluster)  [unwired: 9 in]
                      }
                      frame Enabled {
                      }
                    }
                    n650 = call "FormatTree&TableStyle.vi"("Format Command"=FormatTree&TableStyle_Commands."Colour Row", "Error In"=w2075, "Row Index"=w2076, "Array of Table references"=w2078, "Array of Tree references"=w2077) -> ()  [unwired: 6 in, 1 out]
                  }
                  frame True {
                  }
                }
              }
              frame "2D.Frame.Scan", "Fast.Z" {
                n651 = call "Manage UI and GFG states during settings file edit.vi"("Commands"=Update_Scan_Settings_Commands."Initiate Update", "Error In"=w2102, "Command String IN"=w2099, "UI control refnums"=w2101) -> ("Error Out"=w2098:errorcluster)  [unwired: 7 in]
                n652 = call "Dynamically Call_Settings Info dialog VI.vi"("error in (no error)"=w2098, "Setting File Type"=w2096) -> ("error out"=w2097:errorcluster)  [unwired: 9 in]
              }
              frame "Z.Stack" {
                n653 = call "Manage UI and GFG states during settings file edit.vi"("Commands"=Update_Scan_Settings_Commands."Initiate Update", "Error In"=w2114, "Command String IN"=w2111, "UI control refnums"=w2113) -> ("Error Out"=w2110:errorcluster)  [unwired: 7 in]
                n654 = call "Dynamically Call_Settings Info dialog VI.vi"("error in (no error)"=w2110, "Setting File Type"=w2109) -> ("error out"=w2106:errorcluster)  [unwired: 9 in]
                n655 = call "GFGbooleanGet.vi"("Variable Name in"="Preview.Mode") -> ("Boolean Value OUT"=w2107:bool)  [unwired: 9 in, 1 out]
                n656 = case shown="True" w2107 {
                  tunnel: w2106 -> [w2116 w2118]
                  tunnel: [w2116 w2117] -> w2105
                  frame False {
                  }
                  frame True {
                    n657 = call "GFG_core.vi"("Variable Name in"="move.to.z.stack..start.plane", "Variant in"=TRUE, "error in (no error)"=w2118, "Action"=enum16{"Init", "Set", "Get"}."Set") -> ("error out"=w2122:errorcluster)  [unwired: 9 in, 6 out]
                    n658 = call "Wait till all GFG events stop_for fixed duration.vi"("error in (no error)"=w2122) -> ("error out"=w2117:errorcluster)  [unwired: 10 in]
                  }
                }
              }
              frame "2D.Line.Scan" {
                # "Line"
                n659 = call "Manage UI and GFG states during settings file edit.vi"("Commands"=Update_Scan_Settings_Commands."Initiate Update", "Error In"=w2131, "Command String IN"=w2132, "UI control refnums"=w2128) -> ("Error Out"=w2129:errorcluster)  [unwired: 7 in]
                n660 = call "GFGbooleanGet.vi"("Variable Name in"="Preview.Mode") -> ()  [unwired: 9 in, 2 out]
                n661 = case shown="True" TRUE {
                  tunnel: w2129 -> [w2135 w2137]
                  tunnel: [w2135 w2136] -> w2125
                  frame False {
                  }
                  frame True {
                    n662 = call "Wait till all GFG events stop_for fixed duration.vi"("error in (no error)"=w2137) -> ("error out"=w2138:errorcluster)  [unwired: 10 in]
                    n663 = call "GFG_core.vi"("Variable Name in"="scan.mode.main.settings", "Variant in"=scan_mode_main_settings_tab."2D frame" ("scan mode main settings"), "error in (no error)"=w2138, "Action"=enum16{"Init", "Set", "Get"}."Set") -> ("error out"=w2139:errorcluster)  [unwired: 9 in, 6 out]
                    n664 = call "Wait till all GFG events stop_for fixed duration.vi"("error in (no error)"=w2139) -> ("error out"=w2136:errorcluster)  [unwired: 10 in]
                  }
                }
                n665 = call "Dynamically Call_Settings Info dialog VI.vi"("error in (no error)"=w2125, "Setting File Type"=w2126) -> ("error out"=w2124:errorcluster)  [unwired: 9 in]
              }
              frame "LOOP.Start" {
                # "LOOP.Start"
                n666 = call "Dialog_Enter Loop Iterations.vi"("Error In"=w2147) -> ("Error Out"=w2146:errorcluster, "Cancelled?"=w2145:bool, "Macro Command"=w2144:string)  [unwired: 8 in]
              }
            }
            n667 = case shown="False" w1891 {
              tunnel: w1892 -> [w1908 w1950]
              tunnel: w1876 -> [w1893 w1951]
              tunnel: [w1909 w1947] -> w1874
              tunnel: w1890 -> [w1914 _]
              tunnel: w1870 -> [w1900 _]
              tunnel: [w1905 w1946] -> w1888
              tunnel: w1889 -> [_ w1946]
              tunnel: w1870 -> [w1906 w1952]
              tunnel: [w1906 w1952] -> w1884
              tunnel: w1873 -> [_ w1945]
              tunnel: [TRUE ("Any Error?") w1945] -> w1872
              frame False {
                # "Update params in tree"
                # "Preview mode?"
                n668 = Unbundle By Name(w1893) -> ("Params Table"=w1915:refnum<vi>, "Created Macro"=w1898:refnum<vi>)
                n669 = call "FGV_MacroCore.vi"("Final Index"=w1900, "MacroFGV_Commands"=FGV_MacroCore_Commands."Edit Parameter String", "Error In"=w1908, "Start Index"=w1900, "Macro Command or Info (String)"=w1914) -> ("Error Out"=w1895:errorcluster, "Macro String Array"=w1902:string[])  [unwired: 2 in, 3 out]
                n670 = disable-structure shown="Disabled" {
                  disable-tunnel: w1915 -> [w1922 _]
                  disable-tunnel: w1895 -> [w1921 _]
                  disable-tunnel: [w1918 _] -> w1912
                  disable-tunnel: w1902 -> [w1917 _]
                  frame Disabled {
                    n671 = call "Macro_Text Array to Instruction and Argument array.vi"("Error In"=w1921, "Macro Array IN"=w1917) -> ("Error Out"=w1920:errorcluster, "Argument List (Txt)"=w1919:string[])  [unwired: 7 in, 1 out]
                    n672 = Build Array(w1919) -> (w1925:string[][])
                    n673 = Transpose 2D Array(2D array=w1925) -> (transposed array=w1926:string[][])
                    n674 = property class="Tbl (strict)"(reference=w1922, error in=w1920, "Value"=w1926) -> (reference out=w1924:refnum<vi>, error out=w1923:errorcluster)
                    n675 = Close Reference(reference=w1924, error in (no error)=w1923) -> (error out=w1918:errorcluster)
                  }
                  frame Enabled {
                  }
                }
                n676 = call "Tree_GetTag FromIndex.vi"("Error In"=w1895, "Index IN"=w1900, "Tree Refnum IN"=w1898) -> ("Error Out"=w1896:errorcluster, "Tag OUT"=w1897:string, "Tree Refnum OUT"=w1899:refnum<vi>)  [unwired: 6 in]
                n677 = Index Array(array=w1902, index=w1900) -> (element=w1901:string)
                n678 = call "TimingEstimate_Valid_Invalid_Update.vi"("Command"=enum16{"Valid", "Invalid"}."Invalid", "UI control refnums"=w1893) -> ()  [unwired: 9 in, 1 out]
                n679 = call "Tree_SetText_at_specified_Tag.vi"("Error In"=w1896, "New String IN"=w1901, "Tag (whose string to be edited)"=w1897, "Tree Refnum IN"=w1899) -> ()  [unwired: 6 in, 2 out]
                n680 = call "SavedStatusUpdate.vi"("Options"=enum16{"Unsaved", "Saved"}."Unsaved", "UI control refnums"=w1893) -> ()  [unwired: 9 in, 1 out]
                n681 = call "GFGbooleanGet.vi"("Variable Name in"="Preview.Mode") -> ("Boolean Value OUT"=w1910:bool)  [unwired: 9 in, 1 out]
                n682 = call "MacroExecution and Timing.vi"("MacroExecution and Timing Command"=Macro_Execution_and_Timing_Commands."Update Macro array (Idx Unchanged)", "Error In"=w1912, "Macro IN"=w1902) -> ("Error Out"=w1907:errorcluster)  [unwired: 3 in, 5 out]
                n683 = case shown="False" w1910 {
                  tunnel: [w1928 w1944] -> w1909
                  tunnel: w1907 -> [w1931 w1943]
                  tunnel: w1893 -> [w1929 w1941]
                  tunnel: [w1927 w1940] -> w1905
                  frame False {
                    n684 = call "Macro Debugger.vi"("Error In"=w1931, "UI control refnums"=w1929) -> ("Error Out"=w1930:errorcluster, "Any Error?"=w1927:bool)  [unwired: 8 in]
                    n685 = disable-structure shown="Enabled" {
                      disable-tunnel: w1930 -> [w1935 w1936]
                      disable-tunnel: w1929 -> [w1934 _]
                      disable-tunnel: [w1933 w1936] -> w1928
                      disable-tunnel: w1927 -> [w1932 _]
                      frame Disabled {
                        n686 = call "MacroTiming_Update.vi"("error in (no error)"=w1935, "UI control refnums"=w1934, "Macro Error IN?"=w1932) -> ("error out"=w1933:errorcluster)  [unwired: 8 in]
                      }
                      frame Enabled {
                      }
                    }
                  }
                  frame True {
                    # "This variable is listned to in the Ops Manager. It is used during Preview for actions which do not involve a settings\nfile (like Move.To.Position)"
                    n687 = call "Macro Debugger.vi"("Error In"=w1943, "UI control refnums"=w1941) -> ("Error Out"=w1942:errorcluster, "Any Error?"=w1940:bool)  [unwired: 8 in]
                    n688 = call "GFG_core.vi"("Variable Name in"="Settings.Confirmed", "Variant in"=TRUE, "error in (no error)"=w1942, "Action"=enum16{"Init", "Set", "Get", "Clear"}."Set") -> ("error out"=w1944:errorcluster)  [unwired: 9 in, 6 out]
                  }
                }
              }
              frame True {
                # "Preview mode?"
                # "Cancelled or  Command requires no parameter string modification"
                n689 = call "GFGbooleanGet.vi"("Variable Name in"="Preview.Mode") -> ("Boolean Value OUT"=w1948:bool)  [unwired: 9 in, 1 out]
                n690 = case shown="False" w1948 {
                  tunnel: [w1954 w1967] -> w1947
                  tunnel: w1950 -> [w1957 w1966]
                  tunnel: w1951 -> [w1955 w1964]
                  tunnel: [w1953 w1963] -> _
                  frame False {
                    n691 = call "Macro Debugger.vi"("Error In"=w1957, "UI control refnums"=w1955) -> ("Error Out"=w1956:errorcluster, "Any Error?"=w1953:bool)  [unwired: 8 in]
                    n692 = disable-structure shown="Enabled" {
                      disable-tunnel: w1956 -> [w1961 w1962]
                      disable-tunnel: w1955 -> [w1960 _]
                      disable-tunnel: [w1959 w1962] -> w1954
                      disable-tunnel: w1953 -> [w1958 _]
                      frame Disabled {
                        n693 = call "MacroTiming_Update.vi"("error in (no error)"=w1961, "UI control refnums"=w1960, "Macro Error IN?"=w1958) -> ("error out"=w1959:errorcluster)  [unwired: 8 in]
                      }
                      frame Enabled {
                      }
                    }
                  }
                  frame True {
                    # "This variable is listned to in the Ops Manager. It is used during Preview for actions which do not involve a settings\nfile (like Move.To.Position)"
                    n694 = disable-structure shown="Enabled" {
                      disable-tunnel: w1966 -> [w1971 w1972]
                      disable-tunnel: [w1970 w1972] -> w1965
                      disable-tunnel: w1964 -> [w1969 _]
                      disable-tunnel: [w1968 _] -> w1963
                      frame Disabled {
                        n695 = call "Macro Debugger.vi"("Error In"=w1971, "UI control refnums"=w1969) -> ("Error Out"=w1970:errorcluster, "Any Error?"=w1968:bool)  [unwired: 8 in]
                      }
                      frame Enabled {
                      }
                    }
                    n696 = disable-structure shown="Disabled" {
                      disable-tunnel: [w1974 w1978] -> w1967
                      disable-tunnel: w1965 -> [w1973 w1978]
                      frame Disabled {
                        n697 = call "GFG_core.vi"("Variable Name in"="Settings.Confirmed", "Variant in"=TRUE, "error in (no error)"=w1973, "Action"=enum16{"Init", "Set", "Get", "Clear"}."Set") -> ("error out"=w1974:errorcluster)  [unwired: 9 in, 6 out]
                      }
                      frame Enabled {
                      }
                    }
                  }
                }
              }
            }
          }
          frame True {
            # "DONOT popup message if 'Edit Pressed' as part of a Preview"
            n698 = call "GFGbooleanGet.vi"("Variable Name in"="Preview.Mode") -> ("Boolean Value OUT"=w2148:bool)  [unwired: 9 in, 1 out]
            n699 = case shown="False" w2148 {
              frame False {
                n700 = call "Dialog_Cannot Edit preset element_Popup.vi"() -> ()  [unwired: 11 in, 1 out]
              }
              frame True {
              }
            }
          }
        }
        n701 = Not(x="Edit Parameters") -> (.not. x?=w1839:T5)
        n702 = local write "Edit Parameters"(w1839) -> ()
        n703 = call "reg unreg for MacroGUI.vi"("T for reg, F for unreg"=TRUE, "error in (no error)"=w1854, "event cluster"=w1850, "Event Registration Refnum"=w1851) -> ("error out"=w1853:errorcluster, "Event Registration Refnum Out"=w1852:refnum<event-registration>)  [unwired: 6 in]
      }
      event "Refresh Timing": Value Change {
        n704 = event-data() -> ()  [unwired: 1 in, 1 out]
        n705 = call <vilib>:"Create Cursor From File.vi"("error in (no error)"=w2159, "cursor file"=w2160) -> ("error out"=w2163:errorcluster, "cursor ID"=w2162:refnum<k1>)  [unwired: 8 in]
        n706 = call <vilib>:"Set Busy.vi"("error in (no error)"=w2163, "cursor ID"=w2162) -> ("error out"=w2161:errorcluster)  [unwired: 8 in, 1 out]
        n707 = call "MacroTiming_Update.vi"("error in (no error)"=w2161, "UI control refnums"=w2154, "Macro Error IN?"=w2164) -> ("error out"=w2156:errorcluster)  [unwired: 8 in]
        n708 = call "TimingEstimate_Valid_Invalid_Update.vi"("Command"=enum16{"Valid", "Invalid"}."Valid", "error in (no error)"=w2156, "UI control refnums"=w2154) -> ("error out"=w2155:errorcluster)  [unwired: 8 in]
        n709 = call <vilib>:"Unset Busy.vi"("error in (no error)"=w2155) -> ("error out"=w2158:errorcluster)  [unwired: 10 in]
      }
      event Value Change {
        # "Added to cater for changes in lineScan configuration - \nMove back to 2D frame tab to undo modifications to frame scan settings (which gtes modified to cater for lines)"
        # "Unsaved changes!"
        # "Make sure EDIT is done!"
        n710 = event-data() -> ()  [unwired: 1 in, 1 out]
        n711 = call "FGV_MacroCore.vi"("MacroFGV_Commands"=FGV_MacroCore_Commands."Get Array", "Error In"=w2177) -> ("Error Out"=w2192:errorcluster, "Macro String Array"=w2194:string[])  [unwired: 5 in, 3 out]
        n712 = Index Array(array=w2194, index=w2182) -> (element=w2193:string)
        n713 = call "Decompose Command String.vi"("Error In"=w2192, "Command IN"=w2193) -> ("Error Out"=w2187:errorcluster, "Action"=w2186:string)  [unwired: 6 in, 2 out]
        n714 = call "Macro Action String to Action and Settings Enum.vi"("error in (no error)"=w2187, "Action String IN"=w2186) -> ("error out"=w2175:errorcluster, "Action Enum OUT"=w2178:T49)  [unwired: 6 in, 2 out]
        n715 = case shown="\"2D.Line.Scan\"" w2178 {
          tunnel: w2175 -> [w2209 w2212]
          tunnel: [w2209 w2210] -> w2174
          frame Default {
          }
          frame "2D.Line.Scan" {
            n716 = call "GFG_core.vi"("Variable Name in"="scan.mode.main.settings", "Variant in"=scan_mode_main_settings_tab."2D frame" ("scan mode main settings"), "error in (no error)"=w2212, "Action"=enum16{"Init", "Set", "Get"}."Set") -> ("error out"=w2215:errorcluster)  [unwired: 9 in, 6 out]
            n717 = call "Wait till all GFG events stop_for fixed duration.vi"("error in (no error)"=w2215) -> ("error out"=w2210:errorcluster)  [unwired: 10 in]
          }
        }
        n718 = call "Manage UI and GFG states during settings file edit.vi"("Commands"=Update_Scan_Settings_Commands."Finalise Update", "Error In"=w2174, "UI control refnums"=w2181) -> ("Error Out"=w2199:errorcluster)  [unwired: 8 in]
        n719 = call "FGV_MacroCore.vi"("Final Index"=w2182, "MacroFGV_Commands"=FGV_MacroCore_Commands."Edit Settings File", "Error In"=w2199, "Start Index"=w2182) -> ("Error Out"=w2180:errorcluster)  [unwired: 3 in, 4 out]
        n720 = call "GFG_core.vi"("Variable Name in"="Settings.Confirmed", "Variant in"=TRUE, "error in (no error)"=w2180, "Action"=enum16{"Init", "Set", "Get", "Clear"}."Set") -> ("error out"=w2176:errorcluster)  [unwired: 9 in, 6 out]
        n721 = case shown="\"2D.Line.Scan\"" w2178 {
          tunnel: w2176 -> [w2235 w2239]
          tunnel: [w2232 w2239] -> w2191
          frame "2D.Line.Scan" {
            # "Change Tab - else error\nif focus pressed again\n(It tries to take Line scan)"
            n722 = call "Draw ROI on Line Scan Display.vi"("Draw ROI on Line Scan Display_Command"=Draw_ROI_on_Line_Scan_Display_Command."Clear ROI", "error in (no error)"=w2235) -> ("error out"=w2230:errorcluster)  [unwired: 9 in]
            n723 = call "Wait till all GFG events stop_for fixed duration.vi"("error in (no error)"=w2230) -> ("error out"=w2231:errorcluster)  [unwired: 10 in]
            n724 = call "GFG_core.vi"("Variable Name in"="scan.mode.main.settings", "Variant in"=scan_mode_main_settings_tab."2D frame" ("scan mode main settings"), "error in (no error)"=w2231, "Action"=enum16{"Init", "Set", "Get"}."Set") -> ("error out"=w2233:errorcluster)  [unwired: 9 in, 6 out]
            n725 = call "Wait till all GFG events stop_for fixed duration.vi"("error in (no error)"=w2233) -> ("error out"=w2232:errorcluster)  [unwired: 10 in]
          }
          frame Default {
          }
        }
        n726 = call "GFGbooleanGet.vi"("Variable Name in"="Preview.Mode") -> ("Boolean Value OUT"=w2188:bool)  [unwired: 9 in, 1 out]
        n727 = case shown="False" w2188 {
          tunnel: w2191 -> [w2219 w2224]
          tunnel: w2181 -> [w2218 w2222]
          tunnel: [w2217 w2221] -> w2190
          tunnel: [w2216 w2220] -> w2184
          frame True {
            n728 = call "Macro Debugger.vi"("Error In"=w2219, "UI control refnums"=w2218) -> ("Error Out"=w2216:errorcluster, "Any Error?"=w2217:bool)  [unwired: 8 in]
          }
          frame False {
            n729 = call "Macro Debugger.vi"("Error In"=w2224, "UI control refnums"=w2222) -> ("Error Out"=w2223:errorcluster, "Any Error?"=w2221:bool)  [unwired: 8 in]
            n730 = disable-structure shown="Enabled" {
              disable-tunnel: w2223 -> [w2228 w2229]
              disable-tunnel: w2222 -> [w2227 _]
              disable-tunnel: w2221 -> [w2226 _]
              disable-tunnel: [w2225 w2229] -> w2220
              frame Disabled {
                n731 = call "MacroTiming_Update.vi"("error in (no error)"=w2228, "UI control refnums"=w2227, "Macro Error IN?"=w2226) -> ("error out"=w2225:errorcluster)  [unwired: 8 in]
              }
              frame Enabled {
              }
            }
          }
        }
        n732 = call "SavedStatusUpdate.vi"("Options"=enum16{"Unsaved", "Saved"}."Unsaved", "error in (no error)"=w2184, "UI control refnums"=w2181) -> ("error out"=w2183:errorcluster)  [unwired: 8 in]
      }
      event Value Change {
        # "Get the index where next item needs to be added (ensure its not added in a preset)"
        # "Insert Move.To.Pos commands into FGV,\nupdate UI, and run a debug"
        n733 = event-data() -> ()  [unwired: 1 in, 1 out]
        n734 = Unbundle By Name(w2244) -> ("Created Macro"=w2241:refnum<vi>)
        n735 = call "reg unreg for MacroGUI.vi"("T for reg, F for unreg"=FALSE, "error in (no error)"=w2242, "event cluster"=w2251, "Event Registration Refnum"=w2253) -> ("error out"=w2249:errorcluster, "Event Registration Refnum Out"=w2250:refnum<event-registration>)  [unwired: 6 in]
        n736 = call "Dialog_Load positions from PSM.vi"("error in (no error)"=w2249) -> ("error out"=w2257:errorcluster, "Cancelled or no data?"=w2259:bool, "Move.to.Pos_Cmd Array"=w2258:string[])  [unwired: 8 in]
        n737 = case shown="False" w2259 {
          tunnel: w2258 -> [w2288 _]
          tunnel: [w2267 w2307] -> w2243
          tunnel: w2244 -> [w2285 _]
          tunnel: w2257 -> [w2273 w2309]
          tunnel: w2256 -> [w2287 w2308]
          tunnel: [w2286 w2308] -> w2255
          tunnel: [w2283 w2309] -> w2248
          tunnel: w2241 -> [w2274 _]
          tunnel: w2240 -> [w2271 w2307]
          frame False {
            # "Start index should be atleast 0"
            # "Show dialog if dropped inside a Preset"
            n738 = call "Tree_GetTag FromIndex.vi"("Error In"=w2273, "Index IN"=w2271, "Tree Refnum IN"=w2274) -> ("Error Out"=w2275:errorcluster, "Tag OUT"=w2276:string, "Tree Refnum OUT"=w2277:refnum<vi>)  [unwired: 6 in]
            n739 = call "Check if specified tag is inside a Preset.vi"("error in (no error)"=w2275, "Tag to check"=w2276, "Tree Refnum"=w2277) -> ("error out"=w2278:errorcluster, "Tag to add new item"=w2279:string, "Specified tag is part of a Preset?"=w2281:bool)  [unwired: 5 in, 1 out]
            n740 = case shown="True" w2281 {
              frame False {
              }
              frame True {
                n741 = call "Dialog_Cannot insert PSM commands in the specified position as within a preset_Popup.vi"() -> ()  [unwired: 11 in, 1 out]
              }
            }
            n742 = Empty String/Path?(string/path=w2279) -> (empty?=w2280:bool)
            n743 = case shown="False" w2280 {
              tunnel: w2274 -> [w2293 w2298]
              tunnel: w2279 -> [w2292 _]
              tunnel: w2278 -> [w2291 w2297]
              tunnel: [w2290 w2295] -> w2272
              tunnel: [w2289 w2294] -> w2269
              frame False {
                n744 = call "Tree_GetIndexFromTag.vi"("Error In"=w2291, "Tag IN"=w2292, "Tree Refnum IN"=w2293) -> ("Error Out"=w2290:errorcluster, "Index OUT"=w2289:i32)  [unwired: 6 in, 1 out]
              }
              frame True {
                n745 = call "Tree_GetAll.vi"("Error In"=w2297, "Tree Refnum IN"=w2298) -> ("Error Out"=w2295:errorcluster, "Tags"=w2296:string[])  [unwired: 6 in, 2 out]
                n746 = Array Size(array=w2296) -> (size(s)=w2294:i32)
              }
            }
            n747 = Greater Or Equal To 0?(x=w2269) -> (x >= 0?=w2270:bool)
            n748 = Select(t=w2269, s=w2270, f=0) -> (s? t:f=w2267:i32)
            n749 = for {
              tunnel: w2288 -> [w2302] mode=indexing
              tunnel: [w2303] -> w2282
              tunnel: w2267 -> [w2304]
              shift-right: [w2300] -> w2284
              shift-left: w2272 -> [w2301]
              i -> [w2305]
              n750 = Add(x=w2304, y=w2305) -> (x+y=w2299:i32)
              n751 = call "FGV_MacroCore.vi"("Final Index"=w2299, "MacroFGV_Commands"=FGV_MacroCore_Commands."Insert Item", "Error In"=w2301, "Start Index"=w2299, "Macro Command or Info (String)"=w2302) -> ("Error Out"=w2300:errorcluster, "Macro String Array"=w2303:string[])  [unwired: 2 in, 3 out]
            }
            n752 = call "Display Update During Macro Load.vi"("Macro Error IN"=w2287, "New Index IN"=w2267, "error in (no error)"=w2284, "Macro Array IN"=w2282, "Previous Index IN"=w2267, "UI control refnums"=w2285) -> ("error out"=w2283:errorcluster, "Macro Error OUT"=w2286:bool)  [unwired: 3 in, 1 out]
          }
          frame True {
          }
        }
        n753 = call "reg unreg for MacroGUI.vi"("T for reg, F for unreg"=TRUE, "error in (no error)"=w2248, "event cluster"=w2251, "Event Registration Refnum"=w2250) -> ("error out"=w2246:errorcluster, "Event Registration Refnum Out"=w2247:refnum<event-registration>)  [unwired: 6 in]
      }
      event Value Change {
        # "If 2D LineScan, clear the ROI and change tab to 2D frame scan (to deactivate linescan mode during the next press of focus)"
        # "This GFG is used to signal to\nOps manager than user has \nconfirmed/cancelled the settings."
        # "NO EDIT to settings \nfile is done!"
        n754 = event-data() -> ()  [unwired: 1 in, 6 out]
        n755 = call "Manage UI and GFG states during settings file edit.vi"("Commands"=Update_Scan_Settings_Commands."Finalise Update", "Error In"=w2330, "UI control refnums"=w2325) -> ("Error Out"=w2315:errorcluster)  [unwired: 8 in]
        n756 = call "GFG_core.vi"("Variable Name in"="Settings.Confirmed", "Variant in"=TRUE, "error in (no error)"=w2315, "Action"=enum16{"Init", "Set", "Get", "Clear"}."Set") -> ("error out"=w2324:errorcluster)  [unwired: 9 in, 6 out]
        n757 = call "Macro Debugger.vi"("Error In"=w2324, "UI control refnums"=w2325) -> ("Error Out"=w2321:errorcluster, "Any Error?"=w2323:bool)  [unwired: 8 in]
        n758 = call "FGV_MacroCore.vi"("MacroFGV_Commands"=FGV_MacroCore_Commands."Get Array", "Error In"=w2321) -> ("Error Out"=w2317:errorcluster, "Macro String Array"=w2320:string[])  [unwired: 5 in, 3 out]
        n759 = Index Array(array=w2320, index=w2319) -> (element=w2318:string)
        n760 = call "Decompose Command String.vi"("Error In"=w2317, "Command IN"=w2318) -> ("Error Out"=w2314:errorcluster, "Action"=w2311:string)  [unwired: 6 in, 2 out]
        n761 = call "Macro Action String to Action and Settings Enum.vi"("error in (no error)"=w2314, "Action String IN"=w2311) -> ("error out"=w2313:errorcluster, "Action Enum OUT"=w2312:T49)  [unwired: 6 in, 2 out]
        n762 = case shown="\"2D.Line.Scan\"" w2312 {
          tunnel: w2313 -> [w2343 w2347]
          tunnel: [w2338 w2347] -> w2316
          frame "2D.Line.Scan" {
            # "Change Tab - else error\nif focus pressed again\n(It tries to take Line scan)"
            n763 = call "Draw ROI on Line Scan Display.vi"("Draw ROI on Line Scan Display_Command"=Draw_ROI_on_Line_Scan_Display_Command."Clear ROI", "error in (no error)"=w2343) -> ("error out"=w2340:errorcluster)  [unwired: 9 in]
            n764 = call "Wait till all GFG events stop_for fixed duration.vi"("error in (no error)"=w2340) -> ("error out"=w2339:errorcluster)  [unwired: 10 in]
            n765 = call "GFG_core.vi"("Variable Name in"="scan.mode.main.settings", "Variant in"=scan_mode_main_settings_tab."2D frame" ("scan mode main settings"), "error in (no error)"=w2339, "Action"=enum16{"Init", "Set", "Get"}."Set") -> ("error out"=w2342:errorcluster)  [unwired: 9 in, 6 out]
            n766 = call "Wait till all GFG events stop_for fixed duration.vi"("error in (no error)"=w2342) -> ("error out"=w2338:errorcluster)  [unwired: 10 in]
          }
          frame Default {
          }
        }
      }
      event "stop 2": Value Change {
        n767 = event-data() -> ("NewVal"=w2355:bool)  [unwired: 1 in]
      }
    }
    "Current Index" <- w105
    "Paused/Wait for Trig" <- w97
    "Macro Error?" <- w92
    n768 = call <vilib>:"Simple Error Handler.vi"("error in (no error)"=w81) -> ("error out"=w80:errorcluster)  [unwired: 4 in, 4 out]
    n769 = Wait (ms)(milliseconds to wait=u32 10) -> ()  [unwired: 1 out]
    n770 = Unbundle(w80) -> ("status"=w107:bool)  [unwired: 2 out]
    n771 = Or(x=w107, y=w108) -> (x .or. y?=w93:bool)
    n772 = local write "stop 2"(w93) -> ()
  }
  n773 = while {
    tunnel: w66 -> [w2373]
    tunnel: w15 -> [w2372]
    shift-right: [w2369] -> _
    shift-left: 0 ("Slave Completions Received") -> [w2370]
    tunnel: [w2363] -> w9
    stop <- w2362 stop-if-true
    n774 = call "Heartbeat State Manager.vi"("Heartbeat state manager Input VI names"=w2373, "HB Command Event IN"=w2372) -> ("Error Out"=w2363:errorcluster, "Error conditions Cluster"=→"Error conditions Cluster":T12, "Master-Slave messaging Flags"=w2371:T13, "Heartbeat information cluster"=→"Heartbeat information cluster":T9, "Slave Completions Received"=→"Slave conf received":i32, "Master Instructions Issued"=→"Master instr received":i32)  [unwired: 4 in]
    "Master-Slave messaging Flags" <- w2371
    n775 = Unbundle By Name(w2371) -> ("Slave Ready?"=w2365:bool)
    n776 = feedback-in #2(w2365) -> ()
    n777 = feedback #2() -> (w2368:bool)  [unwired: 1 in]
    n778 = Not(x=w2365) -> (.not. x?=w2364:bool)
    n779 = Not Equal?(x=w2368, y=w2365) -> (x != y?=w2367:bool)
    n780 = And(x=w2367, y=w2364) -> (x .and. y?=w2366:bool)
    n781 = case shown="False" w2366 {
      tunnel: w2370 -> [w2378 w2380]
      tunnel: [w2378 w2379] -> w2369
      frame False {
      }
      frame True {
        n782 = Increment(x=w2380) -> (x+1=w2379:i32)
      }
    }
    "Slave Completions Received" <- w2369
    n783 = Unbundle By Name(w2363) -> ("status"=w2360:bool)
    n784 = Or(x=w2360, y="stop 2") -> (x .or. y?=w2362:bool)
  }
  n785 = call "Clear Specific Errors.vi"("Error In"=w9, "Error number In"=1) -> ("Error Out"=w56:errorcluster)  [unwired: 8 in, 1 out]
  n786 = property on="stop 2" class="Bool (strict)"(error in=w56, "Val(Sgnl)"=TRUE ("Value (Signaling)")) -> (error out=w53:errorcluster)  [unwired: 1 in, 1 out]
  n787 = property on="stop 2" class="Bool (strict)"(error in=w53, "Val(Sgnl)"=FALSE ("stop")) -> (error out=w52:errorcluster)  [unwired: 1 in, 1 out]
  n788 = Merge Errors(w59, w52) -> (w58:errorcluster)
  n789 = call <vilib>:"Simple Error Handler.vi"("error in (no error)"=w58) -> ()  [unwired: 4 in, 5 out]
